vi "Main.vi"() -> ()   [LabVIEW 2015]
doc: "This template is for the Queued Message Handler design pattern.\n\nThe Event Handling Loop generates messages based on user interface actions.\n\nThe Message Handling Loop processes messages generated by the Event Handling Loop, or by other messages. The messages are string values, so new messages can be added easily to the Message Cases case structure in the Message Handling Loop. Each message cluster can also provide an optional value for Message Data, which is a variant that can be converted to whatever message-specific data is required."
uses:
  <vilib>/Utility/miscctls.llb/LV3DPointTypeDef.ctl
  <vilib>/Utility/miscctls.llb/LVRGBAColorTypeDef.ctl
  processedObjectInfo.ctl
  controls/UI Data.ctl
  controls/scanInstrumentInfo.ctl
  controls/Equip_Data.ctl
  controls/startScanData.ctl
  <vilib>/addons/h5labview2/base/hid_t.ctl
  controls/relativeMoveData.ctl
  controls/pBotMessageData.ctl
  controls/currentInfoData.ctl
  <vilib>/addons/h5labview2/file/H5Fmode.ctl
  controls/_acquireScanData_currentState.ctl
  <vilib>/Utility/miscctls.llb/LVPoint32TypeDef.ctl
  <vilib>/Utility/miscctls.llb/LVPointTypeDef.ctl
  <vilib>/Utility/miscctls.llb/LVPositionTypeDef.ctl
  <vilib>/Instr/_visa.llb/VISA Find Search Mode.ctl
  <vilib>/event_ctls.llb/usereventprio.ctl
  support/Message Queue/Enqueue Message (Single).vi
  <vilib>/Instr/_visa.llb/VISA Configure Serial Port (Instr).vi
  <vilib>/addons/h5labview2/base/lib_path.vi
  <vilib>/addons/h5labview2/base/H5Equery.vi
  <vilib>/Utility/error.llb/Error Cluster From Error Code.vi
  <userlib>/_MGI/Application Control/MGI Disable Enum/MGI Disable Enum (Grayed).vi
  <userlib>/_MGI/Application Control/MGI Disable Enum/MGI Disable Enum (Enabled).vi
  flipYZdbl.vi
  flipYZsgl.vi
  <vilib>/Utility/file.llb/Write Delimited Spreadsheet (DBL).vi
  <vilib>/addons/h5labview2/attrib/H5Awrite.llb/H5Awrite.xnode
  <vilib>/addons/h5labview2/dataset/H5Dwrite.llb/H5Dwrite.xnode
  <vilib>/ErrorRing/Error Ring.xnode
  support/Message Queue/Message Queue.lvlib
  support/User Event - Stop/User Event - Stop.lvlib
  <vilib>/picture/3D Picture Control/NI_3D Picture Control.lvlib
  <vilib>/addons/h5labview2/file/H5F.lvlib
  <vilib>/addons/h5labview2/dataset/H5D.lvlib
  <instrlib>/Ocean Optics 2000 4000/Ocean Optics 2000 4000.lvlib
  <vilib>/addons/h5labview2/space/H5S.lvlib
panel:
  out "textColorGray":u32(colorbox)=9174826
  out "textColorRed":u32(colorbox)=9174826
  out "textColorGreen":u32(colorbox)=9174826
  in  "pBot_timeSinceXHome":dbl
  in  "pBot_timeSinceYHome":dbl
  out "emptyObj":T1
  in  "objCol_sel":T2={"Red"=0.0, "Green"=1.0, "Blue"=0.0, "Alpha"=1.0}
  in  "objCol_deSel":T2={"Red"=0.0, "Green"=1.0, "Blue"=0.0, "Alpha"=1.0}
  out "PickPoint":T3
  in  "numberOfCommandLines":i32=50
  in  "cB_dataView":bool
  in  "cB_3Dview":bool
  in  "cB_USB2000+":bool
  in  "cB_plasmaBot":bool
  in  "controlTab":T4(tab)
  in  "pBot_ExperimentTabControl":enum32{"Scan", "Simple Exposure"}(tab)
  in  "pBot_scanNz":u16
  in  "pBot_scanNy":u16
  in  "pBot_scanNx":u16
  in  "pBot_scanningZmax":sgl min=0 step=0.1
  in  "pBot_scanningZmin":sgl caption="Z" min=0 step=0.1
  in  "pBot_scanningYmax":sgl min=0 step=0.1
  in  "pBot_scanningYmin":sgl caption="Y" min=0 step=0.1
  in  "pBot_scanningXmax":sgl min=0 step=0.1
  in  "pBot_scanningXmin":sgl caption="X" min=0 step=0.1
  in  "pBot_scanInstrument":string(combo) caption="Data instrument"
  in  "pBot_runScan":bool
  in  "pBot_yBack1":bool
  in  "pBot_yBack01":bool
  in  "pBot_yBack10":bool
  in  "pBot_xHome":bool
  in  "pBot_xRight1":bool
  in  "pBot_xRight01":bool
  in  "pBot_xRight10":bool
  in  "pBot_xLeft1":bool
  in  "pBot_xLeft10":bool
  in  "pBot_xLeft01":bool
  out "pBot_xyMoveDisplay":string
  in  "pBot_yForward1":bool
  in  "pBot_yForward10":bool
  in  "pBot_yForward01":bool
  in  "pBot_yHome":bool
  in  "pBot_zHome":bool
  out "pBot_zMoveDisplay":string
  in  "pBot_zUp1":bool
  in  "pBot_zUp01":bool
  in  "pBot_zUp10":bool
  in  "pBot_zDown1":bool
  in  "pBot_zDown10":bool
  in  "pBot_zDown01":bool
  in  "pBot_sendCommand":bool
  in  "pBot_gcodeCommand":string caption="G-code command"
  in  "pBot_ConnectButton":bool
  in  "pBot_VISAstrings":string(combo) caption="printrBot Port"
  in  "usb2000p_continuous?":bool caption="Continuous?"
  in  "usb2000p_saveSpectra":bool caption="usb2000p_ConnectButton"
  in  "usb2000p_aquireSpectra":bool caption="usb2000p_ConnectButton"
  in  "usb2000p_ConnectButton":bool
  in  "usb2000p_VISAstrings":string(combo) caption="USB2000+ Port"
  in  "usb2000p_intTime":u32=1000 caption="Integration Time (ms):"
  in  "cB_getObjectInfo":bool caption="Object Information:"
  in  "cB_rotate":bool
  in  "cB_translateDown":bool caption="cB_translateUp"
  in  "cB_translateUp":bool
  in  "cB_translateRight":bool
  in  "cB_translateLeft":bool
  in  "cB_translateForward":bool
  in  "cB_translateBack":bool caption="cB_translateUp"
  in  "cB_revertToActualPos":bool
  in  "cB_visualizeYtrans":dbl(knob) caption="Y" min=0.0 max=150.0 scale=0.0..150.0
  in  "cB_visualizeXtrans":dbl(knob) caption="X" min=0.0 max=285.0 scale=0.0..285.0
  in  "cB_visualizeZtrans":dbl(knob) caption="Z" min=0.0 max=150.0 scale=0.0..150.0
  in  "cB_addObject":bool
  in  "availibleObjectNames":string(combo) caption="Objects availible to add"
  in  "cB_toggleView":bool
  out "cB_realTimeInfoT2":string caption=", T2="
  out "cB_realTimeInfoT1":string caption=", T1="
  out "cB_realTimeInfoZ":string caption=", Z="
  out "cB_realTimeInfoY":string caption=",Y="
  out "cB_realTimeInfoX":string caption="X="
  out "1DdataGraph":cluster{dbl[], dbl[]}(graph)
  out "3D Picture":refnum<vi>(3d-picture)
  out "cB_commandLog":string
  # "(escape to quit  for now)"
  # "Configure the instrument first!!"
  # "Region"
  # "# of points"
  # ":"
  # ":"
  # ":"
  # "Y"
  # "X"
  # "Z"
  # "Use toggleView in the top right to switch between viewing spectra and the  3Dscene."
  # "Translate, rotate, get info of object\n(right click to select)"
  # "Use below knobs to visualize a\ntranslation without actually moving"
  # "dataView"
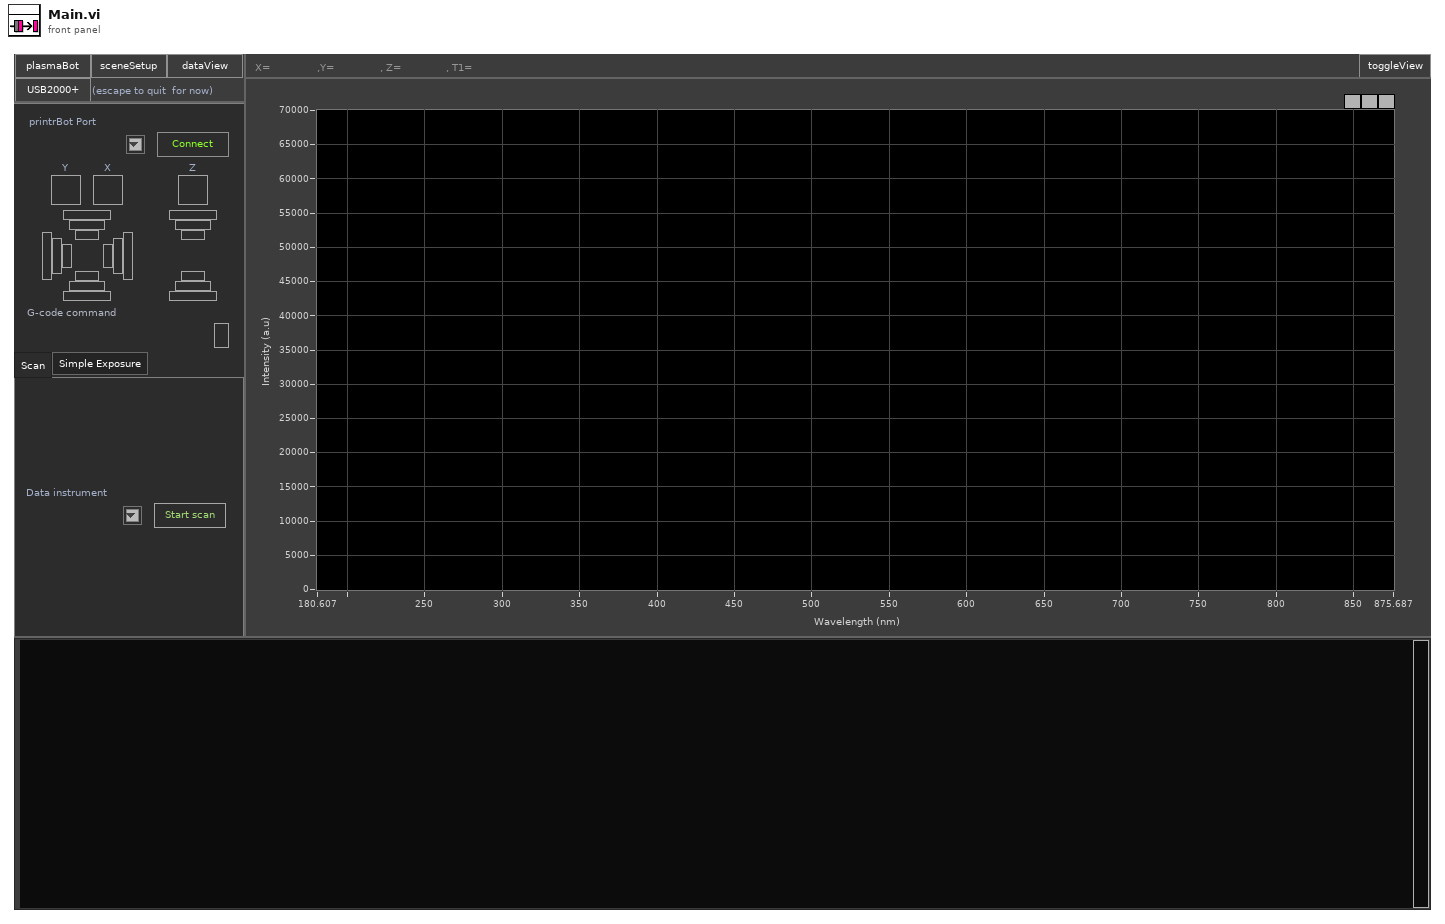
[diagram p1: front panel]
types:
  T1 = typedef "processedObjectInfo.ctl" = cluster{"Name":string, "objectFiles":cluster{"Location":path, "Color":cluster{"R":dbl, "G":dbl, "B":dbl, "A":dbl}}[], "center":cluster{"X":dbl, "Y":dbl, "Z":dbl}, "extent":cluster{"X":dbl, "Y":dbl, "Z":dbl}, "allowedMotion":enum16{"XY", "Z"}, "mountOn":enum16{"yArm", "breadBoard"}, "Movements":cluster{"Type":enum16{"rr", "ra", "tr", "ta"}, "vector":cluster{"X":dbl, "Y":dbl, "Z":dbl}, "scalar":dbl}[], "extraInfo":cluster{"parameter":string, "dataType":string, "vector":cluster{"X":dbl, "Y":dbl, "Z":dbl}, "scalar":dbl}[], "hasPOI?":bool, "POI":cluster{"X":dbl, "Y":dbl, "Z":dbl}, "posOffset":cluster{"X":dbl, "Y":dbl, "Z":dbl}, "referenceNum":refnum<vi>}
  T2 = typedef "LVRGBAColorTypeDef.ctl" = cluster{"Red":sgl, "Green":sgl, "Blue":sgl, "Alpha":sgl}
  T3 = typedef "LV3DPointTypeDef.ctl" = cluster{"X":sgl, "Y":sgl, "Z":sgl}
  T4 = enum32{"plasmaBot", "USB2000+", "3DView", "dataView"}
  T5 = typedef "Equip_Data.ctl" = cluster{"travelRange":T3, "yPOI_0":T3, "yPOI":T3, "pBot_VISA":refnum<visa-resource-name>, "pBotConnected?":bool, "disconnectPBot_Event":refnum<user-event>, "scanData":T6, "scanIndex":cluster{"X":u16, "Y":u16, "Z":u16}, "scanIncrementDir":cluster{"xFwd?":i16, "yFwd?":i16, "zFwd?":i16}, "scanSpeed":u16, "instrDataPage":u16[][][][], "instrDataPageSize":i32[], "h5File_refOut":T8, "ish5FileOpen?":bool, "h5File_dsetOut":T8, "h5FileError":errorcluster, "totalSteps":u32, "currentStep":u32, "USB2000p_Info":T7, "integrationTime":u32, "scan?":bool, "pBot_currentEEPROMsettings":string}
  T6 = typedef "startScanData.ctl" = cluster{"dataFilePath":path, "scanPoints":cluster{"dim1":sgl[], "dim2":sgl[], "dim3":sgl[]}, "N":cluster{"X":u16, "Y":u16, "Z":u16}, "scanInstrumentInfo":T7}
  T7 = typedef "scanInstrumentInfo.ctl" = cluster{"Name":string, "VISAname":refnum<visa-resource-name>, "1D_dataArraySize":u16, "extraInfo":variant, "error":errorcluster}
  T8 = typedef "hid_t.ctl" = i32
  T9 = typedef "UI Data.ctl" = cluster{"controlTabState":bool[], "pathToSTLFiles":path, "availableObjs":T1[], "objectNames":string[], "addedObjs":T1[], "selectedObj":T1, "3DPictureObjRef":refnum<vi>, "yPOI_0":cluster{"X":dbl, "Y":dbl, "Z":dbl}, "yPOI":cluster{"X":dbl, "Y":dbl, "Z":dbl}, "yPOI_Added?":bool, "breadBoard_00":cluster{"X":dbl, "Y":dbl, "Z":dbl}, "breadBoardOriginOffset":cluster{"X":dbl, "Y":dbl, "Z":dbl}, "XYtranslateObjControls":refnum<vi>[], "ZtranslateObjControls":refnum<vi>[], "pBot_controls":refnum<vi>[], "pBot_VISA":refnum<visa-resource-name>, "commandLog":string, "pBotConnected?":bool, "pBot_currentEEPROMsettings":string, "realTimeInfoControls":refnum<vi>[], "pBot_tempSensor1":dbl, "pBot_tempSensor2":dbl, "realTimeInfoTextColor":u32[], "disconnectPBot_Event":refnum<user-event>, "needToHomeY?":bool, "pBot_relativePositioning":bool, "pBot_minPos":cluster{"X":dbl, "Y":dbl, "Z":dbl}, "pBot_maxPos":cluster{"X":dbl, "Y":dbl, "Z":dbl}, "pBot_homeOffset":cluster{"X":dbl, "Y":dbl, "Z":dbl}, "textColorGreen":u32, "textColorRed":u32, "textColorGray":u32, "transVisualizationControls":refnum<vi>[], "needToHomeXY?":bool, "pBot_minScanRegion":cluster{"X":sgl, "Y":sgl, "Z":sgl}, "pBot_maxScanRegion":cluster{"X":sgl, "Y":sgl, "Z":sgl}, "pBot_scanN":cluster{"X":u16, "Y":u16, "Z":u16}, "connectedInstruments":T7[], "isScanning?":bool, "Wavelengths":dbl[], "usb2000p_controlRefs":refnum<vi>[], "3DPictureRef":refnum<vi>}
  T10 = typedef "Message Queue.lvlib/All Message Queues.ctl" = cluster{"UI":refnum<queue>, "equipment":refnum<queue>}
  T11 = cluster{"Message":string, "error constant":errorcluster, "disconnectPBot_Event":refnum<user-event>}
  T12 = typedef "relativeMoveData.ctl" = cluster{"Direction":enum16{"Y", "X", "Z"}, "Amount":dbl}
  T13 = typedef "eventvkey.ctl" = enum16{"ASCII", "Enter", "Return", "Shift", "Ctrl", "Alt", "Cmd", "Opt", "Caps", "NumLock", "Clear", "Break", "Up", "Down", "Left", "Right", "Insert", "Delete", "Home", "End", "PageUp", "PageDown", "Escape", "Help", "Pause", "ScrollLock", "F1", "F2", "F3", "F4", "F5", "F6", "F7", "F8", "F9", "F10", "F11", "F12", "F13", "F14", "F15", "F16", "F17", "F18", "F19", "F20", "F21", "F22", "F23", "F24", "Play", "VolumeUp", "VolumeDown", "Mute", "Two Byte Char"}
  T14 = typedef "LVPoint32TypeDef.ctl" = cluster{"Horizontal":i32, "Vertical":i32}
  T15 = typedef "pBotMessageData.ctl" = cluster{"commandID":string, "gCode":string, "extraInfo":string, "originatingCommandID":string, "error":errorcluster}
  T16 = typedef "currentInfoData.ctl" = cluster{"currentPos":cluster{"X":dbl, "Y":dbl, "Z":dbl}, "temperature":dbl, "error constant":errorcluster}
  T17 = typedef "H5F.lvlib/H5Fmode.ctl" = enum16{"read-only", "read-write", "overwrite", "create new", "open or create"}
  T18 = typedef "_acquireScanData_currentState.ctl" = cluster{"scanIndex":cluster{"X":u16, "Y":u16, "Z":u16}, "scanFinished?":bool, "savePageData?":bool}
  T19 = cluster{"dim1":sgl[], "dim2":sgl[], "dim3":sgl[]}
  T20 = cluster{"cB_visualizeXtrans":dbl, "cB_visualizeZtrans":dbl, "cB_visualizeYtrans":dbl}
  T21 = cluster{"cB_visualizeXtrans":dbl, "cB_visualizeYtrans":dbl, "cB_visualizeZtrans":dbl}
  T22 = enum8{"Enabled", "Disabled", "Disabled and Grayed Out"}
  T23 = typedef "LVPositionTypeDef.ctl" = cluster{"Left":i32, "Top":i32}
  T24 = typedef "LVPointTypeDef.ctl" = cluster{"Horizontal":i16, "Vertical":i16}
  T25 = enum16{"None", "Spherical", "Flying", "Oriented"}
  T26 = typedef "usereventprio.ctl" = enum32{"high priority", "normal priority"}
  T27 = typedef "LVRectTypeDef.ctl" = cluster{"Left":i16, "Top":i16, "Right":i16, "Bottom":i16}
  T28 = typedef "VISA Find Search Mode.ctl" = u32
  T29 = cluster{"Wavelengths":dbl[], "Spectrum by Pixels":dbl[]}
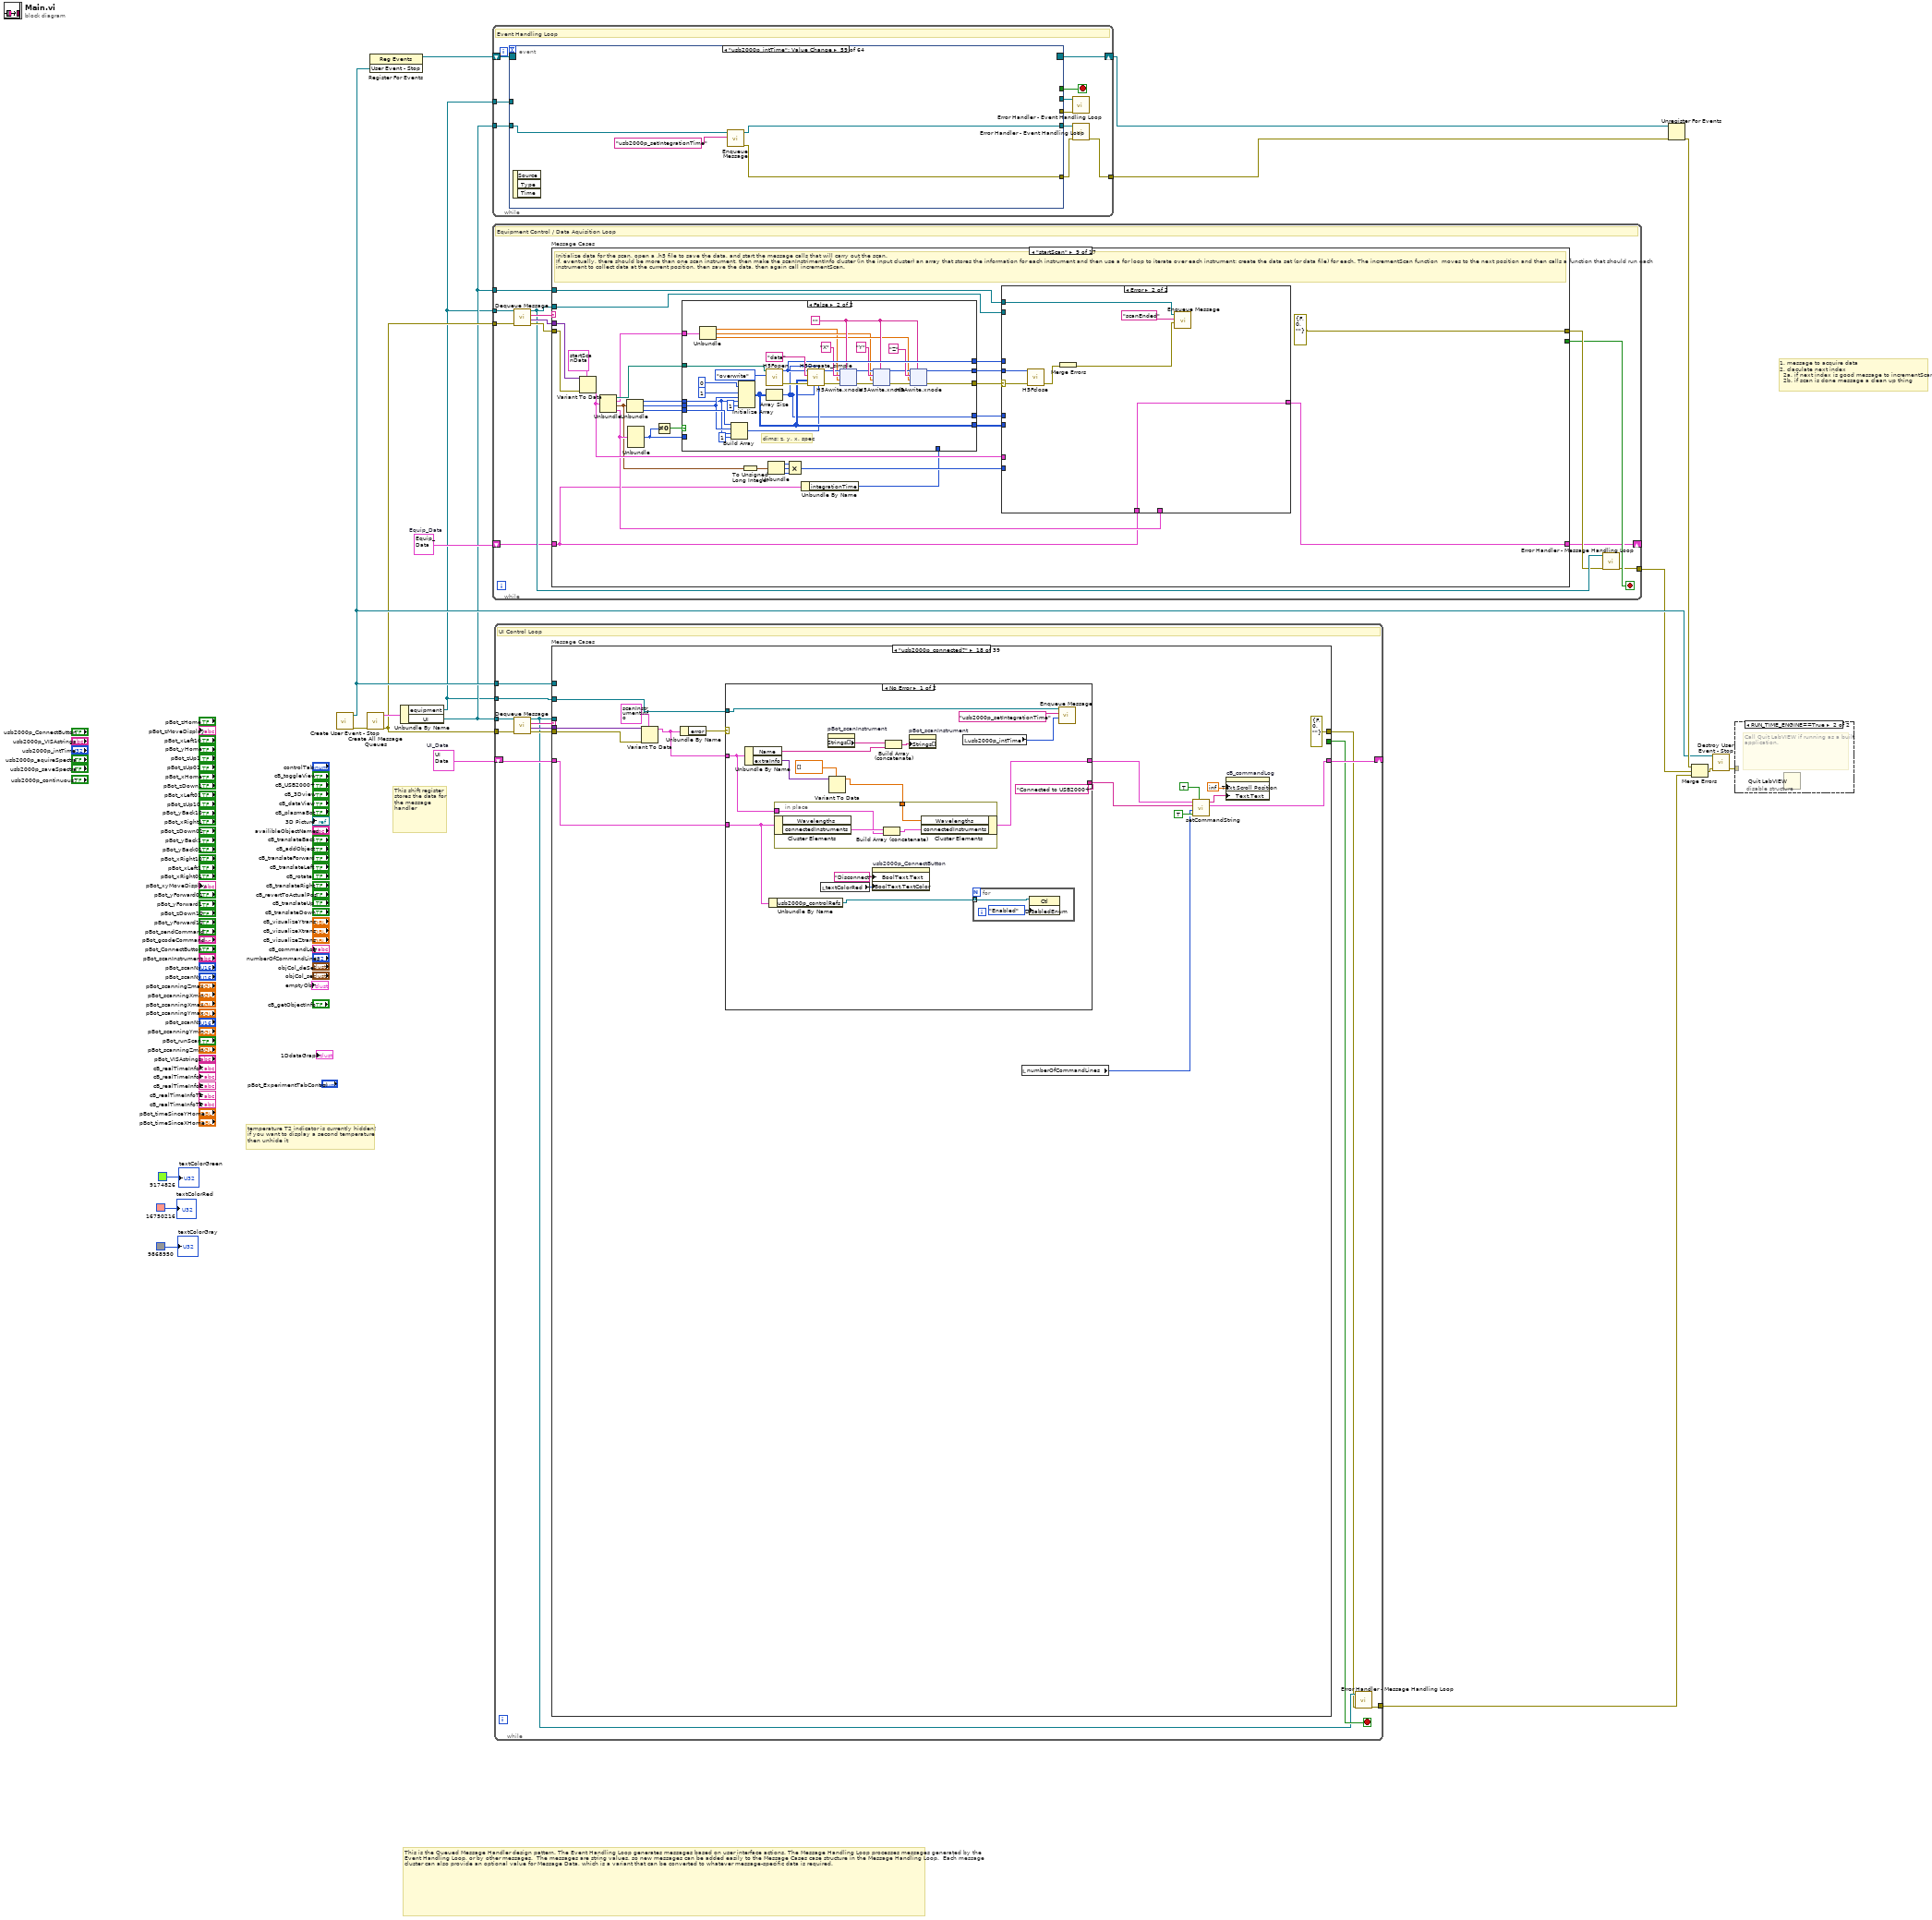
[diagram p0: block diagram]
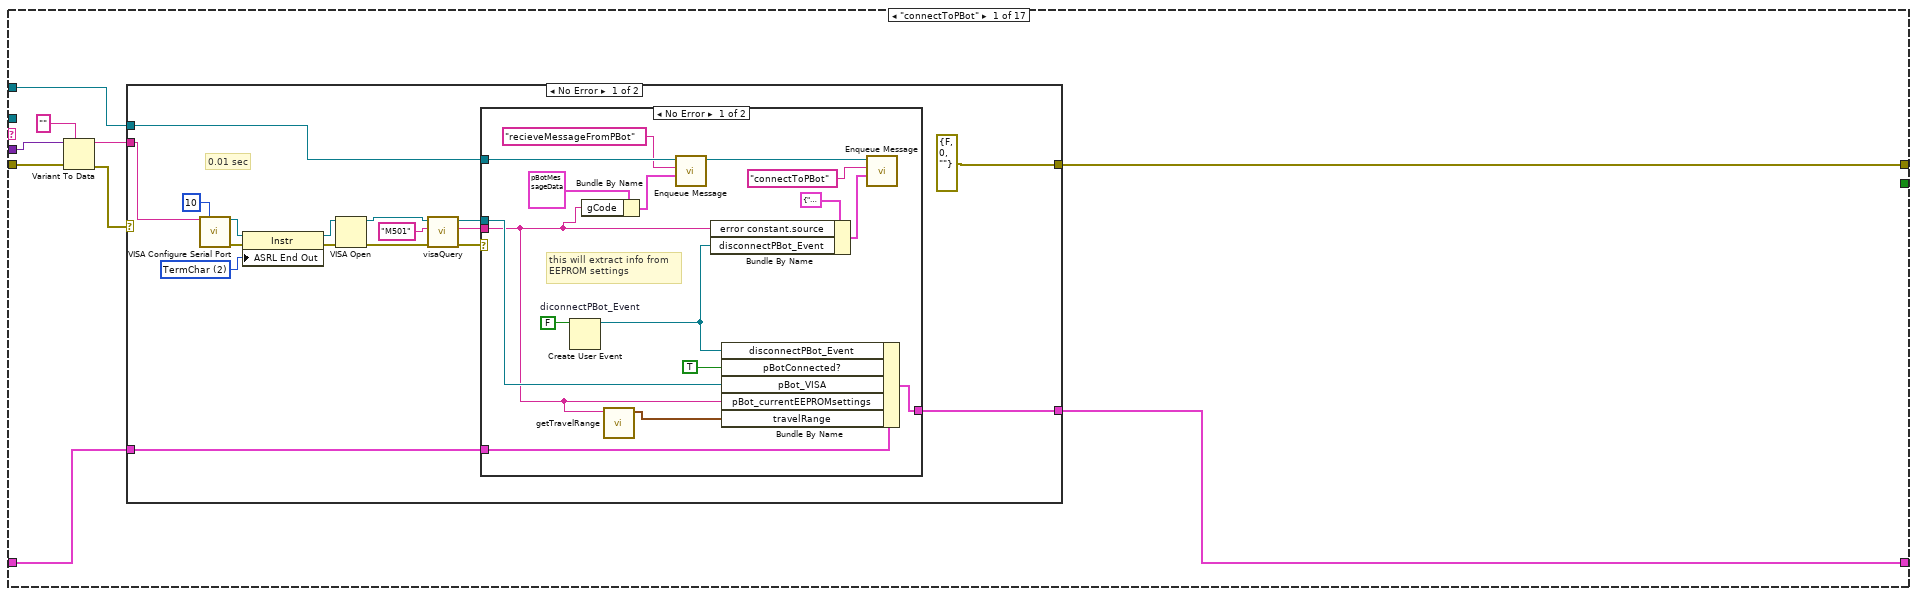
[diagram p2: hidden frame]
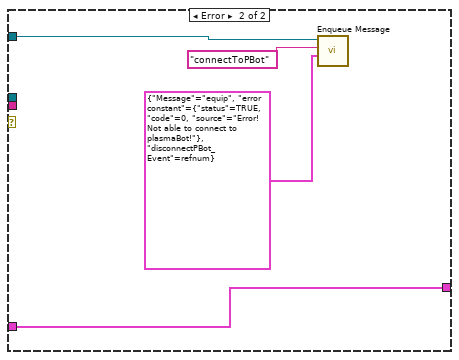
[diagram p3: hidden frame]
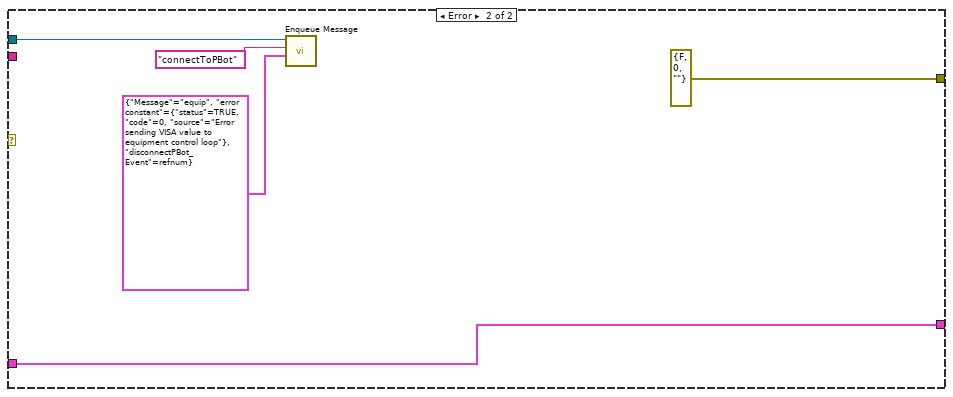
[diagram p4: hidden frame]
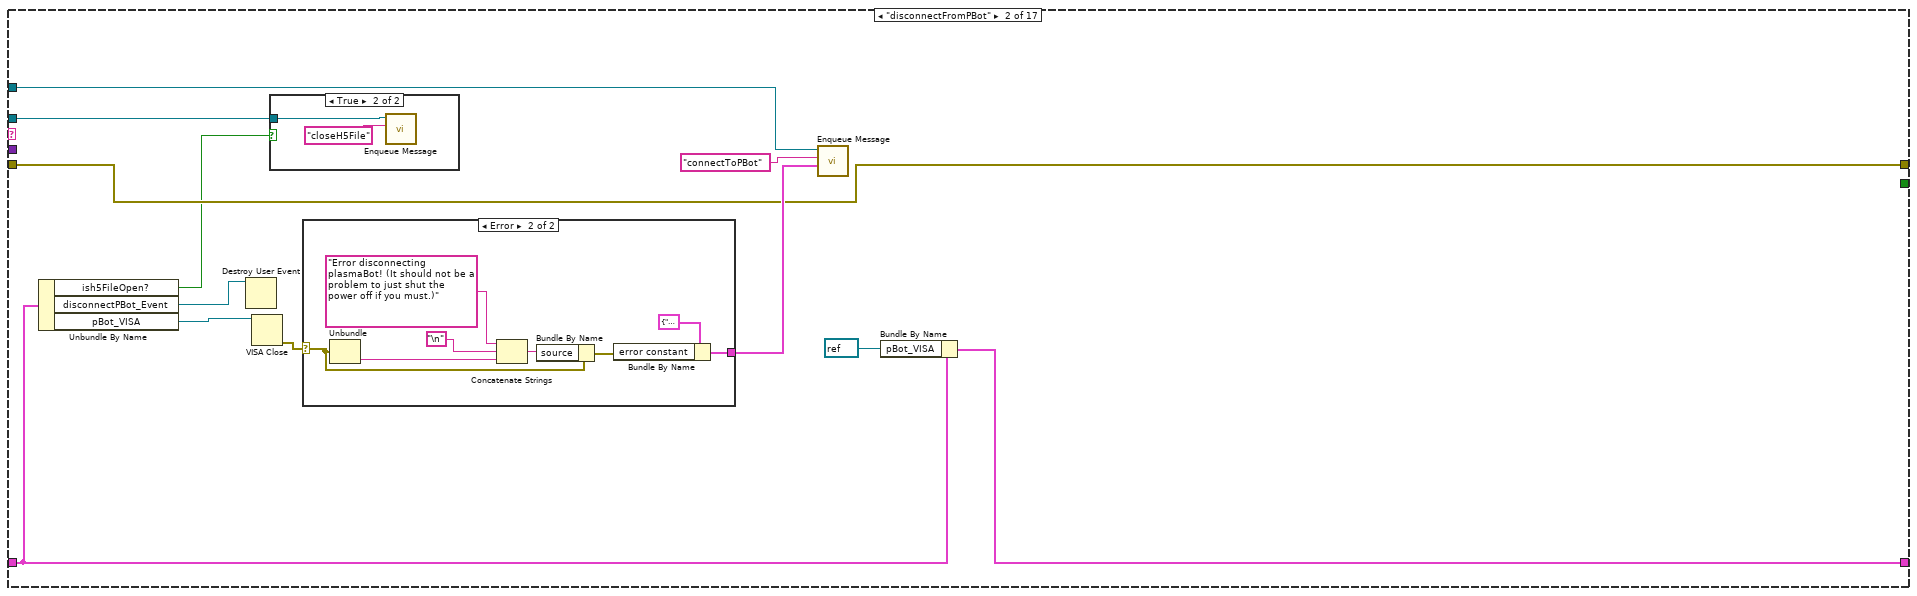
[diagram p5: hidden frame]
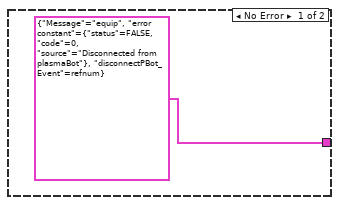
[diagram p7: hidden frame]
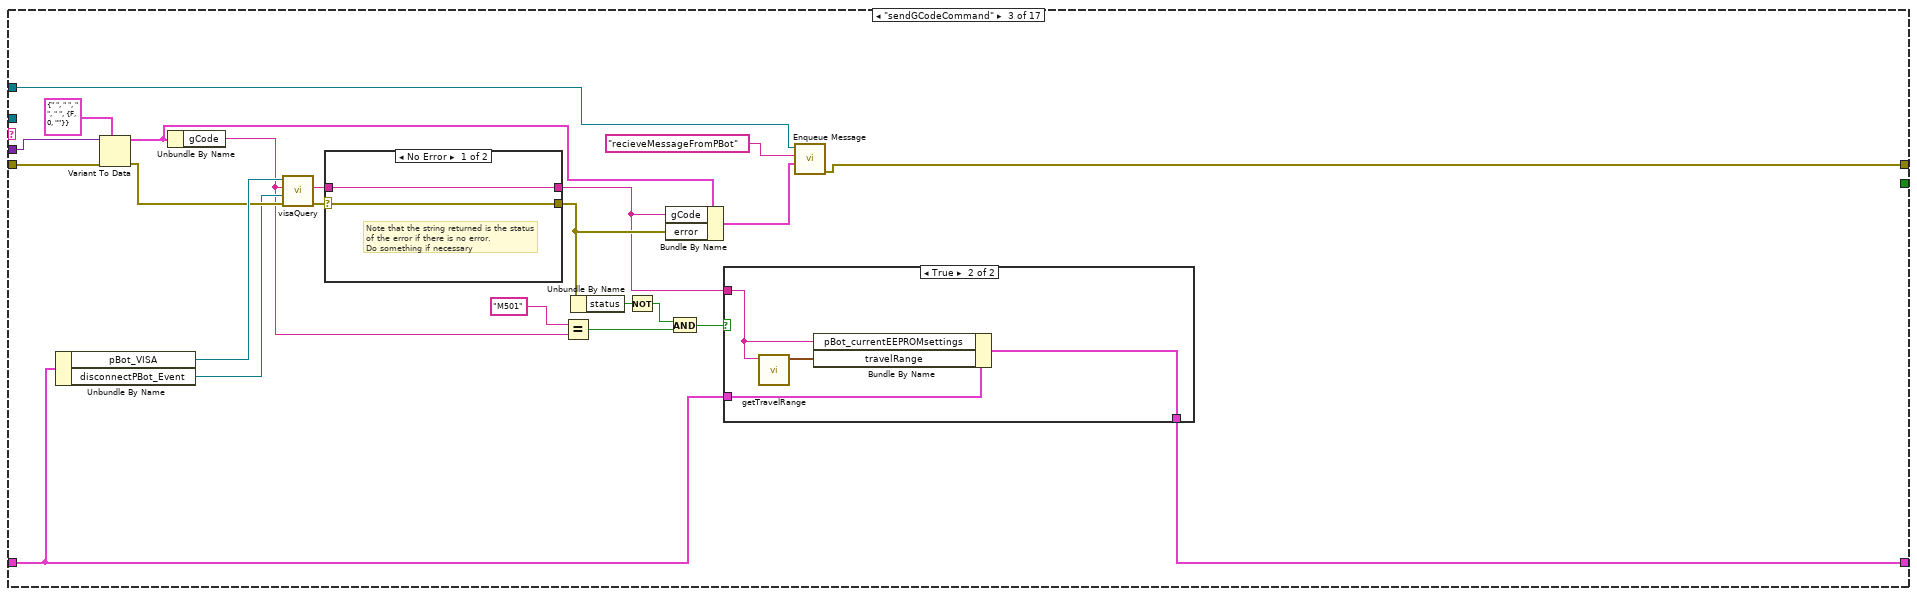
[diagram p8: hidden frame]
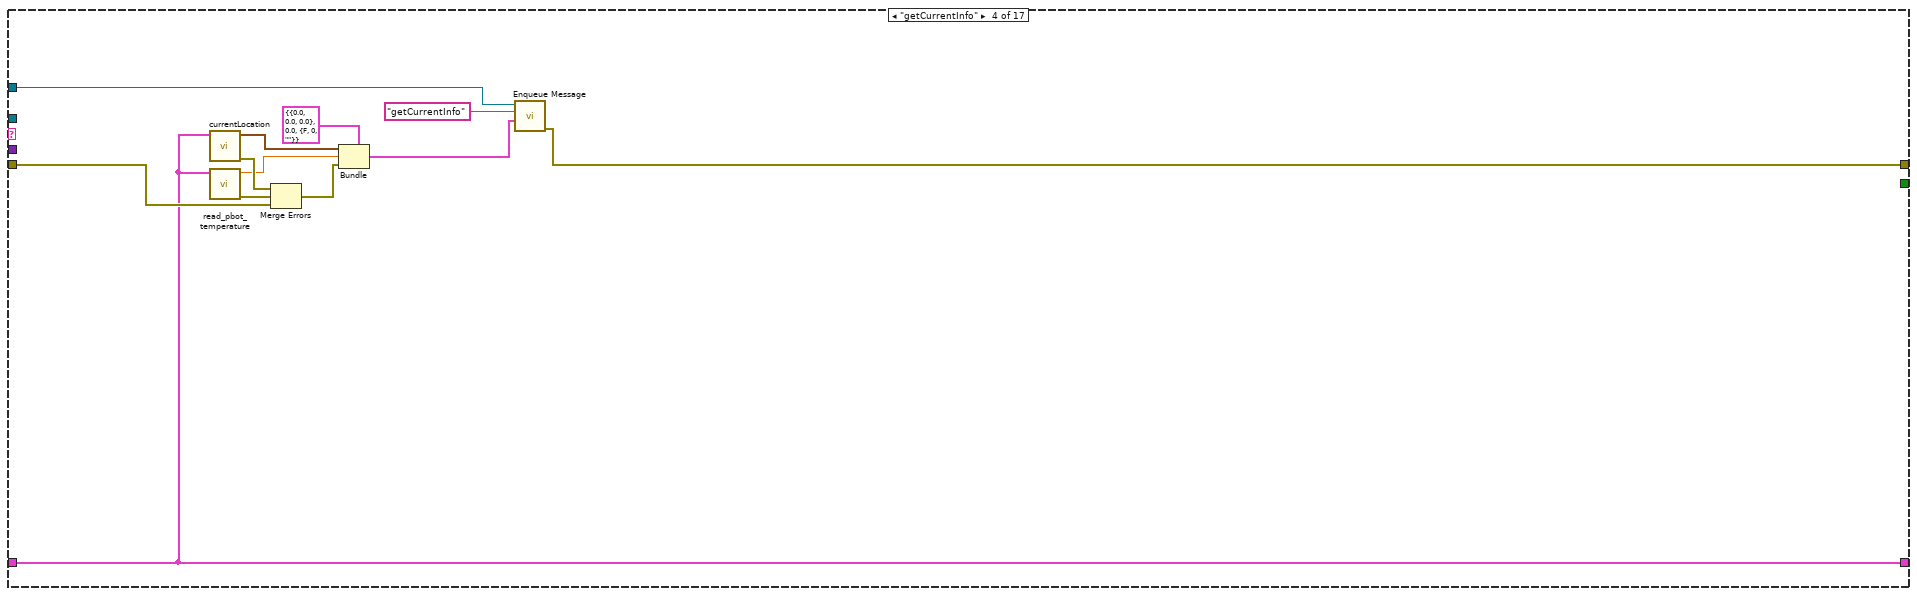
[diagram p11: hidden frame]
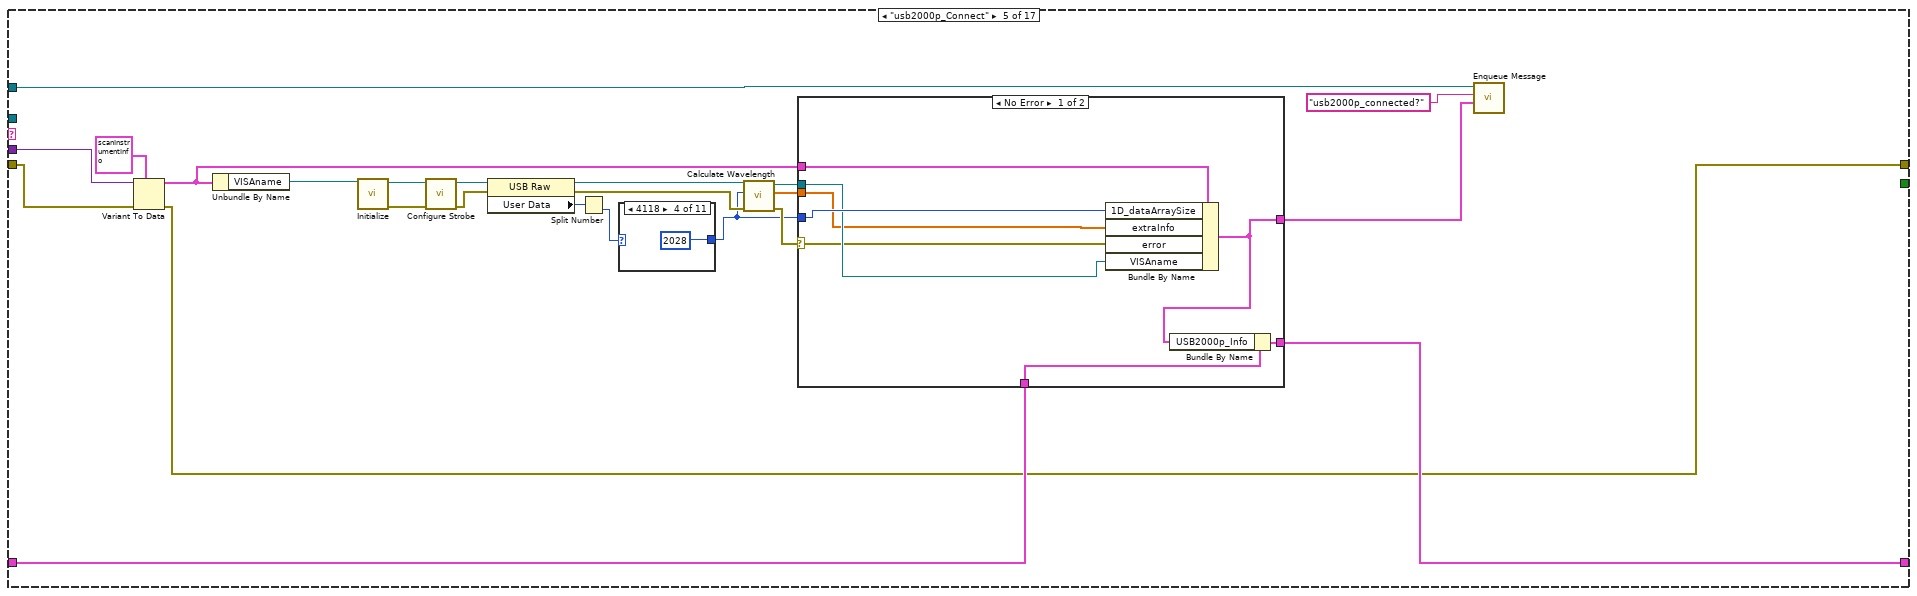
[diagram p12: hidden frame]
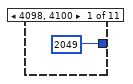
[diagram p13: hidden frame]
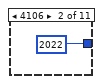
[diagram p14: hidden frame]
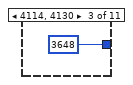
[diagram p15: hidden frame]
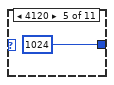
[diagram p16: hidden frame]
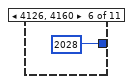
[diagram p17: hidden frame]
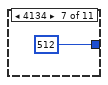
[diagram p18: hidden frame]
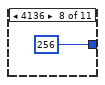
[diagram p19: hidden frame]
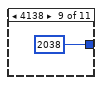
[diagram p20: hidden frame]
diagram:
  w4 = T5 {"travelRange"={"X"=0.0, "Y"=0.0, "Z"=0.0}, "yPOI_0"={"X"=0.0, "Y"=0.0, "Z"=0.0}, "yPOI"={"X"=0.0, "Y"=0.0, "Z"=0.0}, "pBot_VISA"="", "pBotConnected?"=FALSE, "disconnectPBot_Event"=refnum, "scanData"={"dataFilePath"=path "", "scanPoints"={"dim1"=[], "dim2"=[], "dim3"=[]}, "N"={"X"=0, "Y"=0, "Z"=0}, "scanInstrumentInfo"={"Name"="", "VISAname"="", "1D_dataArraySize"=0, "extraInfo"=variant, "error"={"status"=FALSE, "code"=0, "source"=""}}}, "scanIndex"={"X"=0, "Y"=0, "Z"=0}, "scanIncrementDir"={"xFwd?"=0, "yFwd?"=0, "zFwd?"=0}, "scanSpeed"=0, "instrDataPage"=[], "instrDataPageSize"=[], "h5File_refOut"=0, "ish5FileOpen?"=FALSE, "h5File_dsetOut"=0, "h5FileError"={"status"=FALSE, "code"=0, "source"=""}, "totalSteps"=0, "currentStep"=0, "USB2000p_Info"={"Name"="", "VISAname"="", "1D_dataArraySize"=0, "extraInfo"=variant, "error"={"status"=FALSE, "code"=0, "source"=""}}, "integrationTime"=0, "scan?"=FALSE, "pBot_currentEEPROMsettings"=""}  # Equip_Data
  w14 = T9 {"controlTabState"=[], "pathToSTLFiles"=path "", "availableObjs"=[], "objectNames"=[], "addedObjs"=[], "selectedObj"={"Name"="", "objectFiles"=[], "center"={"X"=0.0, "Y"=0.0, "Z"=0.0}, "extent"={"X"=0.0, "Y"=0.0, "Z"=0.0}, "allowedMotion"=enum."XY", "mountOn"=enum."yArm", "Movements"=[], "extraInfo"=[], "hasPOI?"=FALSE, "POI"={"X"=0.0, "Y"=0.0, "Z"=0.0}, "posOffset"={"X"=0.0, "Y"=0.0, "Z"=0.0}, "referenceNum"=refnum}, "3DPictureObjRef"=refnum, "yPOI_0"={"X"=0.0, "Y"=0.0, "Z"=0.0}, "yPOI"={"X"=0.0, "Y"=0.0, "Z"=0.0}, "yPOI_Added?"=FALSE, "breadBoard_00"={"X"=0.0, "Y"=0.0, "Z"=0.0}, "breadBoardOriginOffset"={"X"=0.0, "Y"=0.0, "Z"=0.0}, "XYtranslateObjControls"=[], "ZtranslateObjControls"=[], "pBot_controls"=[], "pBot_VISA"="", "commandLog"="", "pBotConnected?"=FALSE, "pBot_currentEEPROMsettings"="", "realTimeInfoControls"=[], "pBot_tempSensor1"=0.0, "pBot_tempSensor2"=0.0, "realTimeInfoTextColor"=[], "disconnectPBot_Event"=refnum, "needToHomeY?"=FALSE, "pBot_relativePositioning"=FALSE, "pBot_minPos"={"X"=0.0, "Y"=0.0, "Z"=0.0}, "pBot_maxPos"={"X"=0.0, "Y"=0.0, "Z"=0.0}, "pBot_homeOffset"={"X"=0.0, "Y"=0.0, "Z"=0.0}, "textColorGreen"=9174826, "textColorRed"=16750216, "textColorGray"=9868950, "transVisualizationControls"=[], "needToHomeXY?"=FALSE, "pBot_minScanRegion"={"X"=0.0, "Y"=0.0, "Z"=0.0}, "pBot_maxScanRegion"={"X"=0.0, "Y"=0.0, "Z"=0.0}, "pBot_scanN"={"X"=0, "Y"=0, "Z"=0}, "connectedInstruments"=[], "isScanning?"=FALSE, "Wavelengths"=[], "usb2000p_controlRefs"=[], "3DPictureRef"=refnum}  # UI_Data
  # "1. message to acquire data\n2. claculate next index\n  2a. if next index is good message to incrementScan\n  2b. if scan is done message a clean up thing"
  # "temperature T2 indicator is currently hidden!\nif you want to display a second temperature\nthen unhide it"
  # "This is the Queued Message Handler design pattern. The Event Handling Loop generates messages based on user interface actions. The Message Handling Loop processes messages generated by the Event Handling Loop, or by other messages.  The messages are string values, so new messages can be added easily to the Message Cases case structure in the Message Handling Loop.  Each message cluster can also provide an optional value for Message Data, which is a variant that can be converted to whatever message-specific data is required."
  # "This shift register stores the data for the message handler"
  n1 = call "Create User Event - Stop.vi"() -> ("error out"=w18:errorcluster, "User Event - Stop"=w10:refnum<user-event>)  [unwired: 10 in]
  n2 = call "Create All Message Queues.vi"("error in (no error)"=w18) -> ("error out"=w7:errorcluster, "Message Queues out"=w19:T10)  [unwired: 9 in]
  n3 = register-events(w10) -> (reference out=w11:refnum<event-registration>)  [unwired: 2 in, 1 out]
  n4 = Unbundle By Name(w19) -> ("equipment"=w2:refnum<queue>, "UI"=w3:refnum<queue>)
  n5 = while {
    tunnel: w3 -> [w29]
    shift-right: [w27] -> w15
    shift-left: w11 -> [w28]
    tunnel: [w23] -> w12
    tunnel: w2 -> [w22]
    stop <- w25 stop-if-true
    # "Event Handling Loop"
    n6 = event shown="[58] \"usb2000p_intTime\": Value Change" {
      selector: w28 -> [_ _ _ _ _ _ _ _ _ _ _ _ _ _ _ _ _ _ _ _ _ _ _ _ _ _ _ _ _ _ _ _ _ _ _ _ _ _ _ _ _ _ _ _ _ _ _ _ _ _ _ _ _ _ _ _ _ _ _ _ _ _ _ _]
      dyn-events: [_ _ _ _ _ _ _ _ _ _ _ _ _ _ _ _ _ _ _ _ _ _ _ _ _ _ _ _ _ _ _ _ _ _ _ _ _ _ _ _ _ _ _ _ _ _ _ _ _ _ _ _ _ _ _ _ _ _ _ _ _ _ _ _] -> w27
      timeout: _ -> [_ _ _ _ _ _ _ _ _ _ _ _ _ _ _ _ _ _ _ _ _ _ _ _ _ _ _ _ _ _ _ _ _ _ _ _ _ _ _ _ _ _ _ _ _ _ _ _ _ _ _ _ _ _ _ _ _ _ _ _ _ _ _ _]
      tunnel: [_ _ _ _ _ _ _ _ _ _ _ _ _ _ _ _ _ _ _ _ _ _ _ _ _ _ _ _ _ _ _ _ _ _ _ _ _ _ _ _ _ _ _ _ _ _ _ _ _ _ _ _ _ _ _ _ _ _ _ _ _ TRUE ("Discard?") _ _] -> w25
      tunnel: w29 -> [w33 w37 w41 w45 w49 w54 w59 w64 w69 w74 w79 w83 w90 w117 w120 w124 w132 w136 w140 w144 w149 w154 w159 w164 w169 w174 w179 w184 w189 w194 w199 w204 w209 w215 w220 w225 w231 w236 w241 w246 w251 w256 w261 w266 w271 w276 w281 w286 w291 w296 w301 w306 w311 w316 w319 w323 w328 w332 w336 w340 w344 w346 w351 w353]
      tunnel: [w31 w34 w38 w42 w46 w50 w55 w60 w65 w70 w75 w80 w87 _ _ _ _ _ w138 w142 w147 w152 w157 w162 w167 w172 w177 w182 w187 w192 w197 w202 w207 w213 w218 w223 w227 w232 w237 w242 w247 w252 w257 w262 w267 w272 w277 w282 w287 w292 w297 w302 w307 w312 w317 w321 w326 w330 w334 w338 w342 _ w350 _] -> w26
      tunnel: [w32 w36 w40 w44 w48 w53 w58 w63 w68 w73 w78 w82 w89 w116 w119 w123 w131 w135 w139 w143 w148 w153 w158 w163 w168 w173 w178 w183 w188 w193 w198 w203 w208 w214 w219 w224 w228 w233 w238 w243 w248 w253 w258 w263 w268 w273 w278 w283 w288 w293 w298 w303 w308 w313 w318 w322 w327 w331 w335 w339 w343 w346 w349 w353] -> w24
      tunnel: w22 -> [_ _ _ _ _ _ _ _ _ _ _ _ w86 _ _ _ _ _ _ _ _ _ _ _ _ _ _ _ _ _ _ _ _ _ _ _ _ _ _ _ _ _ _ _ _ _ _ _ _ _ _ _ _ _ _ _ _ _ _ _ _ _ _ _]
      tunnel: [_ _ _ _ _ _ _ _ _ _ _ _ w85 _ _ _ _ _ _ _ _ _ _ _ _ _ _ _ _ _ _ _ _ _ _ _ _ _ _ _ _ _ _ _ _ _ _ _ _ _ _ _ _ _ _ _ _ _ _ _ _ _ _ _] -> w21
      tunnel: [_ _ _ _ _ _ _ _ _ _ _ _ w84 _ _ _ _ _ _ _ _ _ _ _ _ _ _ _ _ _ _ _ _ _ _ _ _ _ _ _ _ _ _ _ _ _ _ _ _ _ _ _ _ _ _ _ _ _ _ _ _ _ _ _] -> w20
      event Pane Size {
        n7 = event-data() -> ()  [unwired: 1 in, 1 out]
        n8 = call-poly "Enqueue Message.vi"("Message"="updateDisplay", "Message Queue"=w33) -> ("error out"=w31:errorcluster, "dup Message Queue"=w32:refnum<queue>)  [unwired: 8 in]
      }
      event "cB_dataView", "cB_3Dview", "cB_USB2000+", "cB_plasmaBot": Value Change {
        n9 = event-data() -> ()  [unwired: 1 in, 6 out]
        n10 = call-poly "Enqueue Message.vi"("Message"="changeControlTab", "Message Queue"=w37) -> ("error out"=w34:errorcluster, "dup Message Queue"=w36:refnum<queue>)  [unwired: 8 in]
      }
      event "cB_toggleView": Value Change {
        n11 = event-data() -> ()  [unwired: 1 in, 6 out]
        n12 = call-poly "Enqueue Message.vi"("Message"="toggleView", "Message Queue"=w41) -> ("error out"=w38:errorcluster, "dup Message Queue"=w40:refnum<queue>)  [unwired: 8 in]
      }
      event "cB_addObject": Value Change {
        n13 = event-data() -> ()  [unwired: 1 in, 1 out]
        n14 = call-poly "Enqueue Message.vi"("Message"="addObject", "Message Queue"=w45) -> ("error out"=w42:errorcluster, "dup Message Queue"=w44:refnum<queue>)  [unwired: 8 in]
      }
      event "cB_rotate": Value Change {
        n15 = event-data() -> ()  [unwired: 1 in, 1 out]
        n16 = call-poly "Enqueue Message.vi"("Message"="rotateObject", "Message Queue"=w49) -> ("error out"=w46:errorcluster, "dup Message Queue"=w48:refnum<queue>)  [unwired: 8 in]
      }
      event "cB_translateBack": Value Change {
        n17 = event-data() -> ()  [unwired: 1 in, 2 out]
        n18 = call-poly "Enqueue Message.vi"("Message Data"=cluster{"X":dbl, "Y":dbl, "Z":dbl} {"X"=0.0, "Y"=0.0, "Z"=-25.4} ("currentCenter"), "Message"="translateObj", "Message Queue"=w54) -> ("error out"=w50:errorcluster, "dup Message Queue"=w53:refnum<queue>)  [unwired: 7 in]
      }
      event "cB_translateForward": Value Change {
        n19 = event-data() -> ()  [unwired: 1 in, 2 out]
        n20 = call-poly "Enqueue Message.vi"("Message Data"=cluster{"X":dbl, "Y":dbl, "Z":dbl} {"X"=0.0, "Y"=0.0, "Z"=25.4} ("currentCenter"), "Message"="translateObj", "Message Queue"=w59) -> ("error out"=w55:errorcluster, "dup Message Queue"=w58:refnum<queue>)  [unwired: 7 in]
      }
      event "cB_translateRight": Value Change {
        n21 = event-data() -> ()  [unwired: 1 in, 2 out]
        n22 = call-poly "Enqueue Message.vi"("Message Data"=cluster{"X":dbl, "Y":dbl, "Z":dbl} {"X"=25.4, "Y"=0.0, "Z"=0.0} ("currentCenter"), "Message"="translateObj", "Message Queue"=w64) -> ("error out"=w60:errorcluster, "dup Message Queue"=w63:refnum<queue>)  [unwired: 7 in]
      }
      event "cB_translateLeft": Value Change {
        n23 = event-data() -> ()  [unwired: 1 in, 2 out]
        n24 = call-poly "Enqueue Message.vi"("Message Data"=cluster{"X":dbl, "Y":dbl, "Z":dbl} {"X"=-25.4, "Y"=0.0, "Z"=0.0} ("currentCenter"), "Message"="translateObj", "Message Queue"=w69) -> ("error out"=w65:errorcluster, "dup Message Queue"=w68:refnum<queue>)  [unwired: 7 in]
      }
      event "cB_translateUp": Value Change {
        n25 = event-data() -> ()  [unwired: 1 in, 2 out]
        n26 = call-poly "Enqueue Message.vi"("Message Data"=cluster{"X":dbl, "Y":dbl, "Z":dbl} {"X"=0.0, "Y"=10.0, "Z"=0.0} ("currentCenter"), "Message"="translateObj", "Message Queue"=w74) -> ("error out"=w70:errorcluster, "dup Message Queue"=w73:refnum<queue>)  [unwired: 7 in]
      }
      event "cB_translateDown": Value Change {
        n27 = event-data() -> ()  [unwired: 1 in, 2 out]
        n28 = call-poly "Enqueue Message.vi"("Message Data"=cluster{"X":dbl, "Y":dbl, "Z":dbl} {"X"=0.0, "Y"=-10.0, "Z"=0.0} ("currentCenter"), "Message"="translateObj", "Message Queue"=w79) -> ("error out"=w75:errorcluster, "dup Message Queue"=w78:refnum<queue>)  [unwired: 7 in]
      }
      event "cB_getObjectInfo": Value Change {
        n29 = event-data() -> ()  [unwired: 1 in, 2 out]
        n30 = call-poly "Enqueue Message.vi"("Message"="getObjectInfo", "Message Queue"=w83) -> ("error out"=w80:errorcluster, "dup Message Queue"=w82:refnum<queue>)  [unwired: 8 in]
      }
      event Key Down {
        n31 = event-data() -> ("VKey"=w88:T13)  [unwired: 1 in]
        n32 = case shown="Default" w88 {
          tunnel: w90 -> [w94 w100 w106]
          tunnel: [w94 w99 w105] -> w89
          tunnel: [errorcluster {"status"=FALSE, "code"=0, "source"=""} ("error out") w97 w104] -> w87
          tunnel: w86 -> [w91 w96 w103]
          tunnel: [w91 w96 w102] -> w85
          tunnel: [errorcluster {"status"=FALSE, "code"=0, "source"=""} ("error out") errorcluster {"status"=FALSE, "code"=0, "source"=""} ("error out") errorcluster {"status"=FALSE, "code"=0, "source"=""} ("error out")] -> w84
          frame Default {
          }
          frame "Delete" {
            n33 = call-poly "Enqueue Message.vi"("Message"="deleteObject", "Message Queue"=w100) -> ("error out"=w97:errorcluster, "dup Message Queue"=w99:refnum<queue>)  [unwired: 8 in]
          }
          frame "Escape" {
            n34 = disable-structure shown="Enabled" {
              disable-tunnel: w106 -> [w110 w114]
              disable-tunnel: [w109 w114] -> w105
              disable-tunnel: [w108 errorcluster {"status"=FALSE, "code"=0, "source"=""} ("error out")] -> w104
              disable-tunnel: w103 -> [w107 _]
              disable-tunnel: [w107 _] -> w102
              frame Enabled {
                n35 = call-poly "Enqueue Message.vi"("Priority Message? (F)"=TRUE, "Message"="Confirm Quit", "Message Queue"=w110) -> ("error out"=w108:errorcluster, "dup Message Queue"=w109:refnum<queue>)  [unwired: 7 in]
              }
              frame Disabled {
              }
            }
          }
        }
      }
      event "cB_visualizeXtrans", "cB_visualizeZtrans", "cB_visualizeYtrans": Value Change {
        n36 = event-data() -> ()  [unwired: 1 in, 3 out]
        n37 = call-poly "Enqueue Message.vi"("Message"="visualizeTranslation", "Message Queue"=w117) -> ("dup Message Queue"=w116:refnum<queue>)  [unwired: 8 in, 1 out]
      }
      event "cB_revertToActualPos": Value Change {
        n38 = event-data() -> ()  [unwired: 1 in, 3 out]
        n39 = call-poly "Enqueue Message.vi"("Message"="revertToActualPos", "Message Queue"=w120) -> ("dup Message Queue"=w119:refnum<queue>)  [unwired: 8 in, 1 out]
      }
      event "3D Picture": Mouse Down {
        n40 = event-data() -> ("Button"=w121:u16, "Coords"=w122:T14)  [unwired: 1 in]
        n41 = case shown="2" w121 {
          tunnel: w124 -> [w125 w129]
          tunnel: [w125 w128] -> w123
          tunnel: w122 -> [_ w127]
          frame Default {
          }
          frame 2 {
            n42 = call-poly "Enqueue Message.vi"("Message Data"=w127, "Message"="selectObject", "Message Queue"=w129) -> ("dup Message Queue"=w128:refnum<queue>)  [unwired: 7 in, 1 out]
          }
        }
      }
      event "pBot_VISAstrings": Mouse Down? {
        n43 = event-data() -> ()  [unwired: 1 in, 3 out]
        n44 = call-poly "Enqueue Message.vi"("Message"="pBot_getInstruments" ("expression (\"?*\")"), "Message Queue"=w132) -> ("dup Message Queue"=w131:refnum<queue>)  [unwired: 8 in, 1 out]
        n45 = event-data() -> ()  [unwired: 2 in, 1 out]
      }
      event "pBot_ConnectButton": Value Change {
        n46 = event-data() -> ()  [unwired: 1 in, 3 out]
        n47 = call-poly "Enqueue Message.vi"("Message Data"=T11 {"Message"="event", "error constant"={"status"=FALSE, "code"=0, "source"=""}, "disconnectPBot_Event"=refnum}, "Message"="connectToPBot", "Message Queue"=w136) -> ("dup Message Queue"=w135:refnum<queue>)  [unwired: 7 in, 1 out]
      }
      event "pBot_sendCommand": Value Change {
        # "I do not really know where to put this. \nWith that, I am grabbing the gcodeCommand here because that way it might be more deterministic in that when you click the button the message currently there is used. If i grabbed the gcodeCommand in one of the other loops, there may be some delay before the sendGCodeCommand is actually run, and during this time the user might have changed the string; therefore, making the actual string sent to the printrBoard not the string that was in the G-code Command when the Send button was pressed."
        n48 = event-data() -> ()  [unwired: 1 in, 3 out]
        n49 = property on="pBot_gcodeCommand" class="Str"() -> ("Text.Text"=w137:string)  [unwired: 2 in, 2 out]
        n50 = call-poly "Enqueue Message.vi"("Message Data"=w137, "Message"="sendGCodeCommand", "Message Queue"=w140) -> ("error out"=w138:errorcluster, "dup Message Queue"=w139:refnum<queue>)  [unwired: 7 in]
      }
      event "pBot_yForward10", "pBot_xRight10": Mouse Enter {
        n51 = event-data() -> ()  [unwired: 1 in, 3 out]
        n52 = call-poly "Enqueue Message.vi"("Message Data"="+10" ("Message"), "Message"="updateXYmoveDisplay", "Message Queue"=w144) -> ("error out"=w142:errorcluster, "dup Message Queue"=w143:refnum<queue>)  [unwired: 7 in]
      }
      event "pBot_yForward1", "pBot_xRight1": Mouse Enter {
        n53 = event-data() -> ()  [unwired: 1 in, 3 out]
        n54 = call-poly "Enqueue Message.vi"("Message Data"="+1" ("Message"), "Message"="updateXYmoveDisplay", "Message Queue"=w149) -> ("error out"=w147:errorcluster, "dup Message Queue"=w148:refnum<queue>)  [unwired: 7 in]
      }
      event "pBot_yForward01", "pBot_xRight01": Mouse Enter {
        n55 = event-data() -> ()  [unwired: 1 in, 3 out]
        n56 = call-poly "Enqueue Message.vi"("Message Data"="+0.1" ("Message"), "Message"="updateXYmoveDisplay", "Message Queue"=w154) -> ("error out"=w152:errorcluster, "dup Message Queue"=w153:refnum<queue>)  [unwired: 7 in]
      }
      event "pBot_yBack10", "pBot_xLeft10": Mouse Enter {
        n57 = event-data() -> ()  [unwired: 1 in, 3 out]
        n58 = call-poly "Enqueue Message.vi"("Message Data"="-10" ("Message"), "Message"="updateXYmoveDisplay", "Message Queue"=w159) -> ("error out"=w157:errorcluster, "dup Message Queue"=w158:refnum<queue>)  [unwired: 7 in]
      }
      event "pBot_yBack1", "pBot_xLeft1": Mouse Enter {
        n59 = event-data() -> ()  [unwired: 1 in, 3 out]
        n60 = call-poly "Enqueue Message.vi"("Message Data"="-1" ("Message"), "Message"="updateXYmoveDisplay", "Message Queue"=w164) -> ("error out"=w162:errorcluster, "dup Message Queue"=w163:refnum<queue>)  [unwired: 7 in]
      }
      event "pBot_yBack01", "pBot_xLeft01": Mouse Enter {
        n61 = event-data() -> ()  [unwired: 1 in, 3 out]
        n62 = call-poly "Enqueue Message.vi"("Message Data"="-0.1" ("Message"), "Message"="updateXYmoveDisplay", "Message Queue"=w169) -> ("error out"=w167:errorcluster, "dup Message Queue"=w168:refnum<queue>)  [unwired: 7 in]
      }
      event "pBot_yForward01", "pBot_yForward10", "pBot_yForward1", "pBot_yBack10", "pBot_yBack01", "pBot_yBack1", "pBot_xLeft01", "pBot_xLeft10", "pBot_xLeft1", "pBot_xRight10", "pBot_xRight01", "pBot_xRight1": Mouse Leave {
        n63 = event-data() -> ()  [unwired: 1 in, 3 out]
        n64 = call-poly "Enqueue Message.vi"("Message Data"="X/Y" ("Message"), "Message"="updateXYmoveDisplay", "Message Queue"=w174) -> ("error out"=w172:errorcluster, "dup Message Queue"=w173:refnum<queue>)  [unwired: 7 in]
      }
      event "pBot_zDown01", "pBot_zDown10", "pBot_zDown1", "pBot_zUp10", "pBot_zUp01", "pBot_zUp1": Mouse Leave {
        n65 = event-data() -> ()  [unwired: 1 in, 3 out]
        n66 = call-poly "Enqueue Message.vi"("Message Data"="Z" ("Message"), "Message"="updateZmoveDisplay", "Message Queue"=w179) -> ("error out"=w177:errorcluster, "dup Message Queue"=w178:refnum<queue>)  [unwired: 7 in]
      }
      event "pBot_zDown01": Mouse Enter {
        n67 = event-data() -> ()  [unwired: 1 in, 3 out]
        n68 = call-poly "Enqueue Message.vi"("Message Data"="-0.1" ("Message"), "Message"="updateZmoveDisplay", "Message Queue"=w184) -> ("error out"=w182:errorcluster, "dup Message Queue"=w183:refnum<queue>)  [unwired: 7 in]
      }
      event "pBot_zDown10": Mouse Enter {
        n69 = event-data() -> ()  [unwired: 1 in, 3 out]
        n70 = call-poly "Enqueue Message.vi"("Message Data"="-10" ("Message"), "Message"="updateZmoveDisplay", "Message Queue"=w189) -> ("error out"=w187:errorcluster, "dup Message Queue"=w188:refnum<queue>)  [unwired: 7 in]
      }
      event "pBot_zDown1": Mouse Enter {
        n71 = event-data() -> ()  [unwired: 1 in, 3 out]
        n72 = call-poly "Enqueue Message.vi"("Message Data"="-1" ("Message"), "Message"="updateZmoveDisplay", "Message Queue"=w194) -> ("error out"=w192:errorcluster, "dup Message Queue"=w193:refnum<queue>)  [unwired: 7 in]
      }
      event "pBot_zUp10": Mouse Enter {
        n73 = event-data() -> ()  [unwired: 1 in, 3 out]
        n74 = call-poly "Enqueue Message.vi"("Message Data"="+10" ("Message"), "Message"="updateZmoveDisplay", "Message Queue"=w199) -> ("error out"=w197:errorcluster, "dup Message Queue"=w198:refnum<queue>)  [unwired: 7 in]
      }
      event "pBot_zUp01": Mouse Enter {
        n75 = event-data() -> ()  [unwired: 1 in, 3 out]
        n76 = call-poly "Enqueue Message.vi"("Message Data"="+0.1" ("Message"), "Message"="updateZmoveDisplay", "Message Queue"=w204) -> ("error out"=w202:errorcluster, "dup Message Queue"=w203:refnum<queue>)  [unwired: 7 in]
      }
      event "pBot_zUp1": Mouse Enter {
        n77 = event-data() -> ()  [unwired: 1 in, 3 out]
        n78 = call-poly "Enqueue Message.vi"("Message Data"="+1" ("Message"), "Message"="updateZmoveDisplay", "Message Queue"=w209) -> ("error out"=w207:errorcluster, "dup Message Queue"=w208:refnum<queue>)  [unwired: 7 in]
      }
      event "pBot_yHome": Value Change {
        n79 = event-data() -> ()  [unwired: 1 in, 3 out]
        n80 = call-poly "Enqueue Message.vi"("Message Data"=enum16{"Y", "X", "Z"}."Y", "Message"="homePBotAxis", "Message Queue"=w215) -> ("error out"=w213:errorcluster, "dup Message Queue"=w214:refnum<queue>)  [unwired: 7 in]
      }
      event "pBot_xHome": Value Change {
        n81 = event-data() -> ()  [unwired: 1 in, 3 out]
        n82 = call-poly "Enqueue Message.vi"("Message Data"=enum16{"Y", "X", "Z"}."X", "Message"="homePBotAxis", "Message Queue"=w220) -> ("error out"=w218:errorcluster, "dup Message Queue"=w219:refnum<queue>)  [unwired: 7 in]
      }
      event "pBot_zHome": Value Change {
        n83 = event-data() -> ()  [unwired: 1 in, 3 out]
        n84 = call-poly "Enqueue Message.vi"("Message Data"=enum16{"Y", "X", "Z"}."Z", "Message"="homePBotAxis", "Message Queue"=w225) -> ("error out"=w223:errorcluster, "dup Message Queue"=w224:refnum<queue>)  [unwired: 7 in]
      }
      event "pBot_yForward01": Value Change {
        n85 = event-data() -> ()  [unwired: 1 in, 3 out]
        n86 = call-poly "Enqueue Message.vi"("Message Data"=T12 {"Direction"=enum."Y", "Amount"=0.1}, "Message"="moveRelative", "Message Queue"=w231) -> ("error out"=w227:errorcluster, "dup Message Queue"=w228:refnum<queue>)  [unwired: 7 in]
      }
      event "pBot_yForward10": Value Change {
        n87 = event-data() -> ()  [unwired: 1 in, 3 out]
        n88 = call-poly "Enqueue Message.vi"("Message Data"=T12 {"Direction"=enum."Y", "Amount"=10.0}, "Message"="moveRelative", "Message Queue"=w236) -> ("error out"=w232:errorcluster, "dup Message Queue"=w233:refnum<queue>)  [unwired: 7 in]
      }
      event "pBot_yForward1": Value Change {
        n89 = event-data() -> ()  [unwired: 1 in, 3 out]
        n90 = call-poly "Enqueue Message.vi"("Message Data"=T12 {"Direction"=enum."Y", "Amount"=1.0}, "Message"="moveRelative", "Message Queue"=w241) -> ("error out"=w237:errorcluster, "dup Message Queue"=w238:refnum<queue>)  [unwired: 7 in]
      }
      event "pBot_yBack10": Value Change {
        n91 = event-data() -> ()  [unwired: 1 in, 3 out]
        n92 = call-poly "Enqueue Message.vi"("Message Data"=T12 {"Direction"=enum."Y", "Amount"=-10.0}, "Message"="moveRelative", "Message Queue"=w246) -> ("error out"=w242:errorcluster, "dup Message Queue"=w243:refnum<queue>)  [unwired: 7 in]
      }
      event "pBot_yBack01": Value Change {
        n93 = event-data() -> ()  [unwired: 1 in, 3 out]
        n94 = call-poly "Enqueue Message.vi"("Message Data"=T12 {"Direction"=enum."Y", "Amount"=-0.1}, "Message"="moveRelative", "Message Queue"=w251) -> ("error out"=w247:errorcluster, "dup Message Queue"=w248:refnum<queue>)  [unwired: 7 in]
      }
      event "pBot_yBack1": Value Change {
        n95 = event-data() -> ()  [unwired: 1 in, 3 out]
        n96 = call-poly "Enqueue Message.vi"("Message Data"=T12 {"Direction"=enum."Y", "Amount"=-1.0}, "Message"="moveRelative", "Message Queue"=w256) -> ("error out"=w252:errorcluster, "dup Message Queue"=w253:refnum<queue>)  [unwired: 7 in]
      }
      event "pBot_xLeft01": Value Change {
        n97 = event-data() -> ()  [unwired: 1 in, 3 out]
        n98 = call-poly "Enqueue Message.vi"("Message Data"=T12 {"Direction"=enum."X", "Amount"=-0.1}, "Message"="moveRelative", "Message Queue"=w261) -> ("error out"=w257:errorcluster, "dup Message Queue"=w258:refnum<queue>)  [unwired: 7 in]
      }
      event "pBot_xLeft10": Value Change {
        n99 = event-data() -> ()  [unwired: 1 in, 3 out]
        n100 = call-poly "Enqueue Message.vi"("Message Data"=T12 {"Direction"=enum."X", "Amount"=-10.0}, "Message"="moveRelative", "Message Queue"=w266) -> ("error out"=w262:errorcluster, "dup Message Queue"=w263:refnum<queue>)  [unwired: 7 in]
      }
      event "pBot_xLeft1": Value Change {
        n101 = event-data() -> ()  [unwired: 1 in, 3 out]
        n102 = call-poly "Enqueue Message.vi"("Message Data"=T12 {"Direction"=enum."X", "Amount"=-1.0}, "Message"="moveRelative", "Message Queue"=w271) -> ("error out"=w267:errorcluster, "dup Message Queue"=w268:refnum<queue>)  [unwired: 7 in]
      }
      event "pBot_xRight10": Value Change {
        n103 = event-data() -> ()  [unwired: 1 in, 3 out]
        n104 = call-poly "Enqueue Message.vi"("Message Data"=T12 {"Direction"=enum."X", "Amount"=10.0}, "Message"="moveRelative", "Message Queue"=w276) -> ("error out"=w272:errorcluster, "dup Message Queue"=w273:refnum<queue>)  [unwired: 7 in]
      }
      event "pBot_xRight01": Value Change {
        n105 = event-data() -> ()  [unwired: 1 in, 3 out]
        n106 = call-poly "Enqueue Message.vi"("Message Data"=T12 {"Direction"=enum."X", "Amount"=0.1}, "Message"="moveRelative", "Message Queue"=w281) -> ("error out"=w277:errorcluster, "dup Message Queue"=w278:refnum<queue>)  [unwired: 7 in]
      }
      event "pBot_xRight1": Value Change {
        n107 = event-data() -> ()  [unwired: 1 in, 3 out]
        n108 = call-poly "Enqueue Message.vi"("Message Data"=T12 {"Direction"=enum."X", "Amount"=1.0}, "Message"="moveRelative", "Message Queue"=w286) -> ("error out"=w282:errorcluster, "dup Message Queue"=w283:refnum<queue>)  [unwired: 7 in]
      }
      event "pBot_zDown01": Value Change {
        n109 = event-data() -> ()  [unwired: 1 in, 3 out]
        n110 = call-poly "Enqueue Message.vi"("Message Data"=T12 {"Direction"=enum."Z", "Amount"=-0.1}, "Message"="moveRelative", "Message Queue"=w291) -> ("error out"=w287:errorcluster, "dup Message Queue"=w288:refnum<queue>)  [unwired: 7 in]
      }
      event "pBot_zDown10": Value Change {
        n111 = event-data() -> ()  [unwired: 1 in, 3 out]
        n112 = call-poly "Enqueue Message.vi"("Message Data"=T12 {"Direction"=enum."Z", "Amount"=-10.0}, "Message"="moveRelative", "Message Queue"=w296) -> ("error out"=w292:errorcluster, "dup Message Queue"=w293:refnum<queue>)  [unwired: 7 in]
      }
      event "pBot_zDown1": Value Change {
        n113 = event-data() -> ()  [unwired: 1 in, 3 out]
        n114 = call-poly "Enqueue Message.vi"("Message Data"=T12 {"Direction"=enum."Z", "Amount"=-1.0}, "Message"="moveRelative", "Message Queue"=w301) -> ("error out"=w297:errorcluster, "dup Message Queue"=w298:refnum<queue>)  [unwired: 7 in]
      }
      event "pBot_zUp10": Value Change {
        n115 = event-data() -> ()  [unwired: 1 in, 3 out]
        n116 = call-poly "Enqueue Message.vi"("Message Data"=T12 {"Direction"=enum."Z", "Amount"=10.0}, "Message"="moveRelative", "Message Queue"=w306) -> ("error out"=w302:errorcluster, "dup Message Queue"=w303:refnum<queue>)  [unwired: 7 in]
      }
      event "pBot_zUp01": Value Change {
        n117 = event-data() -> ()  [unwired: 1 in, 3 out]
        n118 = call-poly "Enqueue Message.vi"("Message Data"=T12 {"Direction"=enum."Z", "Amount"=0.1}, "Message"="moveRelative", "Message Queue"=w311) -> ("error out"=w307:errorcluster, "dup Message Queue"=w308:refnum<queue>)  [unwired: 7 in]
      }
      event "pBot_zUp1": Value Change {
        n119 = event-data() -> ()  [unwired: 1 in, 3 out]
        n120 = call-poly "Enqueue Message.vi"("Message Data"=T12 {"Direction"=enum."Z", "Amount"=1.0}, "Message"="moveRelative", "Message Queue"=w316) -> ("error out"=w312:errorcluster, "dup Message Queue"=w313:refnum<queue>)  [unwired: 7 in]
      }
      event "pBot_scanningXmin", "pBot_scanningXmax", "pBot_scanningYmin", "pBot_scanningYmax", "pBot_scanningZmin", "pBot_scanningZmax", "pBot_scanNx", "pBot_scanNy", "pBot_scanNz": Value Change {
        n121 = event-data() -> ()  [unwired: 1 in, 3 out]
        n122 = call-poly "Enqueue Message.vi"("Message"="updateScanRegion", "Message Queue"=w319) -> ("error out"=w317:errorcluster, "dup Message Queue"=w318:refnum<queue>)  [unwired: 8 in]
      }
      event "pBot_runScan": Value Change {
        n123 = event-data() -> ()  [unwired: 1 in, 3 out]
        n124 = call-poly "Enqueue Message.vi"("Message"="startScan", "Message Queue"=w323) -> ("error out"=w321:errorcluster, "dup Message Queue"=w322:refnum<queue>)  [unwired: 8 in]
      }
      event "usb2000p_VISAstrings": Mouse Down? {
        n125 = event-data() -> ()  [unwired: 1 in, 3 out]
        n126 = call-poly "Enqueue Message.vi"("Message"="usb2000p_getInstruments" ("expression (\"?*\")"), "Message Queue"=w328) -> ("error out"=w326:errorcluster, "dup Message Queue"=w327:refnum<queue>)  [unwired: 8 in]
        n127 = event-data() -> ()  [unwired: 2 in, 1 out]
      }
      event "usb2000p_ConnectButton": Value Change {
        n128 = event-data() -> ()  [unwired: 1 in, 3 out]
        n129 = call-poly "Enqueue Message.vi"("Message"="usb2000p_tryToConnect" ("expression (\"?*\")"), "Message Queue"=w332) -> ("error out"=w330:errorcluster, "dup Message Queue"=w331:refnum<queue>)  [unwired: 8 in]
      }
      event "usb2000p_intTime": Value Change {
        n130 = event-data() -> ()  [unwired: 1 in, 3 out]
        n131 = call-poly "Enqueue Message.vi"("Message"="usb2000p_setIntegrationTime" ("expression (\"?*\")"), "Message Queue"=w336) -> ("error out"=w334:errorcluster, "dup Message Queue"=w335:refnum<queue>)  [unwired: 8 in]
      }
      event "usb2000p_aquireSpectra": Value Change {
        n132 = event-data() -> ()  [unwired: 1 in, 3 out]
        n133 = call-poly "Enqueue Message.vi"("Message"="usb2000p_acquireSpec" ("expression (\"?*\")"), "Message Queue"=w340) -> ("error out"=w338:errorcluster, "dup Message Queue"=w339:refnum<queue>)  [unwired: 8 in]
      }
      event "usb2000p_saveSpectra": Value Change {
        n134 = event-data() -> ()  [unwired: 1 in, 3 out]
        n135 = call-poly "Enqueue Message.vi"("Message"="savePlot" ("expression (\"?*\")"), "Message Queue"=w344) -> ("error out"=w342:errorcluster, "dup Message Queue"=w343:refnum<queue>)  [unwired: 8 in]
      }
      event User Event {
        # "The Message Handling Loop processed an \"Exit\" message, which fired this event to stop the Event Handling Loop."
        n136 = event-data() -> ()  [unwired: 1 in, 2 out]
      }
      event Panel Close? {
        # "Send the 'Confirm Quit' message if the user closes the panel of the VI. Discard the event so the 'Confirm Quit' message has a chance to run."
        n137 = event-data() -> ()  [unwired: 1 in, 1 out]
        n138 = call-poly "Enqueue Message.vi"("Priority Message? (F)"=TRUE, "Message"="Confirm Quit", "Message Queue"=w351) -> ("error out"=w350:errorcluster, "dup Message Queue"=w349:refnum<queue>)  [unwired: 7 in]
        n139 = event-data("Discard?"=TRUE) -> ()  [unwired: 1 in, 1 out]
      }
      event Application Instance Close {
        # "#CodeRecommended - When a project closes, all VIs within that project are aborted and leave memory. However, any code placed in this event frame is guaranteed to run to completion, so add any cleanup code that absolutely must happen here."
        n140 = event-data() -> ()  [unwired: 1 in, 1 out]
      }
    }
    n141 = call "Error Handler - Event Handling Loop.vi"("error in (no error)"=w20, "Message Queue"=w21) -> ()  [unwired: 8 in, 2 out]
    n142 = call "Error Handler - Event Handling Loop.vi"("error in (no error)"=w26, "Message Queue"=w24) -> ("dup error in"=w23:errorcluster)  [unwired: 8 in, 1 out]
  }
  n143 = while {
    tunnel: w2 -> [w362]
    tunnel: w7 -> [w361]
    tunnel: [w357] -> w5
    shift-right: [w355] -> _
    shift-left: w4 -> [w356]
    tunnel: w3 -> [w354]
    stop <- w358 stop-if-true
    # "Equipment Control / Data Aquisition Loop"
    n144 = call "Dequeue Message.vi"("error in (no error)"=w361, "Message Queue"=w362) -> ("error out"=w363:errorcluster, "Message Data"=w364:variant, "Message"=w365:string, "dup Message Queue"=w360:refnum<queue>)  [unwired: 6 in]
    n145 = case "Message Cases" shown="\"startScan\"" w365 {
      selector: w365 -> [_ _ _ _ _ _ _ _ _ _ _ _ _ _ _ _ w1188]
      tunnel: w360 -> [_ w417 _ _ _ _ _ w577 w599 _ w906 w1070 _ _ w1175 w1179 _]
      tunnel: w364 -> [w373 _ w461 _ w504 w538 w562 _ w622 w857 _ w1078 w1131 _ w1170 w1183 _]
      tunnel: w363 -> [w374 w420 w462 w476 w505 w539 w563 w579 w623 w858 _ w1077 w1132 w1162 w1171 w1180 _]
      tunnel: [w366 w420 w455 w481 w484 w533 w555 w579 errorcluster {"status"=FALSE, "code"=0, "source"=""} ("error out") errorcluster {"status"=FALSE, "code"=0, "source"=""} ("error out") errorcluster {"status"=FALSE, "code"=0, "source"=""} ("error out") w1071 w1125 w1162 w1167 w1185 w1187] -> w359
      tunnel: [_ _ _ _ _ _ _ _ _ _ _ _ _ _ _ TRUE _] -> w358
      tunnel: w356 -> [w368 w423 w441 w472 w488 w532 w554 w578 w596 w851 w907 w1073 w1128 w1161 w1166 w1177 w1186]
      tunnel: [w367 w421 w440 w472 w487 w532 w550 w578 w620 w849 w904 w1072 w1126 w1158 w1165 w1177 w1186] -> w355
      tunnel: w354 -> [w369 w424 w456 w482 w492 w536 w556 w580 w610 w850 w902 w1069 _ _ w1173 _ _]
      frame "connectToPBot" {
        n146 = Variant To Data(error in=w374, type="", Variant=w373) -> (data=w371:string, error out=w370:errorcluster)
        n147 = case shown="No Error" w370 {
          tunnel: w371 -> [w382 _]
          tunnel: w369 -> [w377 w415]
          tunnel: w368 -> [w380 w416]
          tunnel: [w378 w416] -> w367
          tunnel: [errorcluster {"status"=FALSE, "code"=0, "source"=""} ("error constant") errorcluster {"status"=FALSE, "code"=0, "source"=""} ("error constant")] -> w366
          frame No Error {
            w389 = u16 2 items=["None", "Last Bit", "TermChar", "Break"] ("Serial Settings:End Mode for Writes")
            # "0.01 sec"
            n148 = call-poly "VISA Configure Serial Port"("VISA resource name"=w382, "timeout (10sec)"=u32 10) -> ("VISA resource name out"=w390:refnum<visa-resource-name>, "error out"=w388:errorcluster)  [unwired: 12 in]
            n149 = property class="Instr"(reference=w390, error in=w388, "ASRL End Out"=w389) -> (reference out=w386:refnum<visa-resource-name>, error out=w387:errorcluster)
            n150 = VISA Open(error in (no error)=w387, VISA resource name=w386) -> (VISA resource name=w385:refnum<visa-resource-name>, error out=w384:errorcluster)  [unwired: 3 in]
            n151 = call "visaQuery.vi"("error constant"=w384, "stringToWrite"="M501", "VISA resource name"=w385) -> ("error Out"=w381:errorcluster, "String"=w375:string, "dub: VISA resource name"=w379:refnum<visa-resource-name>)  [unwired: 6 in]
            n152 = case shown="No Error" w381 {
              tunnel: w380 -> [w407 w411]
              tunnel: w379 -> [w406 _]
              tunnel: [w404 w411] -> w378
              tunnel: w377 -> [w397 w408]
              tunnel: w375 -> [w393 _]
              frame No Error {
                w400 = FALSE  # diconnectPBot_Event
                # "this will extract info from\nEEPROM settings"
                n153 = Create User Event(user event datatype=w400) -> (user event=w399:refnum<user-event>)  [unwired: 1 in, 1 out]
                n154 = Bundle By Name(cluster=T15 {"commandID"="M501", "gCode"="M501", "extraInfo"="noDisplay", "originatingCommandID"="initialization", "error"={"status"=FALSE, "code"=0, "source"=""}}, "gCode"=w393) -> (w394:T15)
                n155 = call "getTravelRange.vi"("EEPROM_string"=w393) -> ("travelRange"=w392:cluster{"X":dbl, "Y":dbl, "Z":dbl})  [unwired: 9 in, 1 out]
                n156 = call-poly "Enqueue Message.vi"("Message Data"=w394, "Message"="recieveMessageFromPBot", "Message Queue"=w397) -> ("dup Message Queue"=w398:refnum<queue>)  [unwired: 7 in, 1 out]
                n157 = Bundle By Name(cluster=T11 {"Message"="equip", "error constant"={"status"=FALSE, "code"=0, "source"=""}, "disconnectPBot_Event"=refnum}, "error constant.source"=w393, "disconnectPBot_Event"=w399) -> (w401:T11)
                n158 = Bundle By Name(cluster=w407, "disconnectPBot_Event"=w399, "pBotConnected?"=TRUE, "pBot_VISA"=w406, "pBot_currentEEPROMsettings"=w393, "travelRange"=w392) -> (w404:T5)
                n159 = call-poly "Enqueue Message.vi"("Message Data"=w401, "Message"="connectToPBot", "Message Queue"=w398) -> ()  [unwired: 7 in, 2 out]
              }
              frame Error {
                n160 = call-poly "Enqueue Message.vi"("Message Data"=T11 {"Message"="equip", "error constant"={"status"=TRUE, "code"=0, "source"="Error! Not able to connect to plasmaBot!"}, "disconnectPBot_Event"=refnum}, "Message"="connectToPBot", "Message Queue"=w408) -> ()  [unwired: 7 in, 2 out]
              }
            }
          }
          frame Error {
            n161 = call-poly "Enqueue Message.vi"("Message Data"=T11 {"Message"="equip", "error constant"={"status"=TRUE, "code"=0, "source"="Error sending VISA value to equipment control loop"}, "disconnectPBot_Event"=refnum}, "Message"="connectToPBot", "Message Queue"=w415) -> ()  [unwired: 7 in, 2 out]
          }
        }
      }
      frame "disconnectFromPBot" {
        n162 = Unbundle By Name(w423) -> ("ish5FileOpen?"=w418:bool, "disconnectPBot_Event"=w419:refnum<user-event>, "pBot_VISA"=w428:refnum<visa-resource-name>)
        n163 = Destroy User Event(user event=w419) -> ()  [unwired: 1 in, 1 out]
        n164 = VISA Close(VISA resource name=w428) -> (error out=w427:errorcluster)  [unwired: 1 in]
        n165 = case shown="True" w418 {
          tunnel: w417 -> [_ w430]
          frame False {
          }
          frame True {
            n166 = call-poly "Enqueue Message.vi"("Message"="closeH5File", "Message Queue"=w430) -> ()  [unwired: 8 in, 2 out]
          }
        }
        n167 = case shown="Error" w427 {
          selector: w427 -> [_ w436]
          tunnel: [T11 {"Message"="equip", "error constant"={"status"=FALSE, "code"=0, "source"="Disconnected from plasmaBot"}, "disconnectPBot_Event"=refnum} w433] -> w426
          frame No Error {
          }
          frame Error {
            n168 = Unbundle(w436) -> ("source"=w439:string)  [unwired: 2 out]
            n169 = Concatenate Strings("Error disconnecting plasmaBot! (It should not be a problem to just shut the power off if you must.)", "\n", w439) -> (w435:string)
            n170 = Bundle By Name(cluster=w436, "source"=w435) -> (w434:errorcluster)
            n171 = Bundle By Name(cluster=T11 {"Message"="equip", "error constant"={"status"=FALSE, "code"=0, "source"=""}, "disconnectPBot_Event"=refnum}, "error constant"=w434) -> (w433:T11)
          }
        }
        n172 = call-poly "Enqueue Message.vi"("Message Data"=w426, "Message"="connectToPBot", "Message Queue"=w424) -> ()  [unwired: 7 in, 2 out]
        n173 = Bundle By Name(cluster=w423, "pBot_VISA"=refnum<visa-resource-name> refnum) -> (w421:T5)
      }
      frame "sendGCodeCommand" {
        n174 = Unbundle By Name(w441) -> ("pBot_VISA"=w460:refnum<visa-resource-name>, "disconnectPBot_Event"=w454:refnum<user-event>)
        n175 = Variant To Data(error in=w462, type=T15 {"commandID"=" ", "gCode"=" ", "extraInfo"=" ", "originatingCommandID"=" ", "error"={"status"=FALSE, "code"=0, "source"=""}}, Variant=w461) -> (data=w450:T15, error out=w459:errorcluster)
        n176 = Unbundle By Name(w450) -> ("gCode"=w443:string)
        n177 = call "visaQuery.vi"("error constant"=w459, "disconnectPBot_Event"=w454, "stringToWrite"=w443, "VISA resource name"=w460) -> ("error Out"=w458:errorcluster, "String"=w452:string)  [unwired: 5 in, 1 out]
        n178 = case shown="No Error" w458 {
          selector: w458 -> [w469 w471]
          tunnel: [w469 w471] -> w448
          tunnel: w452 -> [w468 w470]
          tunnel: [w468 w470] -> w442
          frame No Error {
            # "Note that the string returned is the status of the error if there is no error.\nDo something if necessary"
          }
          frame Error {
          }
        }
        n179 = Equal?(x="M501" ("y"), y=w443) -> (x = y?=w449:bool)
        n180 = Unbundle By Name(w448) -> ("status"=w447:bool)
        n181 = Not(x=w447) -> (.not. x?=w446:bool)
        n182 = Bundle By Name(cluster=w450, "gCode"=w442, "error"=w448) -> (w451:T15)
        n183 = And(x=w446, y=w449) -> (x .and. y?=w445:bool)
        n184 = case shown="True" w445 {
          tunnel: w442 -> [_ w466]
          tunnel: w441 -> [w463 w467]
          tunnel: [w463 w464] -> w440
          frame False {
          }
          frame True {
            n185 = call "getTravelRange.vi"("EEPROM_string"=w466) -> ("travelRange"=w465:cluster{"X":dbl, "Y":dbl, "Z":dbl})  [unwired: 9 in, 1 out]
            n186 = Bundle By Name(cluster=w467, "pBot_currentEEPROMsettings"=w466, "travelRange"=w465) -> (w464:T5)
          }
        }
        n187 = call-poly "Enqueue Message.vi"("Message Data"=w451, "Message"="recieveMessageFromPBot", "Message Queue"=w456) -> ("error out"=w455:errorcluster)  [unwired: 7 in, 1 out]
      }
      frame "getCurrentInfo" {
        n188 = call "currentLocation.vi"("Equip_Data"=w472) -> ("error out"=w477:errorcluster, "position"=w473:cluster{"X":dbl, "Y":dbl, "Z":dbl})  [unwired: 9 in]
        n189 = call "read_pbot_temperature.vi"("Equip_Data"=w472) -> ("error out"=w478:errorcluster, "Temperature"=w474:dbl)  [unwired: 9 in]
        n190 = Merge Errors(w477, w478, w476) -> (w475:errorcluster)
        n191 = Bundle(cluster=T16 {"currentPos"={"X"=0.0, "Y"=0.0, "Z"=0.0}, "temperature"=0.0, "error constant"={"status"=FALSE, "code"=0, "source"=""}}, "currentPos"=w473, "temperature"=w474, "error constant"=w475) -> (w480:T16)
        n192 = call-poly "Enqueue Message.vi"("Message Data"=w480, "Message"="getCurrentInfo", "Message Queue"=w482) -> ("error out"=w481:errorcluster)  [unwired: 7 in, 1 out]
      }
      frame "usb2000p_Connect" {
        n193 = Variant To Data(error in=w505, type=T7 {"Name"="", "VISAname"="", "1D_dataArraySize"=0, "extraInfo"=variant, "error"={"status"=FALSE, "code"=0, "source"=""}} ("instrumentInfo"), Variant=w504) -> (data=w489:T7, error out=w484:errorcluster)
        n194 = Unbundle By Name(w489) -> ("VISAname"=w501:refnum<visa-resource-name>)
        n195 = call <instrlib>:"Initialize.vi"("VISA resource name"=w501) -> ("error out"=w503:errorcluster, "VISA resource name out"=w502:refnum<visa-resource-name>)  [unwired: 1 in, 8 out]
        n196 = call <instrlib>:"Configure Strobe.vi"("error in (no error)"=w503, "VISA resource name"=w502) -> ("error out"=w496:errorcluster, "VISA resource name out"=w497:refnum<visa-resource-name>)  [unwired: 1 in, 7 out]
        n197 = property class="USB Raw"(reference=w497, error in=w496) -> (reference out=w499:refnum<visa-resource-name>, error out=w500:errorcluster, "User Data"=w498:u32)
        n198 = Split Number(x=w498) -> (lo(x)=w485:u16)  [unwired: 1 out]
        n199 = case shown="4118" w485 {
          tunnel: [2049 ("Number of Pixels (3840)") 2022 ("Number of Pixels (3840)") 3648 ("Number of Pixels (3840)") 2028 ("Number of Pixels (3840)") 1024 ("Number of Pixels (3840)") 2028 ("Number of Pixels (3840)") 512 ("Number of Pixels (3840)") 256 ("Number of Pixels (3840)") 2038 ("Number of Pixels (3840)") 2048 ("Number of Pixels (3840)") 0 ("Number of Pixels (3840)")] -> w486
          frame 4098, 4100 {
          }
          frame 4106 {
          }
          frame 4114, 4130 {
          }
          frame 4118 {
          }
          frame 4120 {
          }
          frame 4126, 4160 {
          }
          frame 4134 {
          }
          frame 4136 {
          }
          frame 4138 {
          }
          frame 4140 {
          }
          frame Default {
          }
        }
        n200 = call <instrlib>:"Calculate Wavelength.vi"("error in (no error)"=w500, "Number of Pixels (3648)"=w486, "VISA resource name"=w499) -> ("error out"=w495:errorcluster, "Wavelength (nm)"=w494:dbl[], "VISA resource name out"=w493:refnum<visa-resource-name>)  [unwired: 6 out]
        n201 = case shown="No Error" w495 {
          selector: w495 -> [w518 w527]
          tunnel: w494 -> [w519 _]
          tunnel: w493 -> [w520 _]
          tunnel: w486 -> [w521 _]
          tunnel: [w522 w528] -> w491
          tunnel: w489 -> [w525 _]
          tunnel: w488 -> [w524 w526]
          tunnel: [w523 w526] -> w487
          frame No Error {
            n202 = Bundle By Name(cluster=w525, "1D_dataArraySize"=w521, "extraInfo"=w519, "error"=w518, "VISAname"=w520) -> (w522:T7)
            n203 = Bundle By Name(cluster=w524, "USB2000p_Info"=w522) -> (w523:T5)
          }
          frame Error {
            n204 = Bundle By Name(cluster=T7 {"Name"="", "VISAname"="", "1D_dataArraySize"=0, "extraInfo"=variant, "error"={"status"=FALSE, "code"=0, "source"=""}} ("instrumentInfo"), "error"=w527) -> (w528:T7)
          }
        }
        n205 = call-poly "Enqueue Message.vi"("Message Data"=w491, "Message"="usb2000p_connected?", "Message Queue"=w492) -> ()  [unwired: 7 in, 2 out]
      }
      frame "usb2000p_Disconnect" {
        n206 = Variant To Data(error in=w539, type=T7 {"Name"="", "VISAname"="", "1D_dataArraySize"=0, "extraInfo"=variant, "error"={"status"=FALSE, "code"=0, "source"=""}} ("instrumentInfo"), Variant=w538) -> (data=w537:T7, error out=w533:errorcluster)
        n207 = Unbundle By Name(w537) -> ("VISAname"=w531:refnum<visa-resource-name>)
        n208 = call <instrlib>:"Close.vi"("VISA resource name"=w531) -> ("error out"=w530:errorcluster)  [unwired: 1 in, 9 out]
        n209 = case shown="No Error" w530 {
          selector: w530 -> [w544 w547]
          tunnel: [w545 w548] -> w535
          frame No Error {
            n210 = Bundle By Name(cluster=w544, "status"=TRUE, "source"="Disconnected from USB2000+") -> (w541:errorcluster)
            n211 = Bundle By Name(cluster=T7 {"Name"="", "VISAname"="", "1D_dataArraySize"=0, "extraInfo"=variant, "error"={"status"=FALSE, "code"=0, "source"=""}} ("instrumentInfo"), "error"=w541) -> (w545:T7)
          }
          frame Error {
            n212 = Bundle By Name(cluster=T7 {"Name"="", "VISAname"="", "1D_dataArraySize"=0, "extraInfo"=variant, "error"={"status"=FALSE, "code"=0, "source"=""}} ("instrumentInfo"), "error"=w547) -> (w548:T7)
          }
        }
        n213 = call-poly "Enqueue Message.vi"("Message Data"=w535, "Message"="usb2000p_connected?", "Message Queue"=w536) -> ()  [unwired: 7 in, 2 out]
      }
      frame "usb2000p_setIntegrationTime" {
        n214 = Unbundle By Name(w554) -> ("USB2000p_Info.VISAname"=w560:refnum<visa-resource-name>)
        n215 = Variant To Data(error in=w563, type=u32 0 ("usb2000p_intTime"), Variant=w562) -> (data=w553:u32, error out=w555:errorcluster)
        n216 = Multiply(x=w553, y=u32 1000) -> (x*y=w551:u32)
        n217 = call <instrlib>:"Configure Integration Time.vi"("Integration Time (6000)"=w551, "VISA resource name"=w560) -> ("error out"=w559:errorcluster)  [unwired: 1 in, 8 out]
        n218 = case shown="Error" w559 {
          selector: w559 -> [_ w571]
          tunnel: ["Integration time set" ("Message") w569] -> w557
          tunnel: w554 -> [w566 w568]
          tunnel: w553 -> [w565 _]
          tunnel: [w564 w568] -> w550
          frame No Error {
            n219 = Bundle By Name(cluster=w566, "integrationTime"=w565) -> (w564:T5)
          }
          frame Error {
            n220 = Unbundle By Name(w571) -> ("source"=w570:string)
            n221 = Concatenate Strings("Error! The integration time was not set:" ("Message"), "\n", w570) -> (w569:string)
          }
        }
        n222 = call-poly "Enqueue Message.vi"("Message Data"=w557, "Message"="messageFromEquipLoop", "Message Queue"=w556) -> ()  [unwired: 7 in, 2 out]
      }
      frame "usb2000p_acquireSpec" {
        n223 = Unbundle By Name(w578) -> ("USB2000p_Info.VISAname"=w574:refnum<visa-resource-name>)
        n224 = call <instrlib>:"Read Optical Spectrum.vi"("VISA resource name"=w574) -> ("error out"=w575:errorcluster, "Spectrum by Pixels"=w576:dbl[])  [unwired: 7 in, 2 out]
        n225 = case shown="No Error" w575 {
          selector: w575 -> [_ w590]
          tunnel: w580 -> [w581 w593]
          tunnel: w576 -> [w584 _]
          tunnel: w577 -> [w582 _]
          frame No Error {
            n226 = call-poly "Enqueue Message.vi"("Message Data"=w584, "Message"="plotData", "Message Queue"=w581) -> ()  [unwired: 7 in, 2 out]
            n227 = local read "usb2000p_continuous?"() -> (w583:bool)
            n228 = case shown="True" w583 {
              tunnel: w582 -> [_ w587]
              frame False {
              }
              frame True {
                n229 = call-poly "Enqueue Message.vi"("Message"="usb2000p_acquireSpec", "Message Queue"=w587) -> ()  [unwired: 8 in, 2 out]
              }
            }
          }
          frame Error {
            n230 = Unbundle By Name(w590) -> ("source"=w589:string)
            n231 = Concatenate Strings("Error! Not able to obtain spectra from USB2000+:" ("Message"), "\n", w589) -> (w588:string)
            n232 = call-poly "Enqueue Message.vi"("Message Data"=w588, "Message"="messageFromEquipLoop", "Message Queue"=w593) -> ()  [unwired: 7 in, 2 out]
          }
        }
      }
      frame "startScan" {
        # "Initialize data for the scan, open a .h5 file to save the data, and start the message calls that will carry out the scan. \nIf, eventually, there should be more than one scan instrument, then make the scanInstrimentInfo cluster (in the input cluster) an array that stores the information for each instrument and then use a for loop to iterate over each instrument: create the data set (or data file) for each. The incrementScan function  moves to the next position and then calls a function that should run each instrument to collect data at the current position, then save the data, then again call incrementScan."
        n233 = Variant To Data(error in=w623, type=T6 {"dataFilePath"=path "", "scanPoints"={"dim1"=[], "dim2"=[], "dim3"=[]}, "N"={"X"=0, "Y"=0, "Z"=0}, "scanInstrumentInfo"={"Name"="", "VISAname"="", "1D_dataArraySize"=0, "extraInfo"=variant, "error"={"status"=FALSE, "code"=0, "source"=""}}}, Variant=w622) -> (data=w612:T6)  [unwired: 1 out]
        n234 = Unbundle(w612) -> ("dataFilePath"=w619:path, "scanPoints"=w609:T19, "N"=w602:cluster{"X":u16, "Y":u16, "Z":u16}, "scanInstrumentInfo"=w606:T7)
        n235 = Unbundle(w602) -> ("X"=w614:u16, "Y"=w615:u16, "Z"=w616:u16)
        n236 = Unbundle(w606) -> ("1D_dataArraySize"=w598:u16)  [unwired: 4 out]
        n237 = Not Equal To 0?(x=w598) -> (x != 0?=w597:bool)
        n238 = To Unsigned Long Integer(number=w602) -> (unsigned 32bit integer=w601:cluster{"X":u32, "Y":u32, "Z":u32})
        n239 = Unbundle(w601) -> ("X"=w605:u32, "Y"=w604:u32, "Z"=w603:u32)
        n240 = Compound Arithmetic op=MULTIPLY(w605, w604, w603) -> (w600:u32)
        n241 = Unbundle By Name(w596) -> ("integrationTime"=w595:u32)
        n242 = case shown="False" w597 {
          tunnel: w619 -> [w655 w758]
          tunnel: [w652 w755] -> w618
          tunnel: [w651 w754] -> w617
          tunnel: w616 -> [w632 w753]
          tunnel: w615 -> [w650 w752]
          tunnel: w614 -> [w649 w751]
          tunnel: w598 -> [w648 _]
          tunnel: [w646 w749] -> w613
          tunnel: w609 -> [w636 w738]
          tunnel: [w627 w734] -> w608
          tunnel: [w628 w733] -> w607
          tunnel: w595 -> [w624 _]
          frame True {
            w626 = ""
            # "dims: z, y, x, spec"
            n243 = Increment(x=w632) -> (x+1=w631:u16)
            n244 = Unbundle(w636) -> ("dim1"=w633:sgl[], "dim2"=w634:sgl[], "dim3"=w635:sgl[])
            n245 = Initialize Array(u16 0 ("element"), u32 1 ("dimension size"), w650, w649, w648) -> (w651:u16[][][][])
            n246 = Build Array(w631, w650, w649, w648) -> (w647:u16[])
            n247 = call <vilib>:"H5Fopen.vi"("mode (read-only)"=H5Fmode."overwrite" ("mode"), "path"=w655) -> ("error out"=w654:errorcluster, "ref out"=w652:T8)  [unwired: 8 in]
            n248 = Array Size(array=w651) -> (size(s)=w646:i32[])
            n249 = call <vilib>:"H5Dcreate_simple.vi"("max size"=w647, "chunk size"=w646, "error in (no error)"=w654, "type in"=w651, "name"="data", "ref in"=w652) -> ("error out"=w637:errorcluster, "dset out"=w638:T8)  [unwired: 4 in]
            n250 = xnode "H5Awrite.xnode"("object name"=w626, "error in (no error)"=w637, "data"=w633, "attrib name"="X", "ref in"=w638) -> ("error out"=w640:errorcluster, "ref out"=w642:T8)  [unwired: 2 in, 1 out]
            n251 = xnode "H5Awrite.xnode"("object name"=w626, "error in (no error)"=w640, "data"=w634, "attrib name"="Y", "ref in"=w642) -> ("error out"=w639:errorcluster, "ref out"=w641:T8)  [unwired: 2 in, 1 out]
            n252 = xnode "H5Awrite.xnode"("object name"=w626, "error in (no error)"=w639, "data"=w635, "attrib name"="Z", "ref in"=w641) -> ("error out"=w630:errorcluster, "ref out"=w629:T8)  [unwired: 2 in, 1 out]
            n253 = xnode "H5Awrite.xnode"("object name"=w626, "error in (no error)"=w630, "data"=w624, "attrib name"="integrationTime", "ref in"=w629) -> ("error out"=w627:errorcluster, "ref out"=w628:T8)  [unwired: 2 in, 1 out]
          }
          frame False {
            w745 = ""
            # "dims: z, y, x, spec"
            n254 = Unbundle(w738) -> ("dim1"=w735:sgl[], "dim2"=w736:sgl[], "dim3"=w737:sgl[])
            n255 = Build Array(w753, w752, w751, u16 1 ("element")) -> (w750:u16[])
            n256 = Initialize Array(u16 0 ("element"), u32 1 ("dimension size"), w752, w751, 1 ("dimension size")) -> (w754:u16[][][][])
            n257 = call <vilib>:"H5Fopen.vi"("mode (read-only)"=H5Fmode."overwrite" ("mode"), "path"=w758) -> ("error out"=w757:errorcluster, "ref out"=w755:T8)  [unwired: 8 in]
            n258 = Array Size(array=w754) -> (size(s)=w749:i32[])
            n259 = call <vilib>:"H5Dcreate_simple.vi"("max size"=w750, "chunk size"=w749, "initial size"=w749, "error in (no error)"=w757, "type in"=w754, "name"="data", "ref in"=w755) -> ("error out"=w739:errorcluster, "dset out"=w740:T8)  [unwired: 3 in]
            n260 = xnode "H5Awrite.xnode"("object name"=w745, "error in (no error)"=w739, "data"=w735, "attrib name"="X", "ref in"=w740) -> ("error out"=w742:errorcluster, "ref out"=w744:T8)  [unwired: 2 in, 1 out]
            n261 = xnode "H5Awrite.xnode"("object name"=w745, "error in (no error)"=w742, "data"=w736, "attrib name"="Y", "ref in"=w744) -> ("error out"=w741:errorcluster, "ref out"=w743:T8)  [unwired: 2 in, 1 out]
            n262 = xnode "H5Awrite.xnode"("object name"=w745, "error in (no error)"=w741, "data"=w737, "attrib name"="Z", "ref in"=w743) -> ("error out"=w734:errorcluster, "ref out"=w733:T8)  [unwired: 2 in, 1 out]
          }
        }
        n263 = case shown="Error" w608 {
          selector: w608 -> [w823 w843]
          tunnel: w596 -> [w835 w847]
          tunnel: [w834 w847] -> w620
          tunnel: w618 -> [w833 _]
          tunnel: w607 -> [w827 w844]
          tunnel: w617 -> [w830 _]
          tunnel: w613 -> [w829 _]
          tunnel: w612 -> [w828 _]
          tunnel: w606 -> [w822 _]
          tunnel: w599 -> [w826 _]
          tunnel: w610 -> [_ w846]
          tunnel: w600 -> [w819 _]
          frame No Error {
            n264 = Unbundle By Name(w822) -> ("Name"=w821:string)
            n265 = Bundle By Name(cluster=w835, "ish5FileOpen?"=TRUE, "h5File_refOut"=w833, "h5File_dsetOut"=w827, "h5FileError"=w823, "scanIndex"=cluster{"X":u16, "Y":u16, "Z":u16} {"X"=0, "Y"=0, "Z"=0}, "instrDataPageSize"=w829, "instrDataPage"=w830, "scanData"=w828, "scanSpeed"=u16 500, "currentStep"=u32 0, "totalSteps"=w819, "scanIncrementDir"=cluster{"xFwd?":i16, "yFwd?":i16, "zFwd?":i16} {"xFwd?"=1, "yFwd?"=1, "zFwd?"=1}, "scan?"=TRUE) -> (w834:T5)
            n266 = case shown="Default" w821 {
              tunnel: w826 -> [w836 w840]
              tunnel: [w836 w839] -> w825
              tunnel: w822 -> [_ w837]
              frame "" {
              }
              frame Default {
                n267 = call-poly "Enqueue Message.vi"("Message Data"=w837, "Message"="saveInstrConstData", "Message Queue"=w840) -> ("dup Message Queue"=w839:refnum<queue>)  [unwired: 7 in, 1 out]
              }
            }
            n268 = call-poly "Enqueue Message.vi"("Message"="incrementScan", "Message Queue"=w825) -> ()  [unwired: 8 in, 2 out]
          }
          frame Error {
            n269 = call <vilib>:"H5Fclose.vi"("error in (no error)"=w843, "ref"=w844) -> ("error out"=w842:errorcluster)  [unwired: 9 in]
            n270 = Merge Errors(w842) -> (w841:errorcluster)
            n271 = call-poly "Enqueue Message.vi"("Message Data"=w841, "Message"="scanEnded", "Message Queue"=w846) -> ()  [unwired: 7 in, 2 out]
          }
        }
      }
      frame "saveInstrConstData" {
        n272 = Variant To Data(error in=w858, type=T7 {"Name"="", "VISAname"="", "1D_dataArraySize"=0, "extraInfo"=variant, "error"={"status"=FALSE, "code"=0, "source"=""}} ("scanInstrumentInfo"), Variant=w857) -> (data=w855:T7)  [unwired: 1 out]
        n273 = Unbundle(w855) -> ("Name"=w854:string, "VISAname"=w853:refnum<visa-resource-name>, "1D_dataArraySize"=w852:u16)  [unwired: 2 out]
        n274 = case shown="\"USB2000p\"" w854 {
          tunnel: w853 -> [_ w868]
          tunnel: w852 -> [_ w869]
          tunnel: w851 -> [w859 w864]
          tunnel: w850 -> [_ w861]
          tunnel: [w859 w860] -> w849
          frame Default {
          }
          frame "USB2000p" {
            n275 = Unbundle By Name(w864) -> ("h5File_dsetOut"=w867:T8, "h5FileError"=w865:errorcluster)
            n276 = call <instrlib>:"Calculate Wavelength.vi"("Number of Pixels (3648)"=w869, "VISA resource name"=w868) -> ("error out"=w862:errorcluster, "Wavelength (nm)"=w866:dbl[])  [unwired: 1 in, 7 out]
            n277 = case shown="No Error" w862 {
              tunnel: w867 -> [w873 _]
              tunnel: w866 -> [w872 _]
              tunnel: w865 -> [w871 w897]
              tunnel: [w870 w897] -> w863
              tunnel: w861 -> [_ w894]
              frame No Error {
                n278 = xnode "H5Awrite.xnode"("object name"="", "error in (no error)"=w871, "data"=w872, "attrib name"="Wavelengths", "ref in"=w873) -> ("error out"=w870:errorcluster)  [unwired: 2 in, 2 out]
              }
              frame Error {
                n279 = call-poly "Enqueue Message.vi"("Message Data"="Error! Unable to acquire the wavelength data from the spectrometer!\n\nThe scan will still continue though." ("Message"), "Message"="messageFromEquipLoop", "Message Queue"=w894) -> ()  [unwired: 7 in, 2 out]
              }
            }
            n280 = Bundle By Name(cluster=w864, "h5FileError"=w863) -> (w860:T5)
          }
        }
      }
      frame "incrementScan" {
        n281 = Unbundle By Name(w907) -> ("scan?"=w898:bool, "scanData"=w905:T6, "pBot_VISA"=w912:refnum<visa-resource-name>, "disconnectPBot_Event"=w911:refnum<user-event>, "scanData.scanPoints"=w913:T19, "scanIndex"=w899:cluster{"X":u16, "Y":u16, "Z":u16}, "scanSpeed"=w910:u16, "scanIncrementDir"=w901:cluster{"xFwd?":i16, "yFwd?":i16, "zFwd?":i16}, "currentStep"=w909:u32, "scanData.N"=w908:cluster{"X":u16, "Y":u16, "Z":u16}, "totalSteps"=w900:u32)
        n282 = case shown="True" w898 {
          tunnel: w913 -> [_ w950]
          tunnel: w912 -> [_ w939]
          tunnel: w911 -> [_ w916]
          tunnel: w910 -> [_ w936]
          tunnel: w909 -> [_ w935]
          tunnel: w908 -> [_ w933]
          tunnel: w907 -> [w914 w925]
          tunnel: w906 -> [_ w924]
          tunnel: w905 -> [_ w923]
          tunnel: [w914 w921] -> w904
          tunnel: w902 -> [_ w920]
          tunnel: w901 -> [_ w919]
          tunnel: w900 -> [_ w918]
          tunnel: w899 -> [_ w917]
          frame False {
          }
          frame True {
            n283 = Unbundle By Name(w923) -> ("scanInstrumentInfo.Name"=w922:string)
            n284 = To Unsigned Long Integer(number=w933) -> (unsigned 32bit integer=w932:cluster{"X":u32, "Y":u32, "Z":u32})
            n285 = Unbundle(w932) -> ("X"=w929:u32, "Y"=w931:u32, "Z"=w930:u32)
            n286 = Unbundle(w950) -> ("dim1"=w949:sgl[], "dim2"=w948:sgl[], "dim3"=w947:sgl[])
            n287 = Unbundle(w917) -> ("X"=w946:u16, "Y"=w945:u16, "Z"=w944:u16)
            n288 = Multiply(x=w929, y=w931) -> (x*y=w928:u32)
            n289 = Multiply(x=w928, y=w930) -> (x*y=w927:u32)
            n290 = Index Array(array=w949, index=w946) -> (element=w943:sgl)
            n291 = Index Array(array=w948, index=w945) -> (element=w942:sgl)
            n292 = Index Array(array=w947, index=w944) -> (element=w941:sgl)
            n293 = Build Array(w929, w928, w927) -> (w926:u32[])
            n294 = Format Into String(format string="G1 X%0.3f Y%0.3f Z%0.3f F%u", w943, w942, w941, w936) -> (resulting string=w938:string)  [unwired: 2 in, 1 out]
            n295 = Increment(x=w935) -> (x+1=w934:u32)
            n296 = call "visaQuery.vi"("disconnectPBot_Event"=w916, "stringToWrite"=w938, "VISA resource name"=w939) -> ("error Out"=w937:errorcluster, "dub: VISA resource name"=w915:refnum<visa-resource-name>)  [unwired: 6 in, 1 out]
            n297 = case shown="No Error" w937 {
              tunnel: w919 -> [w958 _]
              tunnel: w917 -> [w954 _]
              tunnel: w934 -> [w956 _]
              tunnel: w926 -> [w963 _]
              tunnel: w925 -> [w962 w1066]
              tunnel: w924 -> [w959 w1065]
              tunnel: w922 -> [w960 _]
              tunnel: [w961 w1066] -> w921
              tunnel: w920 -> [w957 _]
              tunnel: w918 -> [w955 _]
              tunnel: w916 -> [w952 _]
              tunnel: w915 -> [w951 _]
              frame No Error {
                n298 = call "pBot_waitForMoveFinish.vi"("disconnectPBot_Event"=w952, "pBot_VISA"=w951) -> ("errorOut"=w953:errorcluster)  [unwired: 8 in, 1 out]
                n299 = case shown="No Error" w953 {
                  tunnel: w963 -> [w983 _]
                  tunnel: w962 -> [w980 w1060]
                  tunnel: [w979 w1060] -> w961
                  tunnel: w960 -> [w978 _]
                  tunnel: w959 -> [w977 w1061]
                  tunnel: w958 -> [w974 _]
                  tunnel: w957 -> [w968 _]
                  tunnel: w956 -> [w967 _]
                  tunnel: w955 -> [w966 _]
                  tunnel: w954 -> [w964 _]
                  frame No Error {
                    n300 = Quotient & Remainder(x=w967, y=w983) -> (x-y*floor(x/y)=w981:u32[])  [unwired: 1 out]
                    n301 = Equal?(x=w981, y=u32 0) -> (x = y?=w970:bool[])
                    n302 = Boolean Array To Number(Boolean array=w970) -> (number=w969:u32)
                    n303 = case shown="0" w969 {
                      tunnel: w964 -> [w989 w1006 w1026 w1037 w1041]
                      tunnel: w974 -> [w988 w1007 w1027 w1038 w1042]
                      tunnel: [w987 w1004 w1024 w1037 w1041] -> w972
                      tunnel: [w986 w1005 w1025 w1038 w1042] -> w973
                      tunnel: [FALSE FALSE FALSE TRUE FALSE] -> w971
                      tunnel: w968 -> [_ w1002 w1022 _ _]
                      tunnel: w967 -> [_ w1000 w1019 _ _]
                      tunnel: w966 -> [_ w999 w1018 _ _]
                      tunnel: [FALSE FALSE TRUE TRUE FALSE] -> w965
                      frame 0 {
                        # "None of the axis are at a turning point -- increment the first dimension"
                        n304 = in-place {
                          n305 = in-place-cluster #1(w988) -> ("xFwd?"=w990:i16)
                          n306 = in-place-cluster #2(w989) -> ("X"=w992:u16)
                          n307 = Add(x=w990, y=w992) -> (x+y=w991:u16)
                          n308 = in-place-cluster #1("xFwd?"=w990) -> (w986:cluster{"xFwd?":i16, "yFwd?":i16, "zFwd?":i16})
                          n309 = in-place-cluster #2("X"=w991) -> (w987:cluster{"X":u16, "Y":u16, "Z":u16})
                        }
                      }
                      frame 1 {
                        # "the first dimension is at a turning point. reverse the increment value of the first dimension and increment the second dimension"
                        n310 = in-place {
                          n311 = in-place-cluster #3(w1007) -> ("xFwd?"=w1012:i16, "yFwd?"=w1008:i16)
                          n312 = in-place-cluster #4(w1006) -> ("Y"=w1010:u16)
                          n313 = Negate(x=w1012) -> (-x=w1011:i16)
                          n314 = Add(x=w1008, y=w1010) -> (x+y=w1009:u16)
                          n315 = in-place-cluster #3("xFwd?"=w1011, "yFwd?"=w1008) -> (w1005:cluster{"xFwd?":i16, "yFwd?":i16, "zFwd?":i16})
                          n316 = in-place-cluster #4("Y"=w1009) -> (w1004:cluster{"X":u16, "Y":u16, "Z":u16})
                        }
                        n317 = Divide(x=w1000, y=w999) -> (x/y=w997:dbl)
                        n318 = Multiply(x=w997, y=100.0) -> (x*y=w993:dbl)
                        n319 = Format Into String(format string="...%0.2f%%...", w993) -> (resulting string=w995:string)  [unwired: 2 in, 1 out]
                        n320 = call-poly "Enqueue Message.vi"("Message Data"=w995, "Message"="messageFromEquipLoop", "Message Queue"=w1002) -> ()  [unwired: 7 in, 2 out]
                      }
                      frame 3 {
                        # "the first and second dimensions are at a turning points. reverse the increment value of the first and second dimension and increment the third dimension"
                        n321 = in-place {
                          n322 = in-place-cluster #5(w1027) -> ("xFwd?"=w1034:i16, "yFwd?"=w1030:i16, "zFwd?"=w1028:i16)
                          n323 = in-place-cluster #6(w1026) -> ("Z"=w1032:u16)
                          n324 = Negate(x=w1034) -> (-x=w1033:i16)
                          n325 = Negate(x=w1030) -> (-x=w1029:i16)
                          n326 = Add(x=w1028, y=w1032) -> (x+y=w1031:u16)
                          n327 = in-place-cluster #5("xFwd?"=w1033, "yFwd?"=w1029, "zFwd?"=w1028) -> (w1025:cluster{"xFwd?":i16, "yFwd?":i16, "zFwd?":i16})
                          n328 = in-place-cluster #6("Z"=w1031) -> (w1024:cluster{"X":u16, "Y":u16, "Z":u16})
                        }
                        n329 = Divide(x=w1019, y=w1018) -> (x/y=w1016:dbl)
                        n330 = Multiply(x=w1016, y=100.0) -> (x*y=w1013:dbl)
                        n331 = Format Into String(format string="...%0.2f%%...layer finished...", w1013) -> (resulting string=w1017:string)  [unwired: 2 in, 1 out]
                        n332 = call-poly "Enqueue Message.vi"("Message Data"=w1017, "Message"="messageFromEquipLoop", "Message Queue"=w1022) -> ()  [unwired: 7 in, 2 out]
                      }
                      frame 7 {
                        # "The scan is done"
                      }
                      frame Default {
                        # "Should never happen"
                      }
                    }
                    n333 = call-poly "Enqueue Message.vi"("Message"="getCurrentInfo", "Message Queue"=w977) -> ("dup Message Queue"=w976:refnum<queue>)  [unwired: 8 in, 1 out]
                    n334 = case shown="Default" w978 {
                      selector: w978 -> [_ w1055]
                      tunnel: w976 -> [w1043 w1058]
                      tunnel: w964 -> [_ w1054]
                      tunnel: w971 -> [w1044 w1053]
                      tunnel: w965 -> [_ w1050]
                      frame "" {
                        n335 = case shown="True" w1044 {
                          tunnel: w1043 -> [w1046 w1049]
                          frame False {
                            n336 = call-poly "Enqueue Message.vi"("Message"="incrementScan", "Message Queue"=w1046) -> ()  [unwired: 8 in, 2 out]
                          }
                          frame True {
                            n337 = call-poly "Enqueue Message.vi"("Message Data"=errorcluster {"status"=FALSE, "code"=0, "source"=""} ("error out"), "Message"="scanComplete", "Message Queue"=w1049) -> ()  [unwired: 7 in, 2 out]
                          }
                        }
                      }
                      frame Default {
                        n338 = Bundle(cluster=T18 {"scanIndex"={"X"=0, "Y"=0, "Z"=0}, "scanFinished?"=FALSE, "savePageData?"=FALSE} ("output cluster"), "scanIndex"=w1054, "scanFinished?"=w1053, "savePageData?"=w1050) -> (w1052:T18)
                        n339 = Concatenate Strings("acquireScanData_" ("string"), w1055) -> (w1056:string)
                        n340 = call-poly "Enqueue Message.vi"("Message Data"=w1052, "Message"=w1056, "Message Queue"=w1058) -> ()  [unwired: 7 in, 2 out]
                      }
                    }
                    n341 = Bundle By Name(cluster=w980, "scanIncrementDir"=w973, "scanIndex"=w972, "currentStep"=w967) -> (w979:T5)
                  }
                  frame Error {
                    n342 = call-poly "Enqueue Message.vi"("Message Data"=errorcluster {"status"=TRUE, "code"=0, "source"="Error! Scan has been killed because due to an error from pBot_waitForMoveFinish. There may still be data in the file you selected."} ("error constant"), "Message"="scanComplete", "Message Queue"=w1061) -> ()  [unwired: 7 in, 2 out]
                  }
                }
              }
              frame Error {
                n343 = call-poly "Enqueue Message.vi"("Message Data"=errorcluster {"status"=TRUE, "code"=0, "source"="Error! Scan has been killed because due to an error from visaQuery. There may still be data in the file you selected."} ("error constant"), "Message"="scanComplete", "Message Queue"=w1065) -> ()  [unwired: 7 in, 2 out]
              }
            }
          }
        }
      }
      frame "acquireScanData_USB2000p" {
        n344 = Unbundle By Name(w1073) -> ("scanData.scanInstrumentInfo.VISAname"=w1076:refnum<visa-resource-name>, "integrationTime"=w1067:u32, "scan?"=w1068:bool)
        n345 = Variant To Data(error in=w1077, type=T18 {"scanIndex"={"X"=0, "Y"=0, "Z"=0}, "scanFinished?"=FALSE, "savePageData?"=FALSE} ("output cluster"), Variant=w1078) -> (data=w1074:T18, error out=w1071:errorcluster)
        n346 = case shown="True" w1068 {
          tunnel: w1076 -> [_ w1089]
          tunnel: w1074 -> [_ w1088]
          tunnel: w1073 -> [w1079 w1087]
          tunnel: [w1079 w1086] -> w1072
          tunnel: w1070 -> [_ w1085]
          tunnel: w1069 -> [_ w1084]
          tunnel: w1067 -> [_ w1081]
          frame False {
          }
          frame True {
            n347 = call "acquireSpectraWithOverSaturationProtection.vi"("default_integration_time"=w1081, "VISA_name"=w1089) -> ("error out"=w1082:errorcluster, "integration_time"=w1080:i32, "Spectrum"=w1083:dbl[])  [unwired: 7 in]
            n348 = case shown="No Error" w1082 {
              tunnel: w1088 -> [w1104 _]
              tunnel: w1087 -> [w1102 w1121]
              tunnel: [w1099 w1121] -> w1086
              tunnel: w1085 -> [w1097 w1122]
              tunnel: w1084 -> [w1095 _]
              tunnel: w1083 -> [w1090 _]
              tunnel: w1080 -> [_ _]
              frame No Error {
                n349 = To Unsigned Word Integer(number=w1090) -> (unsigned 16bit integer=w1091:u16[])
                n350 = Unbundle By Name(w1104) -> ("savePageData?"=w1093:bool, "scanFinished?"=w1092:bool, "scanIndex"=w1103:cluster{"X":u16, "Y":u16, "Z":u16})
                n351 = Unbundle(w1103) -> ("X"=w1100:u16, "Y"=w1101:u16)  [unwired: 1 out]
                n352 = in-place {
                  in-place-border: w1091 -> [w1116]
                  in-place-border: w1101 -> [w1118]
                  in-place-border: w1100 -> [w1117]
                  in-place-border: [w1115] -> w1098
                  n353 = in-place-cluster #7(w1102) -> ("instrDataPage"=w1120:u16[][][][])
                  n354 = Replace Array Subset(array=w1120, new element=w1116, index (dim 0)=0 ("disabled index (vol)"), index (dim 1)=w1118, index (dim 2)=w1117) -> (w1115:u16[][][][])  [unwired: 1 in]
                  n355 = in-place-cluster #7("instrDataPage"=w1115) -> (w1099:T5)
                }
                n356 = case shown="True" w1093 {
                  tunnel: w1098 -> [_ w1112]
                  tunnel: w1097 -> [w1110 w1113]
                  tunnel: [w1110 w1111] -> w1096
                  frame False {
                  }
                  frame True {
                    n357 = call-poly "Enqueue Message.vi"("Message Data"=w1112, "Message"="appendDataToH5File", "Message Queue"=w1113) -> ("dup Message Queue"=w1111:refnum<queue>)  [unwired: 7 in, 1 out]
                  }
                }
                n358 = case shown="True" w1092 {
                  tunnel: w1096 -> [w1106 w1108]
                  frame False {
                    n359 = call-poly "Enqueue Message.vi"("Message"="incrementScan", "Message Queue"=w1106) -> ()  [unwired: 8 in, 2 out]
                  }
                  frame True {
                    n360 = call-poly "Enqueue Message.vi"("Message Data"=errorcluster {"status"=FALSE, "code"=0, "source"=""} ("error constant"), "Message"="scanComplete", "Message Queue"=w1108) -> ()  [unwired: 7 in, 2 out]
                  }
                }
                n361 = call-poly "Enqueue Message.vi"("Message Data"=w1090, "Message"="plotData", "Message Queue"=w1095) -> ()  [unwired: 7 in, 2 out]
              }
              frame Error {
                n362 = call-poly "Enqueue Message.vi"("Message Data"=errorcluster {"status"=TRUE, "code"=0, "source"="Error! Cannot read spectrum from USB2000+. Scan has been stopped."} ("error constant"), "Message"="scanComplete", "Message Queue"=w1122) -> ()  [unwired: 7 in, 2 out]
              }
            }
          }
        }
      }
      frame "appendDataToH5File" {
        n363 = Variant To Data(error in=w1132, type=u16[][][][] [], Variant=w1131) -> (data=w1129:u16[][][][], error out=w1125:errorcluster)
        n364 = Unbundle By Name(w1128) -> ("h5File_dsetOut"=w1135:T8, "instrDataPageSize"=w1134:i32[], "h5FileError"=w1133:errorcluster)
        n365 = call <vilib>:"H5Dprepare_append.vi"("error in (no error)"=w1133, "append dims"=w1134, "dset in"=w1135) -> ("error out"=w1136:errorcluster, "space out"=w1139:T8, "dset out"=w1137:T8)  [unwired: 6 in]
        n366 = xnode "H5Dwrite.xnode"("error in (no error)"=w1136, "data"=w1129, "file space"=w1139, "ref in"=w1137) -> ("error out"=w1138:errorcluster)  [unwired: 3 in, 2 out]
        n367 = call <vilib>:"H5Sclose.vi"("error in (no error)"=w1138, "space in"=w1139) -> ("error out"=w1127:errorcluster)  [unwired: 9 in]
        n368 = Bundle By Name(cluster=w1128, "h5FileError"=w1127) -> (w1126:T5)
      }
      frame "closeH5File" {
        n369 = Unbundle By Name(w1161) -> ("h5File_refOut"=w1164:T8, "h5FileError"=w1163:errorcluster)
        n370 = call <vilib>:"H5Fclose.vi"("error in (no error)"=w1163, "ref"=w1164) -> ("error out"=w1160:errorcluster)  [unwired: 9 in]
        n371 = Bundle By Name(cluster=w1161, "ish5FileOpen?"=FALSE, "h5FileError"=w1160) -> (w1158:T5)
      }
      frame "scanComplete" {
        n372 = Variant To Data(error in=w1171, type=errorcluster {"status"=FALSE, "code"=0, "source"=""} ("error constant"), Variant=w1170) -> (data=w1168:errorcluster, error out=w1167:errorcluster)
        n373 = call-poly "Enqueue Message.vi"("Message"="closeH5File", "Message Queue"=w1175) -> ()  [unwired: 8 in, 2 out]
        n374 = call-poly "Enqueue Message.vi"("Message Data"=w1168, "Message"="scanEnded", "Message Queue"=w1173) -> ()  [unwired: 7 in, 2 out]
        n375 = in-place {
          n376 = in-place-cluster #8(w1166) -> ()  [unwired: 1 out]
          n377 = in-place-cluster #8("scan?"=FALSE) -> (w1165:T5)
        }
      }
      frame "Exit" {
        # "stop the VI"
        # "Exit the application"
        n378 = Variant To Data(type=errorcluster {"status"=FALSE, "code"=0, "source"=""} ("error constant"), Variant=w1183) -> (data=w1181:errorcluster)  [unwired: 1 in, 1 out]
        n379 = call <vilib>:"Simple Error Handler.vi"("error in (no error)"=w1181) -> ()  [unwired: 4 in, 5 out]
        n380 = Release Queue(queue=w1179, error in (no error)=w1180) -> (error out=w1178:errorcluster)  [unwired: 1 in, 2 out]
        n381 = Merge Errors(w1178) -> (w1185:errorcluster)
      }
      frame Default {
        n382 = xnode "Error Ring"("parameter 0"=w1188) -> ("error out"=w1187:errorcluster)
      }
    }
    n383 = call "Error Handler - Message Handling Loop.vi"("error in (no error)"=w359, "Message Queue"=w360) -> ("dup error in"=w357:errorcluster)  [unwired: 8 in, 1 out]
  }
  n384 = while {
    tunnel: w3 -> [w1200]
    shift-right: [w1207] -> _
    shift-left: w14 -> [w1208]
    tunnel: w10 -> [w1205]
    tunnel: w7 -> [w1204]
    tunnel: [w1198] -> w6
    tunnel: w2 -> [w1196]
    stop <- w1206 stop-if-true
    # "UI Control Loop"
    n385 = call "Dequeue Message.vi"("error in (no error)"=w1204, "Message Queue"=w1200) -> ("error out"=w1203:errorcluster, "Message Data"=w1201:variant, "Message"=w1202:string, "dup Message Queue"=w1199:refnum<queue>)  [unwired: 6 in]
    n386 = case "Message Cases" shown="\"usb2000p_connected?\"" w1202 {
      selector: w1202 -> [_ _ _ _ _ _ _ _ _ _ _ _ _ _ _ _ _ _ _ _ _ _ _ _ _ _ _ _ _ _ _ _ _ _ _ _ _ _ w2930]
      tunnel: w1199 -> [_ _ w1216 w1355 w1456 w1478 _ w1544 w1604 w1625 w1797 _ _ _ _ _ _ _ _ _ w2136 w2261 _ w2424 _ _ _ w2571 w2619 _ _ _ _ _ _ _ w2892 w2929 _]
      tunnel: w1203 -> [w1211 w1212 w1220 w1368 w1458 w1484 w1527 w1548 w1606 w1627 w1800 w1869 w1876 w1898 w1957 w1996 w2034 w2077 w2130 w2135 w2148 w2274 w2412 w2435 w2478 w2485 w2496 w2575 w2618 w2699 w2813 w2833 w2852 w2874 w2876 w2883 w2891 w2922 _]
      tunnel: [w1209 w1214 w1222 w1369 w1464 w1488 w1529 w1554 w1614 w1634 w1701 w1868 w1876 w1904 w1957 w1996 w2034 errorcluster {"status"=FALSE, "code"=0, "source"=""} ("error out") w2130 w2135 w2141 w2282 w2410 w2425 w2473 w2480 w2491 w2562 w2617 w2699 w2795 w2826 w2852 w2871 w2876 w2877 w2889 w2925 w2931] -> w1197
      tunnel: w1208 -> [w1210 w1215 w1218 w1359 w1463 w1486 w1526 w1552 w1607 w1632 w1799 w1860 w1875 w1902 w1949 w1989 w2027 w2072 w2129 w2134 w2143 w2272 w2408 w2433 w2479 w2486 w2493 w2560 w2601 w2695 w2796 w2830 w2853 w2864 w2875 w2882 w2893 w2928 w2932]
      tunnel: [w1210 w1215 w1217 w1358 w1463 w1485 w1524 w1551 w1607 w1632 w1707 w1858 w1875 w1902 w1948 w1988 w2026 w2064 w2129 w2134 w2142 w2276 w2400 w2427 w2479 w2486 w2492 w2561 w2609 w2694 w2802 w2830 w2853 w2863 w2875 w2882 w2893 w2928 w2932] -> w1207
      tunnel: [_ _ _ _ _ _ _ _ _ _ _ _ _ _ _ _ _ _ _ _ _ _ _ _ _ _ _ _ _ _ _ _ _ _ _ _ _ TRUE _] -> w1206
      tunnel: w1201 -> [_ _ _ w1367 _ w1482 _ _ _ _ _ _ _ _ _ _ _ w2076 _ _ w2147 w2273 w2411 w2434 w2477 w2484 w2495 w2574 _ _ w2812 w2832 _ w2873 _ w2881 _ w2919 _]
      tunnel: w1205 -> [_ _ _ _ _ _ _ _ _ _ _ _ _ _ _ _ _ _ _ _ _ _ _ _ _ _ _ _ _ _ _ _ _ _ _ _ _ w2924 _]
      tunnel: w1196 -> [_ _ _ _ _ _ _ _ _ _ _ _ _ _ _ _ w2030 w2062 w2128 w2133 w2149 w2283 _ _ _ _ w2489 _ _ w2693 w2798 _ _ _ _ _ w2890 _ _]
      frame "---Copy This Frame---" {
        # "Duplicate this frame when creating new messages.  Change this comment in the duplicated frame to describe this message."
        n387 = Merge Errors(w1211) -> (w1209:errorcluster)
      }
      frame "update3DPicture" {
        # "update the 3D picture"
        n388 = invoke on="3D Picture" class="SceneGraphDisp (strict)" method="Redraw"(error in=w1212) -> (error out=w1213:errorcluster)  [unwired: 2 in, 2 out]
        n389 = Merge Errors(w1213) -> (w1214:errorcluster)
      }
      frame "addObject" {
        # "This will add an object to the breadBoard"
        n390 = stacked-sequence {
          seq-local: [_ w1256 _] -> [_ _ w1340]
          seq-local: [w1223 _ _] -> [_ _ w1326]
          seq-local: [_ w1255 _] -> [_ _ w1339]
          seq-local: [w1226 _ _] -> [_ w1254 _]
          tunnel: w1218 -> [w1224 _ _]
          tunnel: [_ _ w1338] -> w1217
          tunnel: w1216 -> [_ w1253 _]
          frame #0 {
            n391 = flat-sequence {
              tunnel: [w1235] -> w1223
              tunnel: w1224 -> [w1240]
              frame #0 {
                # "save current visual translation"
                n392 = local read "cB_visualizeXtrans"() -> (w1238:dbl)
                n393 = local read "cB_visualizeZtrans"() -> (w1237:dbl)
                n394 = local read "cB_visualizeYtrans"() -> (w1236:dbl)
                n395 = Bundle(cluster=T20 {"cB_visualizeXtrans"=0.0, "cB_visualizeZtrans"=0.0, "cB_visualizeYtrans"=0.0}, "cB_visualizeXtrans"=w1238, "cB_visualizeZtrans"=w1237, "cB_visualizeYtrans"=w1236) -> (w1235:T20)
              }
              frame #1 {
                # "reset any visual translation"
                n396 = Unbundle By Name(w1240) -> ("3DPictureObjRef"=w1246:refnum<vi>, "yPOI"=w1239:cluster{"X":dbl, "Y":dbl, "Z":dbl}, "yPOI_0"=w1249:cluster{"X":dbl, "Y":dbl, "Z":dbl}, "breadBoard_00"=w1252:cluster{"X":dbl, "Y":dbl, "Z":dbl})
                n397 = Subtract(x=w1239, y=w1249) -> (x-y=w1244:cluster{"X":dbl, "Y":dbl, "Z":dbl})
                n398 = Negate(x=w1239) -> (-x=w1250:cluster{"X":dbl, "Y":dbl, "Z":dbl})
                n399 = Add(x=w1250, y=w1252) -> (x+y=w1251:cluster{"X":dbl, "Y":dbl, "Z":dbl})
                n400 = call <vilib>:"Find Object.vi"("Object Name"="yArm", "Scene Refnum"=w1246) -> ("Object Refnum"=w1248:refnum<vi>)  [unwired: 8 in, 1 out]
                n401 = call "translateObj.vi"("POI_proj_Offset (0,0,0)"=w1251, "vector"=w1244, "Type"="ta", "Scene: Object"=w1248) -> ()  [unwired: 6 in, 2 out]
                n402 = Unbundle(w1244) -> ("X"=w1242:dbl, "Y"=w1243:dbl, "Z"=w1241:dbl)
                n403 = local write "cB_visualizeXtrans"(w1242) -> ()
                n404 = local write "cB_visualizeZtrans"(w1243) -> ()
                n405 = local write "cB_visualizeYtrans"(w1241) -> ()
              }
            }
            n406 = local read "numberOfCommandLines"() -> (w1232:i32)
            n407 = local write "cB_addObject"(FALSE ("cB_addObject")) -> ()
            n408 = call "setCommandString.vi"("addLF? (T)"=FALSE, "addTimeAndChevron? (T)"=TRUE ("addTimeAndChevron?"), "numLines"=w1232, "stringToAdd"="Adding object....", "UI Data In"=w1224) -> ("error out"=w1227:errorcluster, "UI Data Out"=w1226:T9, "outputCommandString"=w1230:string)  [unwired: 4 in]
            n409 = property on="cB_commandLog" class="Str"(error in=w1227, "Text.Scroll Position"=inf) -> ()  [unwired: 1 in, 2 out]
            n410 = local write "cB_commandLog"(w1230) -> ()
          }
          frame #1 {
            n411 = Unbundle By Name(w1254) -> ("addedObjs"=w1258:T1[], "3DPictureObjRef"=w1259:refnum<vi>, "availableObjs"=w1262:T1[], "objectNames"=w1264:string[], "yPOI_Added?"=w1260:bool, "breadBoard_00"=w1257:cluster{"X":dbl, "Y":dbl, "Z":dbl})
            n412 = property on="availibleObjectNames" class="CmbBox"() -> ("Value"=w1263:string)  [unwired: 2 in, 2 out]
            n413 = Search 1D Array(1D array=w1264, element=w1263) -> (index of element=w1261:i32)  [unwired: 1 in]
            n414 = case shown="False" w1260 {
              tunnel: w1262 -> [w1286 w1307]
              tunnel: w1261 -> [w1287 w1306]
              tunnel: w1254 -> [w1281 w1310]
              tunnel: [w1283 w1309] -> w1255
              tunnel: w1259 -> [w1284 w1308]
              tunnel: w1258 -> [w1285 w1305]
              tunnel: w1257 -> [w1280 _]
              tunnel: ["" w1304] -> w1256
              tunnel: w1253 -> [w1265 _]
              frame False {
                n415 = local read "objCol_deSel"() -> (w1288:T2)
                n416 = call "addObjToPlasmaBot.vi"("deselectedColor"=w1288, "homePos_Offset"=w1280, "index"=w1287, "array"=w1286, "3DpictureRefrenceIn"=w1284) -> ("addedObject"=w1279:T1)  [unwired: 3 in, 2 out]
                n417 = Build Array (concatenate)(w1285, w1279) -> (w1275:T1[])
                n418 = Unbundle By Name(w1279) -> ("posOffset"=w1269:cluster{"X":dbl, "Y":dbl, "Z":dbl}, "mountOn"=w1267:enum16{"yArm", "breadBoard"}, "hasPOI?"=w1272:bool, "POI"=w1276:cluster{"X":dbl, "Y":dbl, "Z":dbl})
                n419 = Equal?(x=w1267, y=enum16{"yArm", "breadBoard"}."yArm") -> (x = y?=w1271:bool)
                n420 = Format Into String(w1267) -> (resulting string=w1266:string)  [unwired: 3 in, 1 out]
                n421 = And(x=w1271, y=w1272) -> (x .and. y?=w1270:bool)
                n422 = call <vilib>:"Find Object.vi"("Object Name"=w1266, "Scene Refnum"=w1284) -> ("error out"=w1277:errorcluster, "Object Refnum"=w1278:refnum<vi>)  [unwired: 8 in]
                n423 = call <vilib>:"Get Translation.vi"("error in (no error)"=w1277, "Scene Object"=w1278) -> ("Transformation:Get Translation"=w1274:cluster{"X":sgl, "Y":sgl, "Z":sgl})  [unwired: 7 in, 2 out]
                n424 = case shown="True" w1270 {
                  tunnel: w1276 -> [_ w1293]
                  tunnel: w1269 -> [_ w1298]
                  tunnel: w1274 -> [_ w1297]
                  tunnel: w1281 -> [w1289 w1296]
                  tunnel: [w1289 w1294] -> w1273
                  tunnel: w1265 -> [_ w1292]
                  frame False {
                  }
                  frame True {
                    n425 = Add(x=w1298, y=w1293) -> (x+y=w1290:cluster{"X":dbl, "Y":dbl, "Z":dbl})
                    n426 = Add(x=w1297, y=w1290) -> (x+y=w1295:cluster{"X":dbl, "Y":dbl, "Z":dbl})
                    n427 = Bundle By Name(cluster=w1296, "yPOI"=w1295, "yPOI_0"=w1290) -> (w1294:T9)
                    n428 = call-poly "Enqueue Message.vi"("Message"="updateScanRegion", "Message Queue"=w1292) -> ()  [unwired: 8 in, 2 out]
                  }
                }
                n429 = Bundle By Name(cluster=w1273, "yPOI_Added?"=w1270, "addedObjs"=w1275) -> (w1283:T9)
              }
              frame True {
                n430 = Index Array(array=w1307, index=w1306) -> (element=w1311:T1)
                n431 = Unbundle By Name(w1311) -> ("mountOn"=w1303:enum16{"yArm", "breadBoard"}, "hasPOI?"=w1300:bool)
                n432 = Equal?(x=enum16{"yArm", "breadBoard"}."yArm", y=w1303) -> (x = y?=w1301:bool)
                n433 = And(x=w1301, y=w1300) -> (x .and. y?=w1302:bool)
                n434 = case shown="False" w1302 {
                  tunnel: w1310 -> [w1317 w1323]
                  tunnel: [w1316 w1323] -> w1309
                  tunnel: w1308 -> [w1315 _]
                  tunnel: w1307 -> [w1320 _]
                  tunnel: w1306 -> [w1319 _]
                  tunnel: w1305 -> [w1318 _]
                  tunnel: ["" "Error! There is already an object added to the yArm that has a pointOfInterest. Only one object with a pointOfInterest can be added to the yArm. Remove the first object before trying to add a second. (Select and hit the delete key.)" ("stringToAdd")] -> w1304
                  frame False {
                    n435 = local read "objCol_deSel"() -> (w1321:T2)
                    n436 = call "addObjToPlasmaBot.vi"("deselectedColor"=w1321, "index"=w1319, "array"=w1320, "3DpictureRefrenceIn"=w1315) -> ("addedObject"=w1314:T1)  [unwired: 4 in, 2 out]
                    n437 = Build Array (concatenate)(w1318, w1314) -> (w1312:T1[])
                    n438 = Bundle By Name(cluster=w1317, "addedObjs"=w1312) -> (w1316:T9)
                  }
                  frame True {
                  }
                }
              }
            }
          }
          frame #2 {
            n439 = Unbundle By Name(w1339) -> ("3DPictureObjRef"=w1330:refnum<vi>, "yPOI_0"=w1325:cluster{"X":dbl, "Y":dbl, "Z":dbl}, "breadBoard_00"=w1328:cluster{"X":dbl, "Y":dbl, "Z":dbl})  [unwired: 2 out]
            n440 = Add(x=w1326, y=w1325) -> (x+y=w1324:cluster{dbl, dbl, dbl})
            n441 = call <vilib>:"Find Object.vi"("Object Name"="yArm", "Scene Refnum"=w1330) -> ("Object Refnum"=w1332:refnum<vi>)  [unwired: 8 in, 1 out]
            n442 = Negate(x=w1324) -> (-x=w1329:cluster{dbl, dbl, dbl})
            n443 = Add(x=w1329, y=w1328) -> (x+y=w1327:cluster{dbl, dbl, dbl})
            n444 = Unbundle(w1326) -> ("cB_visualizeXtrans"=w1336:dbl, "cB_visualizeZtrans"=w1334:dbl, "cB_visualizeYtrans"=w1335:dbl)
            n445 = call "translateObj.vi"("POI_proj_Offset (0,0,0)"=w1327, "vector"=w1326, "Type"="ta", "Scene: Object"=w1332) -> ()  [unwired: 6 in, 2 out]
            n446 = local write "cB_visualizeXtrans"(w1336) -> ()
            n447 = local write "cB_visualizeZtrans"(w1334) -> ()
            n448 = local write "cB_visualizeYtrans"(w1335) -> ()
            n449 = Empty String/Path?(string/path=w1340) -> (empty?=w1343:bool)
            n450 = Select(t="object added." ("stringToAdd"), s=w1343, f=w1340) -> (s? t:f=w1341:string)
            n451 = local read "numberOfCommandLines"() -> (w1349:i32)
            n452 = call "setCommandString.vi"("addTab? (F)"=FALSE, "addLF? (T)"=TRUE ("addLF?"), "addTimeAndChevron? (T)"=FALSE ("addTimeAndChevron?"), "numLines"=w1349, "stringToAdd"=w1341, "UI Data In"=w1339) -> ("error out"=w1344:errorcluster, "UI Data Out"=w1338:T9, "outputCommandString"=w1347:string)  [unwired: 3 in]
            n453 = local write "cB_commandLog"(w1347) -> ()
            n454 = property on="cB_commandLog" class="Str"(error in=w1344, "Text.Scroll Position"=inf) -> ()  [unwired: 1 in, 2 out]
          }
        }
        n455 = call-poly "Enqueue Message.vi"("error in (no error)"=w1220, "Message"="update3DPicture", "Message Queue"=w1216) -> ("error out"=w1221:errorcluster)  [unwired: 7 in, 1 out]
        n456 = Merge Errors(w1221) -> (w1222:errorcluster)
      }
      frame "selectObject" {
        # "There was a click in the 3D picture. This will determin if an added object was selected, and if it was it will place it in the selectedObject (overwriting any previously selected object)"
        n457 = property on="3D Picture" class="SceneGraphDisp (strict)"() -> ("Position"=w1364:T23)  [unwired: 2 in, 2 out]
        n458 = Variant To Data(error in=w1368, type=T14 {"Horizontal"=0, "Vertical"=0} ("Coords"), Variant=w1367) -> (data=w1365:T14, error out=w1356:errorcluster)
        n459 = Unbundle By Name(w1359) -> ("addedObjs"=w1361:T1[], "selectedObj"=w1360:T1)
        n460 = Subtract(x=w1365, y=w1364) -> (x-y=w1362:T14)
        n461 = invoke on="3D Picture" class="SceneGraphDisp (strict)" method="PickPoint"("PickPoint"=w1362) -> ("PickPoint"=→"PickPoint":T3, "Hit"=w1363:bool)  [unwired: 4 in, 3 out]
        n462 = call-poly "Enqueue Message.vi"("error in (no error)"=w1356, "Message"="update3DPicture", "Message Queue"=w1355) -> ("error out"=w1353:errorcluster, "dup Message Queue"=w1351:refnum<queue>)  [unwired: 7 in]
        n463 = case shown="True" w1363 {
          tunnel: w1362 -> [_ w1389]
          tunnel: w1361 -> [_ w1385]
          tunnel: w1360 -> [w1373 w1384]
          tunnel: w1359 -> [w1372 w1383]
          tunnel: [w1370 w1382] -> w1358
          frame False {
            n464 = Unbundle By Name(w1373) -> ("referenceNum"=w1374:refnum<vi>, "Name"=w1377:string)
            n465 = local read "emptyObj"() -> (w1371:T1)
            n466 = Equal?(x=w1377, y="") -> (x = y?=w1375:bool)
            n467 = Bundle By Name(cluster=w1372, "selectedObj"=w1371) -> (w1370:T9)
            n468 = case shown="False" w1375 {
              tunnel: w1374 -> [w1381 _]
              frame False {
                n469 = local read "objCol_deSel"() -> (w1378:T2)
                n470 = call <vilib>:"Find Object.vi"("Object Name"="boundingBox", "Scene Refnum"=w1381) -> ("Object Refnum"=w1379:refnum<vi>)  [unwired: 8 in, 1 out]
                n471 = property class="SceneObject"(reference=w1379, "Material.Ambient"=w1378, "Material.Diffuse"=w1378, "Material.Specular"=w1378) -> ()  [unwired: 1 in, 2 out]
              }
              frame True {
              }
            }
          }
          frame True {
            n472 = invoke on="3D Picture" class="SceneGraphDisp (strict)" method="Pick Model"("Point"=w1389) -> ("Pick Model"=w1388:cluster{"Node Path":refnum<vi>[]}[])  [unwired: 3 in, 3 out]
            n473 = Index Array(array=w1388) -> (element=w1387:cluster{"Node Path":refnum<vi>[]})  [unwired: 1 in]
            n474 = Unbundle(w1387) -> ("Node Path"=w1386:refnum<vi>[])
            n475 = while {
              tunnel: w1386 -> [w1397]
              tunnel: w1385 -> [w1394]
              tunnel: w1384 -> [w1392]
              tunnel: w1383 -> [w1391]
              tunnel: [w1390] -> w1382
              i -> [w1401]
              stop <- w1393 stop-if-true
              n476 = Array Size(array=w1397) -> (size(s)=w1400:i32)
              n477 = Increment(x=w1401) -> (x+1=w1399:i32)
              n478 = Subtract(x=w1400, y=w1399) -> (x-y=w1398:i32)
              n479 = Index Array(array=w1397, index=w1398) -> (element=w1396:refnum<vi>)
              n480 = property class="SceneObject"(reference=w1396) -> ("Name"=w1395:string)  [unwired: 1 in, 2 out]
              n481 = case shown="Default" w1395 {
                selector: w1395 -> [_ w1410]
                tunnel: w1394 -> [_ w1411]
                tunnel: [FALSE TRUE] -> w1393
                tunnel: w1392 -> [_ w1407]
                tunnel: w1391 -> [w1402 w1405]
                tunnel: [w1402 w1404] -> w1390
                frame "", "boundingBox" {
                }
                frame Default {
                  n482 = call "findObj.vi"("inputObjName"=w1410, "inputObjArray"=w1411) -> ("found?"=w1408:bool, "outputObj"=w1406:T1)  [unwired: 7 in, 1 out]
                  n483 = case shown="False" w1408 {
                    tunnel: w1407 -> [w1413 w1437]
                    tunnel: w1406 -> [_ w1424]
                    tunnel: w1405 -> [w1415 w1433]
                    tunnel: [w1414 w1432] -> w1404
                    frame False {
                      n484 = Unbundle By Name(w1413) -> ("referenceNum"=w1416:refnum<vi>, "Name"=w1419:string)
                      n485 = local read "emptyObj"() -> (w1412:T1)
                      n486 = Equal?(x=w1419, y="") -> (x = y?=w1417:bool)
                      n487 = Bundle By Name(cluster=w1415, "selectedObj"=w1412) -> (w1414:T9)
                      n488 = case shown="False" w1417 {
                        tunnel: w1416 -> [w1423 _]
                        frame False {
                          n489 = local read "objCol_deSel"() -> (w1420:T2)
                          n490 = call <vilib>:"Find Object.vi"("Object Name"="boundingBox", "Scene Refnum"=w1423) -> ("Object Refnum"=w1421:refnum<vi>)  [unwired: 8 in, 1 out]
                          n491 = property class="SceneObject"(reference=w1421, "Material.Ambient"=w1420, "Material.Diffuse"=w1420, "Material.Specular"=w1420) -> ()  [unwired: 1 in, 2 out]
                        }
                        frame True {
                        }
                      }
                    }
                    frame True {
                      n492 = Unbundle By Name(w1437) -> ("referenceNum"=w1427:refnum<vi>, "Name"=w1436:string)
                      n493 = Unbundle By Name(w1424) -> ("referenceNum"=w1426:refnum<vi>, "Name"=w1430:string)
                      n494 = Equal?(x=w1430, y="") -> (x = y?=w1429:bool)
                      n495 = Equal?(x=w1436, y="") -> (x = y?=w1434:bool)
                      n496 = Equal?(x=w1426, y=w1427) -> (x = y?=w1428:bool)
                      n497 = case shown="True" w1428 {
                        tunnel: w1434 -> [w1442 _]
                        tunnel: w1427 -> [w1441 w1453]
                        tunnel: w1429 -> [w1440 _]
                        tunnel: w1426 -> [w1439 _]
                        tunnel: [w1438 w1454] -> w1425
                        tunnel: w1424 -> [w1438 _]
                        frame False {
                          n498 = case shown="False" w1440 {
                            tunnel: w1439 -> [w1446 _]
                            frame False {
                              n499 = local read "objCol_sel"() -> (w1443:T2)
                              n500 = call <vilib>:"Find Object.vi"("Object Name"="boundingBox", "Scene Refnum"=w1446) -> ("Object Refnum"=w1444:refnum<vi>)  [unwired: 8 in, 1 out]
                              n501 = property class="SceneObject"(reference=w1444, "Material.Ambient"=w1443, "Material.Diffuse"=w1443, "Material.Specular"=w1443) -> ()  [unwired: 1 in, 2 out]
                            }
                            frame True {
                            }
                          }
                          n502 = case shown="False" w1442 {
                            tunnel: w1441 -> [w1450 _]
                            frame False {
                              n503 = local read "objCol_deSel"() -> (w1447:T2)
                              n504 = call <vilib>:"Find Object.vi"("Object Name"="boundingBox", "Scene Refnum"=w1450) -> ("Object Refnum"=w1448:refnum<vi>)  [unwired: 8 in, 1 out]
                              n505 = property class="SceneObject"(reference=w1448, "Material.Ambient"=w1447, "Material.Diffuse"=w1447, "Material.Specular"=w1447) -> ()  [unwired: 1 in, 2 out]
                            }
                            frame True {
                            }
                          }
                        }
                        frame True {
                          n506 = local read "emptyObj"() -> (w1454:T1)
                          n507 = local read "objCol_deSel"() -> (w1451:T2)
                          n508 = call <vilib>:"Find Object.vi"("Object Name"="boundingBox", "Scene Refnum"=w1453) -> ("Object Refnum"=w1452:refnum<vi>)  [unwired: 8 in, 1 out]
                          n509 = property class="SceneObject"(reference=w1452, "Material.Ambient"=w1451, "Material.Diffuse"=w1451, "Material.Specular"=w1451) -> ()  [unwired: 1 in, 2 out]
                        }
                      }
                      n510 = Bundle By Name(cluster=w1433, "selectedObj"=w1425) -> (w1432:T9)
                    }
                  }
                }
              }
            }
          }
        }
        n511 = call-poly "Enqueue Message.vi"("error in (no error)"=w1353, "Message"="updateDisplay", "Message Queue"=w1351) -> ("error out"=w1352:errorcluster)  [unwired: 7 in, 1 out]
        n512 = Merge Errors(w1352) -> (w1369:errorcluster)
      }
      frame "rotateObject" {
        # "rotate selected object by 90 degrees"
        n513 = Unbundle By Name(w1463) -> ("addedObjs"=w1462:T1[], "selectedObj.Name"=w1460:string)
        n514 = case shown="Default" w1460 {
          selector: w1460 -> [w1465 _]
          tunnel: w1462 -> [w1474 _]
          frame Default {
            n515 = call "findObj.vi"("inputObjName"=w1465, "inputObjArray"=w1474) -> ("outputObj"=w1473:T1)  [unwired: 7 in, 2 out]
            n516 = Unbundle By Name(w1473) -> ("referenceNum"=w1471:refnum<vi>, "posOffset"=w1466:cluster{"X":dbl, "Y":dbl, "Z":dbl})
            n517 = Negate(x=w1466) -> (-x=w1472:cluster{"X":dbl, "Y":dbl, "Z":dbl})
            n518 = call <vilib>:"Translate Object.vi"("Translation"=w1472, "Scene.Object In"=w1471) -> ("Scene.Object Out"=w1468:refnum<vi>)  [unwired: 8 in, 1 out]
            n519 = call <vilib>:"Rotate Object.vi"("Angle"=1.5707963267948966, "Axis"=cluster{"X":sgl, "Y":sgl, "Z":sgl} {"X"=0.0, "Y"=1.0, "Z"=0.0}, "Scene.Object In"=w1468) -> ("Scene.Object Out"=w1467:refnum<vi>)  [unwired: 7 in, 1 out]
            n520 = call <vilib>:"Translate Object.vi"("Translation"=w1466, "Scene.Object In"=w1467) -> ()  [unwired: 8 in, 2 out]
          }
          frame "" {
          }
        }
        n521 = call-poly "Enqueue Message.vi"("error in (no error)"=w1458, "Message"="update3DPicture", "Message Queue"=w1456) -> ("error out"=w1457:errorcluster)  [unwired: 7 in, 1 out]
        n522 = local write "cB_rotate"(FALSE ("cB_rotate")) -> ()
        n523 = Merge Errors(w1457) -> (w1464:errorcluster)
      }
      frame "translateObj" {
        w1480 = FALSE ("cB_rotate")
        # "translate selected object"
        n524 = Unbundle By Name(w1486) -> ("addedObjs"=w1487:T1[], "selectedObj.Name"=w1475:string)
        n525 = Variant To Data(error in=w1484, type=cluster{"X":dbl, "Y":dbl, "Z":dbl} {"X"=0.0, "Y"=0.0, "Z"=0.0} ("currentCenter"), Variant=w1482) -> (data=w1481:cluster{"X":dbl, "Y":dbl, "Z":dbl}, error out=w1479:errorcluster)
        n526 = local write "cB_translateForward"(w1480) -> ()
        n527 = local write "cB_translateLeft"(w1480) -> ()
        n528 = local write "cB_translateRight"(w1480) -> ()
        n529 = local write "cB_translateBack"(w1480) -> ()
        n530 = local write "cB_translateUp"(w1480) -> ()
        n531 = local write "cB_translateDown"(w1480) -> ()
        n532 = case shown="Default" w1475 {
          selector: w1475 -> [w1489 _]
          tunnel: w1487 -> [w1503 _]
          tunnel: w1486 -> [w1494 w1522]
          tunnel: [w1501 w1522] -> w1485
          tunnel: w1481 -> [w1491 _]
          frame Default {
            n533 = call "findObj.vi"("inputObjName"=w1489, "inputObjArray"=w1503) -> ("index"=w1506:i32, "outputObj"=w1505:T1)  [unwired: 7 in, 1 out]
            n534 = Unbundle By Name(w1505) -> ("mountOn"=w1493:enum16{"yArm", "breadBoard"}, "referenceNum"=w1497:refnum<vi>, "posOffset"=w1507:cluster{"X":dbl, "Y":dbl, "Z":dbl})
            n535 = Equal?(x=enum16{"yArm", "breadBoard"}."yArm", y=w1493) -> (x = y?=w1492:bool)
            n536 = case shown="True" w1492 {
              tunnel: [w1508 w1512] -> w1500
              tunnel: w1494 -> [w1508 w1510]
              tunnel: w1491 -> [_ w1509]
              frame False {
              }
              frame True {
                n537 = Unbundle By Name(w1510) -> ("yPOI_0"=w1515:cluster{"X":dbl, "Y":dbl, "Z":dbl}, "yPOI"=w1514:cluster{"X":dbl, "Y":dbl, "Z":dbl})
                n538 = Add(x=w1509, y=w1514) -> (x+y=w1513:cluster{"X":dbl, "Y":dbl, "Z":dbl})
                n539 = Add(x=w1509, y=w1515) -> (x+y=w1511:cluster{"X":dbl, "Y":dbl, "Z":dbl})
                n540 = Bundle By Name(cluster=w1510, "yPOI_0"=w1511, "yPOI"=w1513) -> (w1512:T9)
              }
            }
            n541 = call <vilib>:"Find Object.vi"("Object Name"="POI_proj", "Scene Refnum"=w1497) -> ("error out"=w1496:errorcluster, "Object Refnum"=w1495:refnum<vi>)  [unwired: 8 in]
            n542 = Add(x=w1491, y=w1507) -> (x+y=w1499:cluster{"X":dbl, "Y":dbl, "Z":dbl})
            n543 = case shown="No Error" w1496 {
              tunnel: w1495 -> [w1521 _]
              tunnel: w1491 -> [w1519 _]
              frame No Error {
                n544 = Unbundle By Name(w1519) -> ("Y"=w1518:dbl)
                n545 = Negate(x=w1518) -> (-x=w1517:dbl)
                n546 = Bundle By Name(cluster=cluster{"X":dbl, "Y":dbl, "Z":dbl} {"X"=0.0, "Y"=0.0, "Z"=0.0} ("currentCenter"), "Y"=w1517) -> (w1516:cluster{"X":dbl, "Y":dbl, "Z":dbl})
                n547 = call <vilib>:"Translate Object.vi"("Translation"=w1516, "Scene.Object In"=w1521) -> ()  [unwired: 8 in, 2 out]
              }
              frame Error {
              }
            }
            n548 = Bundle By Name(cluster=w1505, "posOffset"=w1499) -> (w1504:T1)
            n549 = call <vilib>:"Set Translation.vi"("Translation"=w1499, "Scene Object"=w1497) -> ()  [unwired: 8 in, 2 out]
            n550 = Replace Array Subset(array=w1503, new element=w1504, index=w1506) -> (w1502:T1[])
            n551 = Bundle By Name(cluster=w1500, "addedObjs"=w1502, "selectedObj.posOffset"=w1499) -> (w1501:T9)
          }
          frame "" {
          }
        }
        n552 = call-poly "Enqueue Message.vi"("error in (no error)"=w1479, "Message"="update3DPicture", "Message Queue"=w1478) -> ("error out"=w1477:errorcluster)  [unwired: 7 in, 1 out]
        n553 = Merge Errors(w1477) -> (w1488:errorcluster)
      }
      frame "getObjectInfo" {
        # "translate selected object"
        n554 = Unbundle By Name(w1526) -> ("selectedObj.Name"=w1523:string, "selectedObj"=w1525:T1)
        n555 = case shown="Default" w1523 {
          tunnel: w1526 -> [w1531 w1543]
          tunnel: w1525 -> [w1533 _]
          tunnel: [w1530 w1543] -> w1524
          frame Default {
            n556 = call "getPosInfo.vi"("UI_DataIn"=w1531) -> ("POI"=w1534:T3[], "extent"=w1535:T3[], "origin"=w1536:T3[])  [unwired: 7 in, 1 out]
            n557 = call "formatObjectInfo.vi"("POI"=w1534, "extent"=w1535, "origin"=w1536, "selectedObj"=w1533) -> ("displayString"=w1532:string)  [unwired: 7 in]
            n558 = local read "numberOfCommandLines"() -> (w1538:i32)
            n559 = call "setCommandString.vi"("addLF? (T)"=FALSE ("addLF?"), "addTimeAndChevron? (T)"=TRUE ("addTimeAndChevron?"), "numLines"=w1538, "stringToAdd"=w1532, "UI Data In"=w1531) -> ("error out"=w1542:errorcluster, "UI Data Out"=w1530:T9, "outputCommandString"=w1540:string)  [unwired: 4 in]
            n560 = local write "cB_commandLog"(w1540) -> ()
            n561 = property on="cB_commandLog" class="Str"(error in=w1542, "Text.Scroll Position"=inf) -> ()  [unwired: 1 in, 2 out]
          }
          frame "" {
          }
        }
        n562 = local write "cB_getObjectInfo"(FALSE ("cB_rotate")) -> ()
        n563 = Merge Errors(w1527) -> (w1529:errorcluster)
      }
      frame "deleteObject" {
        # "delete selected object"
        n564 = Unbundle By Name(w1552) -> ("3DPictureObjRef"=w1550:refnum<vi>, "addedObjs"=w1553:T1[], "selectedObj.Name"=w1545:string, "breadBoard_00"=w1546:cluster{"X":dbl, "Y":dbl, "Z":dbl})
        n565 = call-poly "Enqueue Message.vi"("error in (no error)"=w1548, "Message"="update3DPicture", "Message Queue"=w1544) -> ("error out"=w1547:errorcluster)  [unwired: 7 in, 1 out]
        n566 = case shown="Default" w1545 {
          selector: w1545 -> [w1556 _]
          tunnel: w1553 -> [w1571 _]
          tunnel: w1552 -> [w1575 w1594]
          tunnel: [w1561 w1594] -> w1551
          tunnel: w1550 -> [w1568 _]
          tunnel: w1546 -> [w1557 _]
          tunnel: w1544 -> [w1555 _]
          frame Default {
            n567 = call "findObj.vi"("inputObjName"=w1556, "inputObjArray"=w1571) -> ("index"=w1572:i32, "outputObj"=w1574:T1)  [unwired: 7 in, 1 out]
            n568 = Unbundle By Name(w1574) -> ("referenceNum"=w1569:refnum<vi>, "mountOn"=w1559:enum16{"yArm", "breadBoard"}, "hasPOI?"=w1565:bool)
            n569 = Format Into String(w1559) -> (resulting string=w1558:string)  [unwired: 3 in, 1 out]
            n570 = Equal?(x=w1559, y=enum16{"yArm", "breadBoard"}."yArm") -> (x = y?=w1566:bool)
            n571 = call <vilib>:"Find Object.vi"("Object Name"=w1558, "Scene Refnum"=w1568) -> ("Object Refnum"=w1567:refnum<vi>)  [unwired: 8 in, 1 out]
            n572 = And(x=w1565, y=w1566) -> (x .and. y?=w1564:bool)
            n573 = invoke class="SceneObject" method="Object.Remove Object"(reference=w1567, "Child"=w1569) -> (reference out=w1563:refnum<vi>)  [unwired: 2 in, 3 out]
            n574 = local read "emptyObj"() -> (w1573:T1)
            n575 = Delete From Array(array=w1571, index=w1572) -> (array with subset deleted=w1570:T1[])  [unwired: 1 in, 1 out]
            n576 = Bundle By Name(cluster=w1575, "addedObjs"=w1570, "selectedObj"=w1573) -> (w1562:T9)
            n577 = case shown="True" w1564 {
              tunnel: w1563 -> [_ w1593]
              tunnel: w1562 -> [w1576 w1592]
              tunnel: [w1576 w1590] -> w1561
              tunnel: w1557 -> [_ w1582]
              tunnel: w1555 -> [_ w1578]
              frame False {
              }
              frame True {
                n578 = local read "cB_visualizeXtrans"() -> (w1589:dbl)
                n579 = local read "cB_visualizeZtrans"() -> (w1588:dbl)
                n580 = local read "cB_visualizeYtrans"() -> (w1587:dbl)
                n581 = call <vilib>:"Get Translation.vi"("Scene Object"=w1593) -> ("Transformation:Get Translation"=w1584:cluster{"X":sgl, "Y":sgl, "Z":sgl})  [unwired: 8 in, 2 out]
                n582 = Bundle(cluster=T21 {"cB_visualizeXtrans"=0.0, "cB_visualizeYtrans"=0.0, "cB_visualizeZtrans"=0.0}, "cB_visualizeXtrans"=w1589, "cB_visualizeYtrans"=w1588, "cB_visualizeZtrans"=w1587) -> (w1585:T21)
                n583 = Subtract(x=w1584, y=w1585) -> (x-y=w1583:cluster{dbl, dbl, dbl})
                n584 = Subtract(x=w1583, y=w1582) -> (x-y=w1579:cluster{dbl, dbl, dbl})
                n585 = Subtract(x=T3 {"X"=0.0, "Y"=0.0, "Z"=0.0} ("POI_Home"), y=w1582) -> (x-y=w1580:cluster{"X":dbl, "Y":dbl, "Z":dbl})
                n586 = Bundle By Name(cluster=w1592, "yPOI_0"=w1580, "yPOI"=w1579, "yPOI_Added?"=FALSE ("POI_Added?")) -> (w1590:T9)
                n587 = call-poly "Enqueue Message.vi"("Message"="updateScanRegion", "Message Queue"=w1578) -> ()  [unwired: 8 in, 2 out]
              }
            }
          }
          frame "" {
          }
        }
        n588 = Merge Errors(w1547) -> (w1554:errorcluster)
      }
      frame "visualizeTranslation" {
        # "apply a visual translation"
        n589 = call-poly "Enqueue Message.vi"("error in (no error)"=w1606, "Message"="update3DPicture", "Message Queue"=w1604) -> ("error out"=w1605:errorcluster)  [unwired: 7 in, 1 out]
        n590 = local read "cB_visualizeXtrans"() -> (w1613:dbl)
        n591 = local read "cB_visualizeZtrans"() -> (w1612:dbl)
        n592 = local read "cB_visualizeYtrans"() -> (w1611:dbl)
        n593 = Unbundle By Name(w1607) -> ("yPOI_0"=w1595:cluster{"X":dbl, "Y":dbl, "Z":dbl}, "3DPictureObjRef"=w1609:refnum<vi>, "breadBoard_00"=w1598:cluster{"X":dbl, "Y":dbl, "Z":dbl})  [unwired: 1 out]
        n594 = Bundle(cluster=T21 {"cB_visualizeXtrans"=0.0, "cB_visualizeYtrans"=0.0, "cB_visualizeZtrans"=0.0}, "cB_visualizeXtrans"=w1613, "cB_visualizeYtrans"=w1612, "cB_visualizeZtrans"=w1611) -> (w1596:T21)
        n595 = Add(x=w1596, y=w1595) -> (x+y=w1597:cluster{dbl, dbl, dbl})
        n596 = Negate(x=w1597) -> (-x=w1600:cluster{dbl, dbl, dbl})
        n597 = Merge Errors(w1605) -> (w1614:errorcluster)
        n598 = call <vilib>:"Find Object.vi"("Object Name"="yArm", "Scene Refnum"=w1609) -> ("Object Refnum"=w1602:refnum<vi>)  [unwired: 8 in, 1 out]
        n599 = Add(x=w1600, y=w1598) -> (x+y=w1599:cluster{dbl, dbl, dbl})
        n600 = call "translateObj.vi"("POI_proj_Offset (0,0,0)"=w1599, "vector"=w1596, "Type"="ta", "Scene: Object"=w1602) -> ()  [unwired: 6 in, 2 out]
      }
      frame "revertToActualPos" {
        # "revert the visual translation back to the actual translation"
        n601 = call-poly "Enqueue Message.vi"("error in (no error)"=w1627, "Message"="update3DPicture", "Message Queue"=w1625) -> ("error out"=w1626:errorcluster)  [unwired: 7 in, 1 out]
        n602 = Unbundle By Name(w1632) -> ("3DPictureObjRef"=w1623:refnum<vi>, "yPOI"=w1615:cluster{"X":dbl, "Y":dbl, "Z":dbl}, "yPOI_0"=w1619:cluster{"X":dbl, "Y":dbl, "Z":dbl}, "breadBoard_00"=w1616:cluster{"X":dbl, "Y":dbl, "Z":dbl})
        n603 = local write "cB_revertToActualPos"(FALSE ("cB_revertToActualPos")) -> ()
        n604 = Subtract(x=w1615, y=w1619) -> (x-y=w1620:cluster{"X":dbl, "Y":dbl, "Z":dbl})
        n605 = Negate(x=w1615) -> (-x=w1618:cluster{"X":dbl, "Y":dbl, "Z":dbl})
        n606 = Add(x=w1618, y=w1616) -> (x+y=w1617:cluster{"X":dbl, "Y":dbl, "Z":dbl})
        n607 = call <vilib>:"Find Object.vi"("Object Name"="yArm", "Scene Refnum"=w1623) -> ("Object Refnum"=w1621:refnum<vi>)  [unwired: 8 in, 1 out]
        n608 = Merge Errors(w1626) -> (w1634:errorcluster)
        n609 = call "translateObj.vi"("POI_proj_Offset (0,0,0)"=w1617, "vector"=w1620, "Type"="ta", "Scene: Object"=w1621) -> ()  [unwired: 6 in, 2 out]
        n610 = Unbundle(w1620) -> ("X"=w1630:dbl, "Y"=w1628:dbl, "Z"=w1629:dbl)
        n611 = local write "cB_visualizeXtrans"(w1630) -> ()
        n612 = local write "cB_visualizeZtrans"(w1628) -> ()
        n613 = local write "cB_visualizeYtrans"(w1629) -> ()
      }
      frame "Initialize" {
        w1654 = string[] [] ("Strings []")
        w1666 = u16 11 ("pBot_scanNx")
        w1670 = sgl 0.0 ("pBot_scanningXmin")
        w1671 = sgl 1.0 ("pBot_scanningXmax")
        w1672 = TRUE ("needToHomeY?")
        w1685 = 0.0 ("pBot_tempSensor1")
        w1710 = string[] ["None"] ("Strings []")
        w1737 = string[] [] ("Strings []")
        w1636 = cluster{"X":dbl, "Y":dbl, "Z":dbl} {"X"=0.0, "Y"=0.0, "Z"=0.0} ("0 Vector")
        w1637 = cluster{"X":dbl, "Y":dbl, "Z":dbl} {"X"=25.4, "Y"=12.7, "Z"=12.7} ("breadBoardOriginOffset")
        w1739 = 1000 ("numberOfCommandLines")
        # "Location of breadboard origin in the 3D picture coordinate system."
        # "just for debugging stuff"
        # "Initialize - All initialization work should take place in this message, since other loops can potentially enqueue messages that execute immediately after this one."
        n614 = Current VI's Path() -> (path=w1781:path)
        n615 = Path To String(path=w1781) -> (string=w1780:string)
        n616 = local write "cB_plasmaBot"(TRUE ("cB_plasmaBot")) -> ()
        n617 = local write "cB_USB2000+"(FALSE ("cB_USB2000+")) -> ()
        n618 = local write "cB_3Dview"(FALSE ("cB_3Dview")) -> ()
        n619 = local write "cB_dataView"(FALSE ("cB_dataView")) -> ()
        n620 = Reverse String(1:w1780) -> (0:w1779:string)
        n621 = local write "cB_addObject"(FALSE ("cB_addObject")) -> ()
        n622 = control-ref of="3D Picture"() -> (w1760:refnum<vi>)
        n623 = property on="controlTab" class="TabCtl (strict)"("BG Color"=u32 2894892, "FG Color"=u32 131586) -> ()  [unwired: 2 in, 2 out]
        n624 = Match Pattern(string=w1779, regular expression="\\") -> (match substring=w1771:string, after substring=w1777:string)  [unwired: 1 in, 2 out]
        n625 = local write "pBot_xyMoveDisplay"("X/Y" ("pBot_xyMoveDisplay")) -> ()
        n626 = local write "pBot_zMoveDisplay"("Z" ("pBot_zMoveDisplay")) -> ()
        n627 = property on="3D Picture" class="SceneGraphDisp (strict)"("CameraController"=T25."Spherical" ("Camera Controller:Type"), "AutoProjection"=enum16{"None", "Perspective", "Orthographic"}."Perspective" ("Automatic Projection Mode"), "Background Color"=T2 {"Red"=0.0, "Green"=0.0, "Blue"=0.0, "Alpha"=0.0}) -> ()  [unwired: 2 in, 2 out]
        n628 = control-ref of="pBot_runScan"() -> (w1646:refnum<vi>)
        n629 = local write "1DdataGraph"(cluster{dbl[], dbl[]} {[], []}) -> ()
        n630 = control-ref of="pBot_sendCommand"() -> (w1734:refnum<vi>)
        n631 = control-ref of="pBot_yHome"() -> (w1733:refnum<vi>)
        n632 = control-ref of="pBot_xHome"() -> (w1732:refnum<vi>)
        n633 = control-ref of="pBot_zHome"() -> (w1731:refnum<vi>)
        n634 = control-ref of="pBot_yBack10"() -> (w1730:refnum<vi>)
        n635 = control-ref of="pBot_yBack1"() -> (w1729:refnum<vi>)
        n636 = control-ref of="pBot_yBack01"() -> (w1728:refnum<vi>)
        n637 = control-ref of="pBot_yForward01"() -> (w1727:refnum<vi>)
        n638 = control-ref of="pBot_yForward1"() -> (w1726:refnum<vi>)
        n639 = control-ref of="pBot_yForward10"() -> (w1725:refnum<vi>)
        n640 = control-ref of="pBot_xRight10"() -> (w1724:refnum<vi>)
        n641 = control-ref of="pBot_xRight1"() -> (w1723:refnum<vi>)
        n642 = control-ref of="pBot_xRight01"() -> (w1722:refnum<vi>)
        n643 = control-ref of="pBot_xLeft01"() -> (w1721:refnum<vi>)
        n644 = control-ref of="pBot_xLeft1"() -> (w1720:refnum<vi>)
        n645 = control-ref of="pBot_xLeft10"() -> (w1719:refnum<vi>)
        n646 = control-ref of="pBot_zUp10"() -> (w1718:refnum<vi>)
        n647 = control-ref of="pBot_zUp1"() -> (w1717:refnum<vi>)
        n648 = control-ref of="pBot_zUp01"() -> (w1716:refnum<vi>)
        n649 = control-ref of="pBot_zDown01"() -> (w1715:refnum<vi>)
        n650 = control-ref of="pBot_zDown1"() -> (w1714:refnum<vi>)
        n651 = control-ref of="pBot_zDown10"() -> (w1713:refnum<vi>)
        n652 = control-ref of="pBot_gcodeCommand"() -> (w1735:refnum<vi>)
        n653 = local write "controlTab"(T4."plasmaBot" ("controlTab")) -> ()
        n654 = Reverse String(1:w1777) -> (0:w1776:string)
        n655 = Concatenate Strings(w1776, w1771) -> (w1743:string)
        n656 = invoke class="SceneGraphDisp (strict)" method="Setup Camera"(reference=w1760, "Camera Position"=T3 {"X"=140.0, "Y"=350.0, "Z"=450.0}, "Target"=T3 {"X"=140.0, "Y"=100.0, "Z"=150.0}, "Up Direction"=T3 {"X"=0.0, "Y"=1.0, "Z"=0.0}) -> ()  [unwired: 2 in, 6 out]
        n657 = local write "pBot_scanNx"(w1666) -> ()
        n658 = local write "pBot_scanNy"(w1666) -> ()
        n659 = local write "pBot_scanNz"(w1666) -> ()
        n660 = call-poly <userlib>:"MGI Disable Enum (Small).vi"() -> ("Disabled & Grayed"=w1645:T22)
        n661 = control-ref of="cB_translateUp"() -> (w1752:refnum<vi>)
        n662 = control-ref of="cB_translateDown"() -> (w1753:refnum<vi>)
        n663 = control-ref of="cB_translateBack"() -> (w1754:refnum<vi>)
        n664 = control-ref of="cB_translateForward"() -> (w1757:refnum<vi>)
        n665 = control-ref of="cB_translateLeft"() -> (w1756:refnum<vi>)
        n666 = control-ref of="cB_translateRight"() -> (w1755:refnum<vi>)
        n667 = control-ref of="cB_visualizeXtrans"() -> (w1677:refnum<vi>)
        n668 = control-ref of="cB_visualizeYtrans"() -> (w1678:refnum<vi>)
        n669 = control-ref of="cB_visualizeZtrans"() -> (w1676:refnum<vi>)
        n670 = property on="3D Picture" class="SceneGraphDisp (strict)"("Visible"=TRUE) -> ()  [unwired: 2 in, 2 out]
        n671 = property on="1DdataGraph" class="XYGraph (strict)"("Visible"=FALSE) -> ()  [unwired: 2 in, 2 out]
        n672 = Build Array(TRUE ("cB_plasmaBot"), FALSE ("cB_USB2000+"), FALSE ("cB_3Dview"), FALSE ("cB_dataView")) -> (w1787:bool[])
        n673 = Concatenate Strings(w1743, "stlFiles" ("string"), w1771) -> (w1772:string)
        n674 = local write "pBot_scanningXmax"(w1671) -> ()
        n675 = local write "pBot_scanningXmin"(w1670) -> ()
        n676 = local write "pBot_scanningYmax"(w1671) -> ()
        n677 = local write "pBot_scanningYmin"(w1670) -> ()
        n678 = local write "pBot_scanningZmax"(w1671) -> ()
        n679 = local write "pBot_scanningZmin"(w1670) -> ()
        n680 = property class="Bool (strict)"(reference=w1646, "DisabledEnum"=w1645) -> ()  [unwired: 1 in, 2 out]
        n681 = String To Path(string=w1772) -> (path=w1742:path)
        n682 = Concatenate Strings(w1743, "objectInfo.ini" ("regular expression")) -> (w1774:string)
        n683 = local write "objCol_sel"(T2 {"Red"=1.0, "Green"=0.0, "Blue"=0.0, "Alpha"=1.0} ("deselectedObjCol")) -> ()
        n684 = local write "objCol_deSel"(T2 {"Red"=0.0, "Green"=1.0, "Blue"=0.0, "Alpha"=0.1} ("selectedObjCol")) -> ()
        n685 = Build Array(w1677, w1678, w1676) -> (w1675:refnum<vi>[])
        n686 = Build Array(w1754, w1757, w1756, w1755) -> (w1690:refnum<vi>[])
        n687 = Build Array(w1752, w1753) -> (w1689:refnum<vi>[])
        n688 = String To Path(string=w1774) -> (path=w1773:path)
        n689 = call-poly "Enqueue Message.vi"("error in (no error)"=w1800, "Message"="updateDisplay", "Message Queue"=w1797) -> ("error out"=w1702:errorcluster, "dup Message Queue"=w1700:refnum<queue>)  [unwired: 7 in]
        n690 = Build Array(w1735, w1734, w1733, w1732, w1731, w1730, w1729, w1728, w1727, w1726, w1725, w1724, w1723, w1722, w1721, w1720, w1719, w1718, w1717, w1716, w1715, w1714, w1713) -> (w1688:refnum<vi>[])
        n691 = call "setupScene.vi"("Model File Path"=w1742) -> ("reference out"=w1745:refnum<vi>)  [unwired: 10 in]
        n692 = call "loadObjectInfo.vi"("pathToSTLFiles"=w1742, "Path (dialog)"=w1773) -> ("error Out"=w1740:errorcluster, "availableObjects"=w1738:T1[], "objectNames"=w1766:string[])  [unwired: 7 in]
        n693 = Build Array(w1690, w1689, w1688) -> (w1687:refnum<vi>[][])
        n694 = call-poly "Enqueue Message.vi"("error in (no error)"=w1702, "Message"="testSomething", "Message Queue"=w1700) -> ("error out"=w1701:errorcluster)  [unwired: 7 in, 1 out]
        n695 = for {
          tunnel: w1687 -> [w1822] mode=indexing
          n696 = for {
            tunnel: w1822 -> [w1823] mode=indexing
            n697 = call-poly <userlib>:"MGI Disable Enum (Small).vi"() -> ("Disabled & Grayed"=w1826:T22)
            n698 = property class="Ctl"(reference=w1823, "DisabledEnum"=w1826) -> (reference out=w1824:refnum<vi>, "ClassID"=w1825:u32)  [unwired: 1 in, 1 out]
            n699 = case shown="8" w1825 {
              tunnel: w1824 -> [_ w1828]
              frame Default {
              }
              frame 8 {
                n700 = property class="Ctl"(reference=w1828, "Value"=FALSE) -> ()  [unwired: 1 in, 2 out]
              }
            }
          }
        }
        n701 = local write "3D Picture"(w1745) -> ()
        n702 = control-ref of="cB_realTimeInfoX"() -> (w1692:refnum<vi>)
        n703 = control-ref of="cB_realTimeInfoY"() -> (w1695:refnum<vi>)
        n704 = control-ref of="cB_realTimeInfoZ"() -> (w1694:refnum<vi>)
        n705 = control-ref of="cB_realTimeInfoT1"() -> (w1693:refnum<vi>)
        n706 = control-ref of="cB_realTimeInfoT2"() -> (w1686:refnum<vi>)
        n707 = Index Array(array=w1766, index=0) -> (element=w1765:string)
        n708 = local write "numberOfCommandLines"(w1739) -> ()
        n709 = control-ref of="3D Picture"() -> (w1635:refnum<vi>)
        n710 = local write "usb2000p_intTime"(u32 100 ("usb2000p_intTime")) -> ()
        n711 = local read "textColorRed"() -> (w1684:u32)
        n712 = call <vilib>:"Find Object.vi"("Object Name"="breadBoard", "Scene Refnum"=w1745) -> ("Object Refnum"=w1747:refnum<vi>)  [unwired: 8 in, 1 out]
        n713 = Build Array(w1692, w1695, w1694, w1693, w1686) -> (w1691:refnum<vi>[])
        n714 = property on="availibleObjectNames" class="CmbBox"("Strings[]"=w1766, "AllowUndefStrs"=FALSE ("Allow Undefined Strings"), "Value"=w1765) -> ()  [unwired: 2 in, 2 out]
        n715 = local read "emptyObj"() -> (w1741:T1)
        n716 = for {
          tunnel: w1675 -> [w1821] mode=indexing
          tunnel: dbl[] [285.0, 150.0, 150.0] -> [w1820] mode=indexing
          tunnel: dbl[] [0.0, 0.0, 0.0] -> [w1819] mode=indexing
          w1818 = u8 1 ("Response to Value Outside Limits:Minimum")
          n717 = property class="Knob (strict)"(reference=w1821, "Value"=0.0, "Maximum"=w1820, "Scale.Maximum"=w1820, "Scale.Minimum"=w1819, "Minimum"=w1819, "OutOfRngActMin"=w1818, "OutOfRngActMax"=w1818) -> ()  [unwired: 1 in, 2 out]
        }
        n718 = call <vilib>:"Get Translation.vi"("Scene Object"=w1747) -> ("Transformation:Get Translation"=w1639:cluster{"X":sgl, "Y":sgl, "Z":sgl})  [unwired: 8 in, 2 out]
        n719 = control-ref of="usb2000p_aquireSpectra"() -> (w1650:refnum<vi>)
        n720 = control-ref of="usb2000p_saveSpectra"() -> (w1648:refnum<vi>)
        n721 = control-ref of="usb2000p_continuous?"() -> (w1642:refnum<vi>)
        n722 = control-ref of="usb2000p_intTime"() -> (w1649:refnum<vi>)
        n723 = property on="controlPane" class="Pane"("Minimum Pane Size"=T24 {"Horizontal"=230, "Vertical"=448}) -> (error out=w1697:errorcluster)  [unwired: 2 in, 1 out]
        n724 = Add(x=w1637, y=w1639) -> (x+y=w1638:cluster{"X":dbl, "Y":dbl, "Z":dbl})
        n725 = Initialize Array(w1684, 5 ("dimension size")) -> (w1681:u32[])
        n726 = control-ref of="pBot_scanningXmin"() -> (w1664:refnum<vi>)
        n727 = control-ref of="pBot_scanningYmin"() -> (w1665:refnum<vi>)
        n728 = control-ref of="pBot_scanningZmin"() -> (w1663:refnum<vi>)
        n729 = control-ref of="pBot_scanningXmax"() -> (w1661:refnum<vi>)
        n730 = control-ref of="pBot_scanningYmax"() -> (w1662:refnum<vi>)
        n731 = control-ref of="pBot_scanningZmax"() -> (w1660:refnum<vi>)
        n732 = Build Array(w1642, w1649, w1650, w1648) -> (w1647:refnum<vi>[])
        n733 = for {
          tunnel: w1647 -> [w1803] mode=indexing
          n734 = call-poly <userlib>:"MGI Disable Enum (Small).vi"() -> ("Disabled & Grayed"=w1804:T22)
          n735 = property class="Ctl"(reference=w1803, "DisabledEnum"=w1804) -> (reference out=w1801:refnum<vi>, "ClassID"=w1802:u32)  [unwired: 1 in, 1 out]
          n736 = case shown="8" w1802 {
            tunnel: w1801 -> [_ w1806]
            frame Default {
            }
            frame 8 {
              n737 = property class="Ctl"(reference=w1806, "Value"=FALSE) -> ()  [unwired: 1 in, 2 out]
            }
          }
        }
        n738 = Build Array(w1664, w1665, w1663) -> (w1659:refnum<vi>[])
        n739 = Build Array(w1661, w1662, w1660) -> (w1658:refnum<vi>[])
        n740 = Bundle By Name(cluster=w1799, "yPOI_Added?"=FALSE ("pointOfInterestAdded?"), "yPOI"=w1636, "yPOI_0"=w1636, "breadBoardOriginOffset"=w1637, "breadBoard_00"=w1638, "3DPictureObjRef"=w1745, "objectNames"=w1766, "availableObjs"=w1738, "selectedObj"=w1741, "pathToSTLFiles"=w1742, "controlTabState"=w1787, "XYtranslateObjControls"=w1690, "ZtranslateObjControls"=w1689, "pBot_controls"=w1688, "commandLog"="", "pBotConnected?"=FALSE, "realTimeInfoControls"=w1691, "pBot_tempSensor1"=w1685, "pBot_tempSensor2"=w1685, "realTimeInfoTextColor"=w1681, "needToHomeY?"=w1672, "needToHomeXY?"=w1672, "transVisualizationControls"=w1675, "pBot_minScanRegion"=cluster{"X":sgl, "Y":sgl, "Z":sgl} {"X"=0.0, "Y"=0.0, "Z"=0.0}, "pBot_maxScanRegion"=cluster{"X":sgl, "Y":sgl, "Z":sgl} {"X"=1.0, "Y"=1.0, "Z"=1.0}, "pBot_scanN"=cluster{"X":u16, "Y":u16, "Z":u16} {"X"=11, "Y"=11, "Z"=11} ("pBot_numberScanRegionPoints"), "usb2000p_controlRefs"=w1647, "3DPictureRef"=w1635) -> (w1682:T9)
        n741 = case shown="No Error" w1740 {
          selector: w1740 -> [_ w1845]
          tunnel: w1739 -> [_ w1838]
          tunnel: w1738 -> [_ w1843]
          tunnel: w1682 -> [w1830 w1833]
          tunnel: [w1830 w1831] -> w1707
          frame No Error {
            n742 = local write "cB_commandLog"("") -> ()
          }
          frame Error {
            n743 = Unbundle(w1845) -> ("source"=w1844:string)  [unwired: 2 out]
            n744 = Array Size(array=w1843) -> (size(s)=w1840:i32)
            n745 = call "setCommandString.vi"("addLF? (T)"=TRUE ("addLF?"), "addTimeAndChevron? (T)"=TRUE ("addTimeAndChevron?"), "numLines"=w1838, "stringToAdd"=w1844, "UI Data In"=w1833) -> ("UI Data Out"=w1832:T9)  [unwired: 4 in, 2 out]
            n746 = Format Into String(format string="%d", initial string="Number of objects available to add: ", w1840) -> (resulting string=w1839:string)  [unwired: 1 in, 1 out]
            n747 = call "setCommandString.vi"("addLF? (T)"=TRUE ("addLF?"), "addTimeAndChevron? (T)"=FALSE ("addTimeAndChevron?"), "numLines"=w1838, "stringToAdd"=w1839, "UI Data In"=w1832) -> ("error out"=w1834:errorcluster, "UI Data Out"=w1831:T9, "outputCommandString"=w1835:string)  [unwired: 4 in]
            n748 = local write "cB_commandLog"(w1835) -> ()
            n749 = property on="cB_commandLog" class="Str"(error in=w1834, "Text.Scroll Position"=inf) -> ()  [unwired: 1 in, 2 out]
          }
        }
        n750 = local read "textColorGreen"() -> (w1651:u32)
        n751 = property on="pBot_ExperimentTabControl" class="TabCtl (strict)"(error in=w1697, "Position"=T23 {"Left"=0, "Top"=249}, "PaneWidth"=u32 230 ("Tab Control Pane Dimension:Width")) -> ()  [unwired: 1 in, 2 out]
        n752 = for {
          tunnel: w1659 -> [w1816] mode=indexing
          n753 = property class="DigNum (strict)"(reference=w1816, "Increment"=0.1 ("Data Entry Limits:Increment"), "OutOfRngActInc"=u8 1 ("Response to Value Outside Limits:Increment"), "Minimum"=0.0 ("Data Entry Limits:Minimum"), "OutOfRngActMin"=u8 1 ("Response to Value Outside Limits:Minimum")) -> ()  [unwired: 1 in, 2 out]
        }
        n754 = for {
          tunnel: w1658 -> [w1811] mode=indexing
          n755 = property class="DigNum (strict)"(reference=w1811, "Increment"=0.1 ("Data Entry Limits:Increment"), "OutOfRngActInc"=u8 1 ("Response to Value Outside Limits:Increment"), "Minimum"=0.0 ("Data Entry Limits:Minimum"), "OutOfRngActMin"=u8 1 ("Response to Value Outside Limits:Minimum")) -> ()  [unwired: 1 in, 2 out]
        }
        n756 = property on="usb2000p_ConnectButton" class="Bool (strict)"("BoolText.Text"="Connect" ("Boolean Text.Text"), "BoolText.TextColor"=w1651, "DisabledEnum"=T22."Enabled" ("Disabled")) -> ()  [unwired: 2 in, 2 out]
        n757 = local read "textColorGreen"() -> (w1640:u32)
        n758 = call "updateRealTimeInfo.vi"("UI_Data"=w1682) -> ()  [unwired: 11 in]
        n759 = local read "textColorGreen"() -> (w1706:u32)
        n760 = control-ref of="cB_getObjectInfo"() -> (w1748:refnum<vi>)
        n761 = control-ref of="cB_rotate"() -> (w1751:refnum<vi>)
        n762 = property on="pBot_runScan" class="Bool (strict)"("BoolText.Text"="Start scan" ("Boolean Text.Text"), "BoolText.TextColor"=w1640) -> ()  [unwired: 2 in, 2 out]
        n763 = call-poly <userlib>:"MGI Disable Enum (Small).vi"() -> ("Disabled & Grayed"=w1711:T22)
        n764 = call-poly <userlib>:"MGI Disable Enum (Small).vi"() -> ("Disabled & Grayed"=w1712:T22)
        n765 = Index Array(array=w1710) -> (element=w1709:string)  [unwired: 1 in]
        n766 = Index Array(array=w1737) -> (element=w1736:string)  [unwired: 1 in]
        n767 = Index Array(array=w1654) -> (element=w1655:string)  [unwired: 1 in]
        n768 = property class="Bool (strict)"(reference=w1748, "DisabledEnum"=w1711, "Value"=FALSE) -> ()  [unwired: 1 in, 2 out]
        n769 = property class="Bool (strict)"(reference=w1751, "DisabledEnum"=w1712, "Value"=FALSE) -> ()  [unwired: 1 in, 2 out]
        n770 = property on="pBot_ConnectButton" class="Bool (strict)"("BoolText.Text"="Connect" ("Boolean Text.Text"), "BoolText.TextColor"=w1706, "DisabledEnum"=T22."Enabled" ("Disabled")) -> ()  [unwired: 2 in, 2 out]
        n771 = property on="pBot_scanInstrument" class="CmbBox"("Strings[]"=w1710, "Value"=w1709) -> ()  [unwired: 2 in, 2 out]
        n772 = property on="pBot_VISAstrings" class="CmbBox"("Strings[]"=w1737, "Value"=w1736) -> ()  [unwired: 2 in, 2 out]
        n773 = property on="usb2000p_VISAstrings" class="CmbBox"("Strings[]"=w1654, "Value"=w1655) -> ()  [unwired: 2 in, 2 out]
      }
      frame "changeControlTab" {
        # "this changes the visible tab of the controlTab and updates the toggle buttons acting as the Tabs"
        n774 = local read "cB_plasmaBot"() -> (w1864:bool)
        n775 = local read "cB_USB2000+"() -> (w1867:bool)
        n776 = local read "cB_dataView"() -> (w1865:bool)
        n777 = local read "cB_3Dview"() -> (w1866:bool)
        n778 = Unbundle By Name(w1860) -> ("controlTabState"=w1863:bool[])
        n779 = Build Array(w1864, w1867, w1866, w1865) -> (w1859:bool[])
        n780 = Exclusive Or(1:w1863, 2:w1859) -> (0:w1849:bool[])
        n781 = Bundle By Name(cluster=w1860, "controlTabState"=w1849) -> (w1858:T9)
        n782 = Index Array(array=w1849, index=0) -> (element=w1854:bool)
        n783 = Index Array(array=w1849, index=1) -> (element=w1855:bool)
        n784 = Index Array(array=w1849, index=2) -> (element=w1856:bool)
        n785 = Index Array(array=w1849, index=3) -> (element=w1857:bool)
        n786 = Search 1D Array(1D array=w1849, element=TRUE) -> (index of element=w1861:i32)  [unwired: 1 in]
        n787 = local write "cB_plasmaBot"(w1854) -> ()
        n788 = local write "cB_USB2000+"(w1855) -> ()
        n789 = local write "cB_3Dview"(w1856) -> ()
        n790 = local write "cB_dataView"(w1857) -> ()
        n791 = local write "controlTab"(w1861) -> ()
        n792 = Merge Errors(w1869) -> (w1868:errorcluster)
      }
      frame "toggleView" {
        # "This changes the tab of the viewPane from the 3D Picture to the data"
        n793 = property on="3D Picture" class="SceneGraphDisp (strict)"() -> ("Visible"=w1873:bool)  [unwired: 2 in, 2 out]
        n794 = property on="1DdataGraph" class="XYGraph (strict)"() -> ("Visible"=w1871:bool)  [unwired: 2 in, 2 out]
        n795 = Not(x=w1871) -> (.not. x?=w1870:bool)
        n796 = Not(x=w1873) -> (.not. x?=w1872:bool)
        n797 = local write "cB_toggleView"(FALSE ("cB_toggleView")) -> ()
        n798 = property on="1DdataGraph" class="XYGraph (strict)"("Visible"=w1870) -> ()  [unwired: 2 in, 2 out]
        n799 = property on="3D Picture" class="SceneGraphDisp (strict)"("Visible"=w1872) -> ()  [unwired: 2 in, 2 out]
      }
      frame "updateDisplay" {
        # "Update Display - Convert the message data to a string to display in the Data Display indicator."
        n800 = Unbundle By Name(w1902) -> ("ZtranslateObjControls"=w1900:refnum<vi>[], "XYtranslateObjControls"=w1899:refnum<vi>[], "selectedObj.allowedMotion"=w1901:enum16{"XY", "Z"}, "selectedObj.Name"=w1897:string)
        n801 = case shown="Default" w1897 {
          tunnel: w1901 -> [w1907 _]
          tunnel: w1900 -> [w1906 w1939]
          tunnel: w1899 -> [w1905 w1938]
          frame Default {
            # "An object is selected; so, enable the appropriate buttons"
            n802 = case shown="Default" w1907 {
              tunnel: w1906 -> [w1912 w1923 w1933]
              tunnel: w1905 -> [w1913 w1922 w1932]
              frame "XY" {
                n803 = for {
                  tunnel: w1912 -> [w1916] mode=indexing
                  n804 = property class="Bool (strict)"(reference=w1916, "DisabledEnum"=T22."Disabled and Grayed Out" ("Disabled")) -> ()  [unwired: 1 in, 2 out]
                }
                n805 = for {
                  tunnel: w1913 -> [w1915] mode=indexing
                  n806 = property class="Bool (strict)"(reference=w1915, "DisabledEnum"=T22."Enabled" ("Disabled")) -> ()  [unwired: 1 in, 2 out]
                }
                n807 = control-ref of="cB_rotate"() -> (w1911:refnum<vi>)
                n808 = control-ref of="cB_getObjectInfo"() -> (w1909:refnum<vi>)
                n809 = property class="Bool (strict)"(reference=w1911, "DisabledEnum"=T22."Enabled" ("Disabled")) -> ()  [unwired: 1 in, 2 out]
                n810 = property class="Bool (strict)"(reference=w1909, "DisabledEnum"=T22."Enabled" ("Disabled")) -> ()  [unwired: 1 in, 2 out]
              }
              frame "Z" {
                n811 = for {
                  tunnel: w1923 -> [w1926] mode=indexing
                  n812 = property class="Bool (strict)"(reference=w1926, "DisabledEnum"=T22."Enabled" ("Disabled")) -> ()  [unwired: 1 in, 2 out]
                }
                n813 = for {
                  tunnel: w1922 -> [w1925] mode=indexing
                  n814 = property class="Bool (strict)"(reference=w1925, "DisabledEnum"=T22."Disabled and Grayed Out" ("Disabled")) -> ()  [unwired: 1 in, 2 out]
                }
                n815 = control-ref of="cB_rotate"() -> (w1921:refnum<vi>)
                n816 = control-ref of="cB_getObjectInfo"() -> (w1919:refnum<vi>)
                n817 = property class="Bool (strict)"(reference=w1921, "DisabledEnum"=T22."Enabled" ("Disabled")) -> ()  [unwired: 1 in, 2 out]
                n818 = property class="Bool (strict)"(reference=w1919, "DisabledEnum"=T22."Enabled" ("Disabled")) -> ()  [unwired: 1 in, 2 out]
              }
              frame Default {
                n819 = for {
                  tunnel: w1933 -> [w1936] mode=indexing
                  n820 = property class="Bool (strict)"(reference=w1936, "DisabledEnum"=T22."Disabled and Grayed Out" ("Disabled")) -> ()  [unwired: 1 in, 2 out]
                }
                n821 = for {
                  tunnel: w1932 -> [w1935] mode=indexing
                  n822 = property class="Bool (strict)"(reference=w1935, "DisabledEnum"=T22."Disabled and Grayed Out" ("Disabled")) -> ()  [unwired: 1 in, 2 out]
                }
                n823 = control-ref of="cB_rotate"() -> (w1931:refnum<vi>)
                n824 = control-ref of="cB_getObjectInfo"() -> (w1929:refnum<vi>)
                n825 = property class="Bool (strict)"(reference=w1931, "DisabledEnum"=T22."Disabled and Grayed Out" ("Disabled")) -> ()  [unwired: 1 in, 2 out]
                n826 = property class="Bool (strict)"(reference=w1929, "DisabledEnum"=T22."Disabled and Grayed Out" ("Disabled")) -> ()  [unwired: 1 in, 2 out]
              }
            }
          }
          frame "" {
            # "An object is not selected; so, disable the object translate/rotate/info buttons"
            n827 = for {
              tunnel: w1939 -> [w1946] mode=indexing
              n828 = property class="Bool (strict)"(reference=w1946, "DisabledEnum"=T22."Disabled and Grayed Out" ("Disabled")) -> ()  [unwired: 1 in, 2 out]
            }
            n829 = for {
              tunnel: w1938 -> [w1945] mode=indexing
              n830 = property class="Bool (strict)"(reference=w1945, "DisabledEnum"=T22."Disabled and Grayed Out" ("Disabled")) -> ()  [unwired: 1 in, 2 out]
            }
            n831 = control-ref of="cB_rotate"() -> (w1943:refnum<vi>)
            n832 = control-ref of="cB_getObjectInfo"() -> (w1941:refnum<vi>)
            n833 = property class="Bool (strict)"(reference=w1943, "DisabledEnum"=T22."Disabled and Grayed Out" ("Disabled")) -> ()  [unwired: 1 in, 2 out]
            n834 = property class="Bool (strict)"(reference=w1941, "DisabledEnum"=T22."Disabled and Grayed Out" ("Disabled")) -> ()  [unwired: 1 in, 2 out]
          }
        }
        n835 = property on="viewPane" class="Pane"() -> ("ContentBnds"=w1889:T27)  [unwired: 2 in, 2 out]
        n836 = Unbundle By Name(w1889) -> ("Left"=w1886:i16, "Top"=w1879:i16, "Right"=w1887:i16, "Bottom"=w1888:i16)
        n837 = Merge Errors(w1898) -> (w1904:errorcluster)
        n838 = Subtract(x=w1888, y=w1879) -> (x-y=w1885:i16)
        n839 = Subtract(x=w1887, y=w1886) -> (x-y=w1884:i16)
        n840 = Subtract(x=w1885, y=i16 75) -> (x-y=w1880:i16)
        n841 = property on="3D Picture" class="SceneGraphDisp (strict)" props=["Left", "Top", "ContentBounds:Height", "Content Bounds.Width", "Visible"]("Left"=w1886, "Top"=w1879, "ContentBounds:Height"=w1885, "Content Bounds.Width"=w1884) -> ()  [unwired: 2 in, 3 out]
        n842 = Subtract(x=w1884, y=i16 100) -> (x-y=w1881:i16)
        n843 = Add(x=i16 10, y=w1879) -> (x+y=w1877:i16)
        n844 = property on="1DdataGraph" class="XYGraph (strict)"("Left"=w1886, "Top"=w1877, "Height"=w1880, "Width"=w1881) -> ()  [unwired: 2 in, 2 out]
        n845 = property on="viewInfoPane" class="Pane"() -> ("ContentBnds"=w1903:T27)  [unwired: 2 in, 2 out]
        n846 = property on="pBot_ExperimentTabControl" class="TabCtl (strict)"() -> ("Top"=w1894:i32)  [unwired: 2 in, 2 out]
        n847 = property on="controlPane" class="Pane"() -> ("ContentBnds"=w1896:T27)  [unwired: 2 in, 2 out]
        n848 = Unbundle By Name(w1896) -> ("Bottom"=w1895:i16)
        n849 = Unbundle By Name(w1903) -> ("Right"=w1890:i16)  [unwired: 1 out]
        n850 = Subtract(x=w1895, y=w1894) -> (x-y=w1893:i32)
        n851 = property on="cB_toggleView" class="Bool (strict)"() -> ("Width"=w1892:u32)  [unwired: 2 in, 2 out]
        n852 = property on="pBot_ExperimentTabControl" class="TabCtl (strict)"("PaneHeight"=w1893) -> ()  [unwired: 2 in, 2 out]
        n853 = Subtract(x=w1890, y=w1892) -> (x-y=w1891:u32)
        n854 = property on="cB_toggleView" class="Bool (strict)"("Left"=w1891) -> ()  [unwired: 2 in, 2 out]
      }
      frame "pBot_getInstruments" {
        w1955 = T28 2 items=["Canonical Names Only"=0, "Aliases Only"=2, "Include Matching Aliases"=3, "Include All Aliases"=4] ("Search Mode")
        # "Don't show anything other than COM ports. For debugging, you might want to switch the enabled and the disabled to also show other serial ports, such as the printrport LPT1"
        n855 = VISA Find Resource(10:w1955, 11:"ASRL[0-9]*::?*INSTR" ("expression (\"?*\")")) -> (3:w1954:string[])  [unwired: 1 in, 2 out]
        n856 = for {
          tunnel: w1954 -> [w1971] mode=indexing
          shift-right: [w1973] -> w1950
          shift-left: string[] [] -> [w1974]
          n857 = String Subset(string=w1971, length (rest)=3 ("length (rest)")) -> (substring=w1972:string)  [unwired: 1 in]
          n858 = Equal?(x=w1972, y="COM" ("expression (\"?*\")")) -> (x = y?=w1975:bool)
          n859 = case shown="False" w1975 {
            tunnel: w1974 -> [w1980 w1983]
            tunnel: [w1978 w1981] -> w1973
            tunnel: w1971 -> [w1979 w1982]
            frame True {
              n860 = Build Array (concatenate)(w1980, w1979) -> (w1978:string[])
            }
            frame False {
              n861 = disable-structure shown="Disabled" {
                disable-tunnel: w1983 -> [w1986 w1987]
                disable-tunnel: w1982 -> [w1985 _]
                disable-tunnel: [w1984 w1987] -> w1981
                frame Disabled {
                  n862 = Build Array (concatenate)(w1986, w1985) -> (w1984:string[])
                }
                frame Enabled {
                }
              }
            }
          }
        }
        n863 = Array Size(array=w1950) -> (size(s)=w1952:i32)
        n864 = Not Equal To 0?(x=w1952) -> (x != 0?=w1951:bool)
        n865 = case shown="True" w1951 {
          tunnel: w1950 -> [_ w1970]
          tunnel: w1949 -> [w1959 w1967]
          tunnel: [w1958 w1967] -> w1948
          frame False {
            n866 = local read "numberOfCommandLines"() -> (w1964:i32)
            n867 = call "setCommandString.vi"("addLF? (T)"=TRUE ("addLF?"), "addTimeAndChevron? (T)"=TRUE ("addTimeAndChevron?"), "numLines"=w1964, "stringToAdd"="No COM ports found!", "UI Data In"=w1959) -> ("error out"=w1960:errorcluster, "UI Data Out"=w1958:T9, "outputCommandString"=w1962:string)  [unwired: 4 in]
            n868 = local write "cB_commandLog"(w1962) -> ()
            n869 = property on="cB_commandLog" class="Str"(error in=w1960, "Text.Scroll Position"=inf) -> ()  [unwired: 1 in, 2 out]
          }
          frame True {
            n870 = Index Array(array=w1970, index=0) -> (element=w1968:string)
            n871 = property on="pBot_VISAstrings" class="CmbBox"("Strings[]"=w1970, "Value"=w1968) -> ()  [unwired: 2 in, 2 out]
          }
        }
      }
      frame "usb2000p_getInstruments" {
        w1995 = T28 2 items=["Canonical Names Only"=0, "Aliases Only"=2, "Include Matching Aliases"=3, "Include All Aliases"=4] ("Search Mode")
        # "Don't show anything other than COM ports. For debugging, you might want to switch the enabled and the disabled to also show other serial ports, such as the printrport LPT1"
        n872 = VISA Find Resource(10:w1995) -> (3:w1994:string[])  [unwired: 2 in, 2 out]
        n873 = for {
          tunnel: w1994 -> [w2009] mode=indexing
          shift-right: [w2011] -> w1990
          shift-left: string[] [] -> [w2012]
          n874 = String Subset(string=w2009, length (rest)=3 ("length (rest)")) -> (substring=w2010:string)  [unwired: 1 in]
          n875 = Equal?(x=w2010, y="USB" ("expression (\"?*\")")) -> (x = y?=w2013:bool)
          n876 = case shown="False" w2013 {
            tunnel: w2012 -> [w2018 w2021]
            tunnel: [w2016 w2019] -> w2011
            tunnel: w2009 -> [w2017 w2020]
            frame True {
              n877 = Build Array (concatenate)(w2018, w2017) -> (w2016:string[])
            }
            frame False {
              n878 = disable-structure shown="Disabled" {
                disable-tunnel: w2021 -> [w2024 w2025]
                disable-tunnel: w2020 -> [w2023 _]
                disable-tunnel: [w2022 w2025] -> w2019
                frame Disabled {
                  n879 = Build Array (concatenate)(w2024, w2023) -> (w2022:string[])
                }
                frame Enabled {
                }
              }
            }
          }
        }
        n880 = Array Size(array=w1990) -> (size(s)=w1992:i32)
        n881 = Not Equal To 0?(x=w1992) -> (x != 0?=w1991:bool)
        n882 = case shown="True" w1991 {
          tunnel: w1990 -> [_ w2008]
          tunnel: w1989 -> [w1999 w2005]
          tunnel: [w1998 w2005] -> w1988
          frame False {
            n883 = local read "numberOfCommandLines"() -> (w2002:i32)
            n884 = call "setCommandString.vi"("addLF? (T)"=TRUE ("addLF?"), "addTimeAndChevron? (T)"=TRUE ("addTimeAndChevron?"), "numLines"=w2002, "stringToAdd"="No USB devices found!", "UI Data In"=w1999) -> ("UI Data Out"=w1998:T9, "outputCommandString"=w1997:string)  [unwired: 4 in, 1 out]
            n885 = property on="cB_commandLog" class="Str"("Text.Scroll Position"=inf, "Text.Text"=w1997) -> ()  [unwired: 2 in, 2 out]
          }
          frame True {
            n886 = Index Array(array=w2008, index=0) -> (element=w2006:string)
            n887 = property on="usb2000p_VISAstrings" class="CmbBox"("Strings[]"=w2008, "Value"=w2006) -> ()  [unwired: 2 in, 2 out]
          }
        }
      }
      frame "usb2000p_tryToConnect" {
        # "This is a general instrument. It needs a name, a VISA address and a 1D array size for the data it collects. If this instrument is already connected, then it will be present in the UI_Data.connectedInstruments array."
        n888 = Unbundle By Name(w2027) -> ("connectedInstruments"=w2033:T7[])
        n889 = local write "usb2000p_ConnectButton"(FALSE ("usb2000p_ConnectButton")) -> ()
        n890 = for {
          tunnel: w2033 -> [w2058] mode=indexing
          tunnel: "USB2000p" ("instrumentName") -> [w2060]
          tunnel: [w2059] -> w2031
          tunnel: [w2058] -> w2029
          stop <- w2059 stop-if-true
          n891 = Unbundle By Name(w2058) -> ("Name"=w2061:string)
          n892 = Equal?(x=w2061, y=w2060) -> (x = y?=w2059:bool)
        }
        n893 = case shown="False" w2031 {
          tunnel: w2030 -> [w2038 w2057]
          tunnel: w2029 -> [_ w2055]
          tunnel: w2027 -> [w2036 w2054]
          tunnel: [w2035 w2054] -> w2026
          frame False {
            # "Object is not connected, try to connect"
            n894 = property on="usb2000p_VISAstrings" class="CmbBox"() -> ("Value"=w2037:string)  [unwired: 2 in, 2 out]
            n895 = case shown="Default" w2037 {
              selector: w2037 -> [w2040 _]
              tunnel: w2038 -> [w2043 _]
              tunnel: w2036 -> [w2039 w2048]
              tunnel: [w2039 w2047] -> w2035
              frame Default {
                n896 = Bundle(cluster=T7 {"Name"="", "VISAname"="", "1D_dataArraySize"=0, "extraInfo"=variant, "error"={"status"=FALSE, "code"=0, "source"=""}} ("instrumentInfo"), "Name"="USB2000p", "VISAname"=w2040) -> (w2042:T7)  [unwired: 3 in]
                n897 = call-poly "Enqueue Message.vi"("Message Data"=w2042, "Message"="usb2000p_Connect", "Message Queue"=w2043) -> ()  [unwired: 7 in, 2 out]
              }
              frame "" {
                n898 = local read "numberOfCommandLines"() -> (w2051:i32)
                n899 = call "setCommandString.vi"("addLF? (T)"=TRUE ("addLF?"), "addTimeAndChevron? (T)"=TRUE ("addTimeAndChevron?"), "numLines"=w2051, "stringToAdd"="Error! You must first select the USB2000+ port.", "UI Data In"=w2048) -> ("UI Data Out"=w2047:T9, "outputCommandString"=w2046:string)  [unwired: 4 in, 1 out]
                n900 = property on="cB_commandLog" class="Str"("Text.Scroll Position"=inf, "Text.Text"=w2046) -> ()  [unwired: 2 in, 2 out]
              }
            }
          }
          frame True {
            # "Object is connected, try to disconnect"
            n901 = call-poly "Enqueue Message.vi"("Message Data"=w2055, "Message"="usb2000p_Disconnect", "Message Queue"=w2057) -> ()  [unwired: 7 in, 2 out]
          }
        }
      }
      frame "usb2000p_connected?" {
        n902 = Variant To Data(error in=w2077, type=T7 {"Name"="", "VISAname"="", "1D_dataArraySize"=0, "extraInfo"=variant, "error"={"status"=FALSE, "code"=0, "source"=""}} ("instrumentInfo"), Variant=w2076) -> (data=w2073:T7)  [unwired: 1 out]
        n903 = Unbundle By Name(w2073) -> ("error"=w2074:errorcluster)
        n904 = case shown="No Error" w2074 {
          selector: w2074 -> [_ w2110]
          tunnel: w2073 -> [w2086 _]
          tunnel: w2072 -> [w2084 w2101]
          tunnel: [w2093 w2103] -> w2066
          tunnel: ["Connected to USB2000+" ("source") w2102] -> w2065
          tunnel: w2062 -> [w2082 _]
          frame No Error {
            n905 = Unbundle By Name(w2086) -> ("Name"=w2088:string, "extraInfo"=w2087:variant)
            n906 = Unbundle By Name(w2084) -> ("usb2000p_controlRefs"=w2083:refnum<vi>[])
            n907 = local read "textColorRed"() -> (w2091:u32)
            n908 = property on="pBot_scanInstrument" class="CmbBox"() -> ("Strings[]"=w2090:string[])  [unwired: 2 in, 2 out]
            n909 = Variant To Data(type=dbl[] [] ("Wavelengths"), Variant=w2087) -> (data=w2078:dbl[])  [unwired: 1 in, 1 out]
            n910 = in-place {
              in-place-border: w2086 -> [w2097]
              in-place-border: w2078 -> [w2096]
              n911 = in-place-cluster #9(w2084) -> ("connectedInstruments"=w2099:T7[])  [unwired: 1 out]
              n912 = Build Array (concatenate)(w2099, w2097) -> (w2098:T7[])
              n913 = in-place-cluster #9("Wavelengths"=w2096, "connectedInstruments"=w2098) -> (w2093:T9)
            }
            n914 = property on="usb2000p_ConnectButton" class="Bool (strict)"("BoolText.Text"="Disconnect" ("Boolean Text.Text"), "BoolText.TextColor"=w2091) -> ()  [unwired: 2 in, 2 out]
            n915 = Build Array (concatenate)(w2090, w2088) -> (w2089:string[])
            n916 = property on="pBot_scanInstrument" class="CmbBox"("Strings[]"=w2089) -> ()  [unwired: 2 in, 2 out]
            n917 = local read "usb2000p_intTime"() -> (w2080:u32)
            n918 = for {
              tunnel: w2083 -> [w2095] mode=indexing
              n919 = property class="Ctl"(reference=w2095, "DisabledEnum"=T22."Enabled" ("Disabled")) -> ()  [unwired: 1 in, 2 out]
            }
            n920 = call-poly "Enqueue Message.vi"("Message Data"=w2080, "Message"="usb2000p_setIntegrationTime", "Message Queue"=w2082) -> ()  [unwired: 7 in, 2 out]
          }
          frame Error {
            # "If there is an error, either there was a real error, or it was sucessfully disconnected"
            n921 = in-place {
              n922 = in-place-cluster #10(w2101) -> ("connectedInstruments"=w2118:T7[])
              n923 = for {
                tunnel: w2118 -> [w2122] mode=indexing
                tunnel: "USB2000p" ("instrumentName") -> [w2124]
                tunnel: [w2123] -> _
                tunnel: [w2121] -> w2119
                i -> [w2121]
                stop <- w2123 stop-if-true
                n924 = Unbundle By Name(w2122) -> ("Name"=w2125:string)
                n925 = Equal?(x=w2125, y=w2124) -> (x = y?=w2123:bool)
              }
              n926 = Delete From Array(array=w2118, index=w2119) -> (array with subset deleted=w2117:T7[])  [unwired: 1 in, 1 out]
              n927 = in-place-cluster #10("connectedInstruments"=w2117) -> (w2103:T9)
            }
            n928 = Unbundle By Name(w2101) -> ("usb2000p_controlRefs"=w2100:refnum<vi>[])
            n929 = Unbundle By Name(w2110) -> ("source"=w2102:string)
            n930 = property on="pBot_scanInstrument" class="CmbBox"() -> ("Strings[]"=w2105:string[])  [unwired: 2 in, 2 out]
            n931 = local read "textColorGreen"() -> (w2108:u32)
            n932 = for {
              tunnel: w2105 -> [w2113] mode=indexing
              tunnel: "USB2000p" ("instrumentName") -> [w2116]
              tunnel: [w2115] -> _
              tunnel: [w2114] -> w2106
              i -> [w2114]
              stop <- w2115 stop-if-true
              n933 = Equal?(x=w2113, y=w2116) -> (x = y?=w2115:bool)
            }
            n934 = for {
              tunnel: w2100 -> [w2111] mode=indexing
              n935 = call-poly <userlib>:"MGI Disable Enum (Small).vi"() -> ("Disabled & Grayed"=w2112:T22)
              n936 = property class="Ctl"(reference=w2111, "DisabledEnum"=w2112) -> ()  [unwired: 1 in, 2 out]
            }
            n937 = property on="usb2000p_ConnectButton" class="Bool (strict)"("BoolText.Text"="Connect" ("Boolean Text.Text"), "BoolText.TextColor"=w2108) -> ()  [unwired: 2 in, 2 out]
            n938 = Delete From Array(array=w2105, index=w2106) -> (array with subset deleted=w2104:string[])  [unwired: 1 in, 1 out]
            n939 = property on="pBot_scanInstrument" class="CmbBox"("Strings[]"=w2104) -> ()  [unwired: 2 in, 2 out]
          }
        }
        n940 = local read "numberOfCommandLines"() -> (w2063:i32)
        n941 = call "setCommandString.vi"("addLF? (T)"=TRUE ("addLF?"), "addTimeAndChevron? (T)"=TRUE ("addTimeAndChevron?"), "numLines"=w2063, "stringToAdd"=w2065, "UI Data In"=w2066) -> ("UI Data Out"=w2064:T9, "outputCommandString"=w2067:string)  [unwired: 4 in, 1 out]
        n942 = property on="cB_commandLog" class="Str"("Text.Scroll Position"=inf, "Text.Text"=w2067) -> ()  [unwired: 2 in, 2 out]
      }
      frame "usb2000p_setIntegrationTime" {
        n943 = local read "usb2000p_intTime"() -> (w2126:u32)
        n944 = call-poly "Enqueue Message.vi"("Message Data"=w2126, "Message"="usb2000p_setIntegrationTime" ("expression (\"?*\")"), "Message Queue"=w2128) -> ()  [unwired: 7 in, 2 out]
      }
      frame "usb2000p_acquireSpec" {
        n945 = call-poly "Enqueue Message.vi"("Message"="usb2000p_acquireSpec", "Message Queue"=w2133) -> ()  [unwired: 8 in, 2 out]
        n946 = local write "usb2000p_aquireSpectra"(FALSE ("usb2000p_saveSpectra")) -> ()
      }
      frame "connectToPBot" {
        n947 = Variant To Data(error in=w2148, type=T11 {"Message"="equip", "error constant"={"status"=FALSE, "code"=0, "source"=""}, "disconnectPBot_Event"=refnum}, Variant=w2147) -> (data=w2146:T11, error out=w2140:errorcluster)
        n948 = Unbundle(w2146) -> ("Message"=w2145:string, "error constant"=w2144:errorcluster, "disconnectPBot_Event"=w2137:refnum<user-event>)
        n949 = case shown="\"equip\"" w2145 {
          selector: w2145 -> [w2152 _ _]
          tunnel: w2143 -> [w2153 w2165 w2202]
          tunnel: w2149 -> [_ w2166 w2199]
          tunnel: w2144 -> [_ _ w2212]
          tunnel: [w2153 w2164 w2204] -> w2142
          tunnel: [w2151 _ _] -> w2139
          tunnel: w2137 -> [_ _ w2200]
          tunnel: w2136 -> [_ w2161 _]
          frame Default {
            n950 = xnode "Error Ring"("parameter 0"=w2152) -> ("error out"=w2151:errorcluster)
          }
          frame "event" {
            # "determine if we are already connected or not"
            # "The event was called by the Event Handeling Loop"
            n951 = Unbundle By Name(w2165) -> ("disconnectPBot_Event"=w2163:refnum<user-event>, "pBotConnected?"=w2167:bool, "isScanning?"=w2162:bool)
            n952 = case shown="False" w2167 {
              tunnel: w2166 -> [w2170 w2190]
              tunnel: w2165 -> [w2169 w2194]
              tunnel: [w2168 w2194] -> w2164
              tunnel: w2163 -> [_ w2193]
              tunnel: w2162 -> [_ w2186]
              tunnel: w2161 -> [_ w2185]
              frame False {
                # "The user hit Connect (we are not connected), so lets tell the Equipment Control Loop to try and connect"
                n953 = property on="pBot_VISAstrings" class="CmbBox"() -> ("Value"=w2171:string)  [unwired: 2 in, 2 out]
                n954 = case shown="Default" w2171 {
                  selector: w2171 -> [w2173 _]
                  tunnel: w2170 -> [w2175 _]
                  tunnel: w2169 -> [w2172 w2177]
                  tunnel: [w2172 w2176] -> w2168
                  frame Default {
                    n955 = call-poly "Enqueue Message.vi"("Message Data"=w2173, "Message"="connectToPBot", "Message Queue"=w2175) -> ()  [unwired: 7 in, 2 out]
                  }
                  frame "" {
                    n956 = local read "numberOfCommandLines"() -> (w2181:i32)
                    n957 = call "setCommandString.vi"("addLF? (T)"=TRUE ("addLF?"), "addTimeAndChevron? (T)"=TRUE ("addTimeAndChevron?"), "numLines"=w2181, "stringToAdd"="Error! You must first select the plasmaBot's port.", "UI Data In"=w2177) -> ("error out"=w2184:errorcluster, "UI Data Out"=w2176:T9, "outputCommandString"=w2178:string)  [unwired: 4 in]
                    n958 = local write "cB_commandLog"(w2178) -> ()
                    n959 = property on="cB_commandLog" class="Str"(error in=w2184, "Text.Scroll Position"=inf) -> ()  [unwired: 1 in, 2 out]
                  }
                }
              }
              frame True {
                # "We are connected, (the user clicked Disconnect) so we will tell the ECL to try and disconnect"
                n960 = Generate User Event(priority (normal)=usereventprio."high priority", user event=w2193, event data cluster=TRUE ("event data")) -> (error out=w2188:errorcluster)  [unwired: 1 in, 1 out]
                n961 = Flush Queue(queue=w2190, error in (no error)=w2188) -> (queue out=w2189:refnum<queue>, error out=w2187:errorcluster)  [unwired: 1 out]
                n962 = call-poly "Enqueue Message.vi"("error in (no error)"=w2187, "Message"="disconnectFromPBot", "Message Queue"=w2189) -> ()  [unwired: 7 in, 2 out]
                n963 = case shown="True" w2186 {
                  tunnel: w2185 -> [_ w2196]
                  frame False {
                  }
                  frame True {
                    n964 = call-poly "Enqueue Message.vi"("Message Data"=errorcluster {"status"=TRUE, "code"=0, "source"="Scan terminated successfully!"} ("error constant"), "Message"="scanComplete", "Message Queue"=w2196) -> ()  [unwired: 7 in, 2 out]
                  }
                }
              }
            }
          }
          frame "equip" {
            # "The event was called by the Equipment Control Loop  -  depending on the error cluster in we determin if we sucessfully connected to the plasmaBot or not"
            n965 = Unbundle By Name(w2202) -> ("pBotConnected?"=w2201:bool)
            n966 = case shown="False" w2201 {
              tunnel: w2212 -> [w2218 w2238]
              tunnel: [w2217 w2236] -> w2205
              tunnel: [w2216 w2235] -> w2203
              tunnel: w2202 -> [w2215 w2237]
              tunnel: w2200 -> [w2214 _]
              tunnel: w2199 -> [w2213 _]
              frame False {
                # "The ECL returned from us asking it to connect to the plasmaBot. If there is no error than we sucessfully connected. If there is an error, then we did not sucessfully connect."
                n967 = case shown="No Error" w2218 {
                  selector: w2218 -> [_ w2234]
                  tunnel: ["Connected to plasmaBot" ("Boolean Text.Text") w2233] -> w2217
                  tunnel: w2215 -> [w2222 w2232]
                  tunnel: [w2223 w2232] -> w2216
                  tunnel: w2214 -> [w2224 _]
                  tunnel: w2213 -> [w2220 _]
                  frame No Error {
                    # "Do stuff with the EEPROM settings returned here after the EEPROM has been set to the correct values. For example load in M212 and use it as the yPOI_Home to change homePos_offset to the correct value."
                    n968 = Unbundle By Name(w2222) -> ("pBot_controls"=w2226:refnum<vi>[])
                    n969 = local read "textColorRed"() -> (w2227:u32)
                    n970 = for {
                      tunnel: w2226 -> [w2230] mode=indexing
                      n971 = property class="Ctl"(reference=w2230, "DisabledEnum"=T22."Enabled" ("Disabled")) -> ()  [unwired: 1 in, 2 out]
                    }
                    n972 = property on="pBot_ConnectButton" class="Bool (strict)"("BoolText.Text"="Disconnect" ("Boolean Text.Text"), "BoolText.TextColor"=w2227) -> ()  [unwired: 2 in, 2 out]
                    n973 = call-poly <userlib>:"MGI Disable Enum (Small).vi"() -> ("Enabled"=w2219:T22)
                    n974 = property on="pBot_runScan" class="Bool (strict)"("DisabledEnum"=w2219) -> ()  [unwired: 2 in, 2 out]
                    n975 = Bundle By Name(cluster=w2222, "pBotConnected?"=TRUE, "disconnectPBot_Event"=w2224) -> (w2223:T9)
                    n976 = call-poly "Enqueue Message.vi"("Message"="getCurrentInfo", "Message Queue"=w2220) -> ()  [unwired: 8 in, 2 out]
                  }
                  frame Error {
                    n977 = Unbundle(w2234) -> ("source"=w2233:string)  [unwired: 2 out]
                  }
                }
              }
              frame True {
                # "The ECL returned from us asking it to disconnect from the plasmaBot. If there is no error, then we sucessfully disconnected. If there is an error, then we did not sucessfully disconnect."
                n978 = case shown="No Error" w2238 {
                  selector: w2238 -> [w2244 w2251]
                  tunnel: w2237 -> [w2242 w2252]
                  tunnel: [w2243 w2250] -> w2236
                  tunnel: [w2240 w2257] -> w2235
                  frame No Error {
                    n979 = Unbundle By Name(w2242) -> ("pBot_controls"=w2245:refnum<vi>[])
                    n980 = Unbundle(w2244) -> ("source"=w2243:string)  [unwired: 2 out]
                    n981 = for {
                      tunnel: w2245 -> [w2249] mode=indexing
                      n982 = call-poly <userlib>:"MGI Disable Enum (Small).vi"() -> ("Disabled & Grayed"=w2248:T22)
                      n983 = property class="Ctl"(reference=w2249, "DisabledEnum"=w2248) -> ()  [unwired: 1 in, 2 out]
                    }
                    n984 = local read "textColorGreen"() -> (w2246:u32)
                    n985 = call-poly <userlib>:"MGI Disable Enum (Small).vi"() -> ("Disabled & Grayed"=w2239:T22)
                    n986 = property on="pBot_runScan" class="Bool (strict)"("DisabledEnum"=w2239) -> ()  [unwired: 2 in, 2 out]
                    n987 = property on="pBot_ConnectButton" class="Bool (strict)"("BoolText.Text"="Connect" ("Boolean Text.Text"), "BoolText.TextColor"=w2246) -> ()  [unwired: 2 in, 2 out]
                    n988 = Bundle By Name(cluster=w2242, "pBotConnected?"=FALSE) -> (w2240:T9)
                  }
                  frame Error {
                    n989 = Unbundle(w2251) -> ("source"=w2250:string)  [unwired: 2 out]
                    n990 = Unbundle By Name(w2252) -> ("pBot_controls"=w2254:refnum<vi>[])
                    n991 = for {
                      tunnel: w2254 -> [w2260] mode=indexing
                      n992 = call-poly <userlib>:"MGI Disable Enum (Small).vi"() -> ("Disabled & Grayed"=w2259:T22)
                      n993 = property class="Ctl"(reference=w2260, "DisabledEnum"=w2259) -> ()  [unwired: 1 in, 2 out]
                    }
                    n994 = local read "textColorRed"() -> (w2255:u32)
                    n995 = call-poly <userlib>:"MGI Disable Enum (Small).vi"() -> ("Disabled & Grayed"=w2253:T22)
                    n996 = property on="pBot_ConnectButton" class="Bool (strict)"("BoolText.Text"="Error" ("Boolean Text.Text"), "BoolText.TextColor"=w2255, "DisabledEnum"=w2253) -> ()  [unwired: 2 in, 2 out]
                    n997 = Bundle By Name(cluster=w2252, "pBotConnected?"=FALSE) -> (w2257:T9)
                  }
                }
              }
            }
            n998 = local read "numberOfCommandLines"() -> (w2208:i32)
            n999 = call "setCommandString.vi"("addLF? (T)"=TRUE ("addLF?"), "addTimeAndChevron? (T)"=TRUE ("addTimeAndChevron?"), "numLines"=w2208, "stringToAdd"=w2205, "UI Data In"=w2203) -> ("error out"=w2211:errorcluster, "UI Data Out"=w2204:T9, "outputCommandString"=w2206:string)  [unwired: 4 in]
            n1000 = local write "cB_commandLog"(w2206) -> ()
            n1001 = property on="cB_commandLog" class="Str"(error in=w2211, "Text.Scroll Position"=inf) -> ()  [unwired: 1 in, 2 out]
          }
        }
        n1002 = local write "pBot_ConnectButton"(FALSE ("pBot_ConnectButton")) -> ()
        n1003 = Merge Errors(w2139, w2140) -> (w2141:errorcluster)
      }
      frame "sendGCodeCommand" {
        n1004 = Variant To Data(error in=w2274, type="", Variant=w2273) -> (data=w2269:string, error out=w2263:errorcluster)
        n1005 = call <vilib>:"Trim Whitespace.vi"("string"=w2269) -> ("trimmed string"=w2266:string)  [unwired: 1 in]
        n1006 = Scan From String(format string="%s ", input string=w2266, error in=w2263) -> (remaining string=w2264:string, error out=w2262:errorcluster, output 1=w2265:string)  [unwired: 2 in, 1 out]
        n1007 = case shown="Default" w2265 {
          tunnel: w2283 -> [_ _ _ w2382]
          tunnel: [w2288 w2340 w2367 w2372] -> w2282
          tunnel: [w2289 w2348 w2369 w2374] -> w2275
          tunnel: w2262 -> [w2288 w2343 w2367 w2381]
          tunnel: w2266 -> [_ w2348 _ w2373]
          tunnel: w2272 -> [w2287 w2350 w2368 w2377]
          tunnel: w2264 -> [w2285 w2346 w2370 _]
          tunnel: [w2287 w2349 w2368 w2371] -> w2268
          tunnel: w2261 -> [_ w2339 _ _]
          frame "get" {
            # "Thiw will allow me an internal way of getting some values, but I wont tell people about it"
            n1008 = Scan From String(format string="%s ", input string=w2285) -> (output 1=w2284:string)  [unwired: 3 in, 3 out]
            n1009 = case shown="\"yPOI\"" w2284 {
              tunnel: w2287 -> [_ w2298 w2306 w2314 w2322 w2330 w2338]
              tunnel: ["" w2291 w2299 w2308 w2316 w2324 w2332] -> w2289
              frame "False", Default {
              }
              frame "yPOI" {
                n1010 = Unbundle By Name(w2298) -> ("yPOI"=w2292:cluster{"X":dbl, "Y":dbl, "Z":dbl})
                n1011 = Unbundle(w2292) -> ("X"=w2297:dbl, "Y"=w2295:dbl, "Z"=w2296:dbl)
                n1012 = Format Into String(format string="X %f Y %f Z %f", initial string="yPOI_Current", w2297, w2296, w2295) -> (resulting string=w2291:string)  [unwired: 1 in, 1 out]
              }
              frame "yPOI_0" {
                n1013 = Unbundle By Name(w2306) -> ("yPOI_0"=w2301:cluster{"X":dbl, "Y":dbl, "Z":dbl})
                n1014 = Unbundle(w2301) -> ("X"=w2305:dbl, "Y"=w2303:dbl, "Z"=w2304:dbl)
                n1015 = Format Into String(format string="X %f Y %f Z %f", initial string="yPOI_0: ", w2305, w2304, w2303) -> (resulting string=w2299:string)  [unwired: 1 in, 1 out]
              }
              frame "breadBoard_00" {
                n1016 = Unbundle By Name(w2314) -> ("breadBoard_00"=w2313:cluster{"X":dbl, "Y":dbl, "Z":dbl})
                n1017 = Unbundle(w2313) -> ("X"=w2312:dbl, "Y"=w2310:dbl, "Z"=w2311:dbl)
                n1018 = Format Into String(format string="X %f Y %f Z %f", initial string="breadBoard_00: ", w2312, w2311, w2310) -> (resulting string=w2308:string)  [unwired: 1 in, 1 out]
              }
              frame "pBot_homeOffset" {
                n1019 = Unbundle By Name(w2322) -> ("pBot_homeOffset"=w2321:cluster{"X":dbl, "Y":dbl, "Z":dbl})
                n1020 = Unbundle(w2321) -> ("X"=w2320:dbl, "Y"=w2318:dbl, "Z"=w2319:dbl)
                n1021 = Format Into String(format string="X %f Y %f Z %f", initial string="pBot_homeOffset: ", w2320, w2319, w2318) -> (resulting string=w2316:string)  [unwired: 1 in, 1 out]
              }
              frame "pBot_minPos" {
                n1022 = Unbundle By Name(w2330) -> ("pBot_minPos"=w2329:cluster{"X":dbl, "Y":dbl, "Z":dbl})
                n1023 = Unbundle(w2329) -> ("X"=w2328:dbl, "Y"=w2326:dbl, "Z"=w2327:dbl)
                n1024 = Format Into String(format string="X %f Y %f Z %f", initial string="pBot_minPos", w2328, w2327, w2326) -> (resulting string=w2324:string)  [unwired: 1 in, 1 out]
              }
              frame "pBot_maxPos" {
                n1025 = Unbundle By Name(w2338) -> ("pBot_maxPos"=w2337:cluster{"X":dbl, "Y":dbl, "Z":dbl})
                n1026 = Unbundle(w2337) -> ("X"=w2336:dbl, "Y"=w2334:dbl, "Z"=w2335:dbl)
                n1027 = Format Into String(format string="X %f Y %f Z %f", initial string="pBot_maxPos: ", w2336, w2335, w2334) -> (resulting string=w2332:string)  [unwired: 1 in, 1 out]
              }
            }
          }
          frame "set" {
            n1028 = Scan From String(format string="%s ", input string=w2346, error in=w2343) -> (remaining string=w2344:string, error out=w2341:errorcluster, output 1=w2345:string)  [unwired: 2 in, 1 out]
            n1029 = case shown="\"breadboard_pos\"" w2345 {
              tunnel: w2344 -> [_ w2363]
              tunnel: w2350 -> [w2352 w2364]
              tunnel: [w2352 w2364] -> w2349
              tunnel: [errorcluster {"status"=FALSE, "code"=0, "source"=""} ("error out") w2355] -> w2340
              tunnel: w2339 -> [_ w2365]
              tunnel: w2341 -> [_ w2355]
              frame Default {
              }
              frame "breadboard_pos" {
                # "set breadboard_pos X# Y# Z#\nSet the current location of the breadboard (in inches) relative to the 0,0 breadboard hole. X, Y, and Z are all optional (the current breadboard location will be used if one of them is not specified.)"
                n1030 = Unbundle By Name(w2364) -> ("yPOI"=w2357:cluster{"X":dbl, "Y":dbl, "Z":dbl}, "breadBoard_00"=w2358:cluster{"X":dbl, "Y":dbl, "Z":dbl})
                n1031 = call "string2vec.vi"("Default (nan,nan,nan)"=w2358, "input string"=w2363) -> ("isDefault"=w2353:cluster{bool, bool, bool}, "output"=w2359:cluster{"X":dbl, "Y":dbl, "Z":dbl})  [unwired: 8 in]
                n1032 = call "poly1.vi"("mask"=w2353, "Translation (0,0,0)"=w2357, "Multiplier (1,1,1)"=cluster{"X":dbl, "Y":dbl, "Z":dbl} {"X"=-25.4, "Y"=-25.4, "Z"=-25.4} ("Into to mm (minus)"), "input vector"=w2359) -> ("output"=w2361:cluster{"X":dbl, "Y":dbl, "Z":dbl})  [unwired: 6 in, 1 out]
                n1033 = call "vec2string.vi"("input vector"=w2361) -> ("output string"=w2362:string)  [unwired: 10 in]
                n1034 = Concatenate Strings("M206 " ("string"), w2362) -> (w2354:string)
                n1035 = call-poly "Enqueue Message.vi"("Message Data"=w2354, "Message"="sendGCodeCommand", "Message Queue"=w2365) -> ()  [unwired: 7 in, 2 out]
              }
            }
            n1036 = call-poly "Enqueue Message.vi"("Message"="update3DPicture", "Message Queue"=w2339) -> ()  [unwired: 8 in, 2 out]
          }
          frame "help" {
            # "help code"
            n1037 = call "gCode_Help.vi"("Input String"=w2370) -> ("stringOut"=w2369:string)  [unwired: 10 in]
          }
          frame Default {
            # "normal g-code ---- well not a \"get\" or a \"help\""
            n1038 = Get Queue Status(queue=w2382, error in (no error)=w2381) -> (queue out=w2378:refnum<queue>, error out=w2372:errorcluster, # elements in queue=w2379:i32)  [unwired: 1 in, 5 out]
            n1039 = Greater Than 0?(x=w2379) -> (x > 0?=w2380:bool)
            n1040 = call "gCode_AnalizeAndSend.vi"("UI_Data"=w2377, "Input String"=w2373, "Equip_Queue"=w2378) -> ("errorOut"=w2376:errorcluster, "UI_Data out"=w2371:T9)  [unwired: 7 in]
            n1041 = case shown="True" w2380 {
              tunnel: w2379 -> [_ w2394]
              tunnel: ["" w2393] -> w2375
              frame False {
              }
              frame True {
                n1042 = Format Into String(format string="...%d commands waiting.....", w2394) -> (resulting string=w2393:string)  [unwired: 2 in, 1 out]
              }
            }
            n1043 = case shown="No Error" w2376 {
              selector: w2376 -> [_ w2391]
              tunnel: w2375 -> [w2385 w2390]
              tunnel: w2373 -> [w2384 w2387]
              tunnel: [w2383 w2389] -> w2374
              frame No Error {
                n1044 = Concatenate Strings(w2384, w2385) -> (w2383:string)
              }
              frame Error {
                w2386 = "\n"
                n1045 = Unbundle(w2391) -> ("source"=w2388:string)  [unwired: 2 out]
                n1046 = Concatenate Strings(w2387, w2386, w2388, w2386, w2390) -> (w2389:string)
              }
            }
          }
        }
        n1047 = local read "numberOfCommandLines"() -> (w2278:i32)
        n1048 = local write "pBot_sendCommand"(FALSE ("pBot_sendCommand")) -> ()
        n1049 = local write "pBot_gcodeCommand"("") -> ()
        n1050 = call "setCommandString.vi"("numLines"=w2278, "stringToAdd"=w2275, "UI Data In"=w2268) -> ("error out"=w2280:errorcluster, "UI Data Out"=w2276:T9, "outputCommandString"=w2277:string)  [unwired: 6 in]
        n1051 = local write "cB_commandLog"(w2277) -> ()
        n1052 = property on="cB_commandLog" class="Str"(error in=w2280, "Text.Scroll Position"=inf) -> ()  [unwired: 1 in, 2 out]
      }
      frame "recieveMessageFromPBot" {
        n1053 = Variant To Data(error in=w2412, type=T15 {"commandID"=" ", "gCode"=" ", "extraInfo"=" ", "originatingCommandID"=" ", "error"={"status"=FALSE, "code"=0, "source"=""}}, Variant=w2411) -> (data=w2409:T15, error out=w2410:errorcluster)
        n1054 = call "gCode_analyseReceivedMessage.vi"("UI_Data"=w2408, "pBotMessageData"=w2409) -> ("error Out"=w2403:errorcluster, "UI_Data Out"=w2399:T9, "messageOut"=w2404:string)  [unwired: 7 in]
        n1055 = local read "numberOfCommandLines"() -> (w2406:i32)
        n1056 = call "setCommandString.vi"("addLF_onlyIfNeeded? (T)"=TRUE, "addLF? (T)"=TRUE ("addLF?"), "addTimeAndChevron? (T)"=TRUE ("addTimeAndChevron?"), "numLines"=w2406, "stringToAdd"=w2404, "UI Data In"=w2399) -> ("UI Data Out"=w2402:T9, "outputCommandString"=w2397:string)  [unwired: 3 in, 1 out]
        n1057 = property on="cB_commandLog" class="Str"("Text.Text"=w2397, "Text.Scroll Position"=inf) -> ()  [unwired: 2 in, 2 out]
        n1058 = case shown="Error" w2403 {
          selector: w2403 -> [_ w2419]
          tunnel: w2402 -> [w2413 w2420]
          tunnel: [w2413 w2417] -> w2400
          frame No Error {
          }
          frame Error {
            n1059 = Unbundle(w2419) -> ("source"=w2418:string)  [unwired: 2 out]
            n1060 = local read "numberOfCommandLines"() -> (w2422:i32)
            n1061 = call "setCommandString.vi"("addLF_onlyIfNeeded? (T)"=TRUE, "addLF? (T)"=TRUE ("addLF?"), "addTimeAndChevron? (T)"=TRUE ("addTimeAndChevron?"), "numLines"=w2422, "stringToAdd"=w2418, "UI Data In"=w2420) -> ("UI Data Out"=w2417:T9, "outputCommandString"=w2414:string)  [unwired: 3 in, 1 out]
            n1062 = property on="cB_commandLog" class="Str"("Text.Text"=w2414, "Text.Scroll Position"=inf) -> ()  [unwired: 2 in, 2 out]
          }
        }
      }
      frame "getCurrentInfo" {
        n1063 = Variant To Data(error in=w2435, type=T16 {"currentPos"={"X"=0.0, "Y"=0.0, "Z"=0.0}, "temperature"=0.0, "error constant"={"status"=FALSE, "code"=0, "source"=""}}, Variant=w2434) -> (data=w2431:T16, error out=w2426:errorcluster)
        n1064 = Unbundle(w2431) -> ("currentPos"=w2429:cluster{"X":dbl, "Y":dbl, "Z":dbl}, "temperature"=w2428:dbl, "error constant"=w2430:errorcluster)
        n1065 = case shown="No Error" w2430 {
          selector: w2430 -> [_ w2465]
          tunnel: w2433 -> [w2459 w2464]
          tunnel: w2429 -> [w2438 _]
          tunnel: w2428 -> [w2444 _]
          tunnel: [w2447 w2463] -> w2427
          tunnel: w2426 -> [w2451 w2462]
          tunnel: [w2450 w2462] -> w2425
          tunnel: w2424 -> [w2449 _]
          frame No Error {
            n1066 = Unbundle By Name(w2459) -> ("realTimeInfoTextColor"=w2458:u32[], "textColorGray"=w2457:u32, "yPOI_0"=w2442:cluster{"X":dbl, "Y":dbl, "Z":dbl}, "3DPictureObjRef"=w2443:refnum<vi>, "transVisualizationControls"=w2445:refnum<vi>[], "breadBoard_00"=w2440:cluster{"X":dbl, "Y":dbl, "Z":dbl})
            n1067 = call-poly "flipYZ.vi"("pointIn"=w2438) -> ("pointOut"=w2437:cluster{"X":dbl, "Y":dbl, "Z":dbl})  [unwired: 10 in]
            n1068 = Cluster To Array(cluster=w2437) -> (array=w2446:dbl[])
            n1069 = for {
              tunnel: w2445 -> [w2461] mode=indexing
              tunnel: w2446 -> [w2460] mode=indexing
              n1070 = property class="Knob (strict)"(reference=w2461, "Value"=w2460) -> ()  [unwired: 1 in, 2 out]
            }
            n1071 = Replace Array Subset(array=w2458, new element=w2457, index=3) -> (w2455:u32[])
            n1072 = call-poly "Enqueue Message.vi"("error in (no error)"=w2451, "Message"="update3DPicture", "Message Queue"=w2449) -> ("error out"=w2450:errorcluster)  [unwired: 7 in, 1 out]
            n1073 = call <vilib>:"Find Object.vi"("Object Name"="yArm", "Scene Refnum"=w2443) -> ("Object Refnum"=w2453:refnum<vi>)  [unwired: 8 in, 1 out]
            n1074 = Add(x=w2438, y=w2442) -> (x+y=w2436:cluster{"X":dbl, "Y":dbl, "Z":dbl})
            n1075 = Bundle By Name(cluster=w2459, "pBot_tempSensor1"=w2444, "realTimeInfoTextColor"=w2455, "yPOI"=w2436) -> (w2447:T9)
            n1076 = Negate(x=w2436) -> (-x=w2441:cluster{"X":dbl, "Y":dbl, "Z":dbl})
            n1077 = Add(x=w2441, y=w2440) -> (x+y=w2439:cluster{"X":dbl, "Y":dbl, "Z":dbl})
            n1078 = call "translateObj.vi"("POI_proj_Offset (0,0,0)"=w2439, "vector"=w2438, "Type"="ta", "Scene: Object"=w2453) -> ()  [unwired: 6 in, 2 out]
            n1079 = call "updateRealTimeInfo.vi"("UI_Data"=w2447) -> ()  [unwired: 11 in]
          }
          frame Error {
            n1080 = Unbundle(w2465) -> ("source"=w2469:string)  [unwired: 2 out]
            n1081 = local read "numberOfCommandLines"() -> (w2471:i32)
            n1082 = call "setCommandString.vi"("addLF_onlyIfNeeded? (T)"=TRUE, "addLF? (T)"=TRUE ("addLF?"), "addTimeAndChevron? (T)"=TRUE ("addTimeAndChevron?"), "numLines"=w2471, "stringToAdd"=w2469, "UI Data In"=w2464) -> ("UI Data Out"=w2463:T9, "outputCommandString"=w2466:string)  [unwired: 3 in, 1 out]
            n1083 = property on="cB_commandLog" class="Str"("Text.Text"=w2466, "Text.Scroll Position"=inf) -> ()  [unwired: 2 in, 2 out]
          }
        }
      }
      frame "updateXYmoveDisplay" {
        n1084 = Variant To Data(error in=w2478, type="", Variant=w2477) -> (data=w2475:string, error out=w2474:errorcluster)
        n1085 = property on="pBot_xyMoveDisplay" class="Str"(error in=w2474, "Text.Text"=w2475) -> (error out=w2473:errorcluster)  [unwired: 1 in, 1 out]
      }
      frame "updateZmoveDisplay" {
        n1086 = Variant To Data(error in=w2485, type="", Variant=w2484) -> (data=w2482:string, error out=w2481:errorcluster)
        n1087 = property on="pBot_zMoveDisplay" class="Str"(error in=w2481, "Text.Text"=w2482) -> (error out=w2480:errorcluster)  [unwired: 1 in, 1 out]
      }
      frame "homePBotAxis" {
        n1088 = Variant To Data(error in=w2496, type=enum16{"Y", "X", "Z"}."Y", Variant=w2495) -> (data=w2490:enum16{"Y", "X", "Z"}, error out=w2491:errorcluster)
        n1089 = case shown="\"X\"" w2490 {
          tunnel: w2493 -> [w2507 w2509 w2534]
          tunnel: [w2506 w2508 w2536] -> w2492
          tunnel: w2489 -> [w2504 w2513 w2537]
          tunnel: [w2497 w2511 w2532] -> w2487
          frame "Y" {
            n1090 = Bundle By Name(cluster=w2507, "needToHomeY?"=FALSE) -> (w2506:T9)
            n1091 = Bundle By Name(cluster=T15 {"commandID"=" ", "gCode"=" ", "extraInfo"=" ", "originatingCommandID"=" ", "error"={"status"=FALSE, "code"=0, "source"=""}} ("pBotMessageData"), "gCode"="G28 Y0" ("Message"), "commandID"="homeY" ("extraInfo")) -> (w2499:T15)
            n1092 = call-poly "Enqueue Message.vi"("Message Data"=w2499, "Message"="sendGCodeCommand", "Message Queue"=w2504) -> ("dup Message Queue"=w2497:refnum<queue>)  [unwired: 7 in, 1 out]
            n1093 = local write "pBot_yHome"(FALSE ("pBot_yHome")) -> ()
          }
          frame "Z" {
            n1094 = local write "pBot_zHome"(FALSE ("pBot_yHome")) -> ()
            n1095 = Unbundle By Name(w2509) -> ("needToHomeXY?"=w2510:bool)
            n1096 = case shown="True" w2510 {
              tunnel: w2513 -> [w2520 w2531]
              tunnel: [w2515 w2531] -> w2511
              tunnel: w2509 -> [w2514 w2523]
              tunnel: [w2514 w2522] -> w2508
              frame False {
                n1097 = Bundle By Name(cluster=T15 {"commandID"=" ", "gCode"=" ", "extraInfo"=" ", "originatingCommandID"=" ", "error"={"status"=FALSE, "code"=0, "source"=""}} ("pBotMessageData"), "gCode"="G28 Z0" ("Message"), "commandID"="homeZ" ("extraInfo")) -> (w2516:T15)
                n1098 = call-poly "Enqueue Message.vi"("Message Data"=w2516, "Message"="sendGCodeCommand", "Message Queue"=w2520) -> ("dup Message Queue"=w2515:refnum<queue>)  [unwired: 7 in, 1 out]
              }
              frame True {
                n1099 = local read "numberOfCommandLines"() -> (w2528:i32)
                n1100 = call "setCommandString.vi"("addLF_onlyIfNeeded? (T)"=TRUE, "addLF? (T)"=TRUE ("addLF?"), "addTimeAndChevron? (T)"=TRUE ("addTimeAndChevron?"), "numLines"=w2528, "stringToAdd"="Home Y/X before Z", "UI Data In"=w2523) -> ("UI Data Out"=w2522:T9, "outputCommandString"=w2524:string)  [unwired: 3 in, 1 out]
                n1101 = property on="cB_commandLog" class="Str"("Text.Text"=w2524, "Text.Scroll Position"=inf) -> ()  [unwired: 2 in, 2 out]
              }
            }
          }
          frame "X" {
            n1102 = Unbundle By Name(w2534) -> ("needToHomeY?"=w2533:bool)
            n1103 = local write "pBot_xHome"(FALSE ("pBot_yHome")) -> ()
            n1104 = case shown="False" w2533 {
              tunnel: w2537 -> [w2543 w2548]
              tunnel: w2534 -> [w2540 w2552]
              tunnel: [w2538 w2550] -> w2536
              tunnel: [w2541 w2548] -> w2532
              frame False {
                n1105 = Bundle By Name(cluster=T15 {"commandID"=" ", "gCode"=" ", "extraInfo"=" ", "originatingCommandID"=" ", "error"={"status"=FALSE, "code"=0, "source"=""}} ("pBotMessageData"), "gCode"="G28 X0" ("Message"), "commandID"="homeX" ("extraInfo")) -> (w2544:T15)
                n1106 = call-poly "Enqueue Message.vi"("Message Data"=w2544, "Message"="sendGCodeCommand", "Message Queue"=w2543) -> ("dup Message Queue"=w2541:refnum<queue>)  [unwired: 7 in, 1 out]
                n1107 = Bundle By Name(cluster=w2540, "needToHomeXY?"=FALSE) -> (w2538:T9)
              }
              frame True {
                n1108 = local read "numberOfCommandLines"() -> (w2555:i32)
                n1109 = call "setCommandString.vi"("addLF_onlyIfNeeded? (T)"=TRUE, "addLF? (T)"=TRUE ("addLF?"), "addTimeAndChevron? (T)"=TRUE ("addTimeAndChevron?"), "numLines"=w2555, "stringToAdd"="Home Y before X", "UI Data In"=w2552) -> ("UI Data Out"=w2550:T9, "outputCommandString"=w2549:string)  [unwired: 3 in, 1 out]
                n1110 = property on="cB_commandLog" class="Str"("Text.Text"=w2549, "Text.Scroll Position"=inf) -> ()  [unwired: 2 in, 2 out]
              }
            }
          }
        }
        n1111 = call-poly "Enqueue Message.vi"("Message"="getCurrentInfo", "Message Queue"=w2487) -> ()  [unwired: 8 in, 2 out]
      }
      frame "moveRelative" {
        w2558 = TRUE ("needToHomeY?")
        w2567 = "sendGCodeCommand" ("Message")
        # "turn all of the boolian pBot_controls to false. I don't think this will give an error but if it does give some weird errors then i'll need to seperate the relative motion controls from the others and then just set all of the relative motion controls to false"
        n1112 = Variant To Data(error in=w2575, type=T12 {"Direction"=enum."Y", "Amount"=-0.1} ("relativeMoveData"), Variant=w2574) -> (data=w2572:T12, error out=w2562:errorcluster)
        n1113 = Unbundle By Name(w2572) -> ("Amount"=w2568:dbl, "Direction"=w2569:enum16{"Y", "X", "Z"})
        n1114 = Unbundle By Name(w2560) -> ("pBot_controls"=w2559:refnum<vi>[])
        n1115 = call-poly "Enqueue Message.vi"("Message Data"="G91" ("Message"), "Message"=w2567, "Message Queue"=w2571) -> ("dup Message Queue"=w2566:refnum<queue>)  [unwired: 7 in, 1 out]
        n1116 = case shown="\"Z\"" w2569 {
          tunnel: w2568 -> [w2585 w2591 w2597]
          tunnel: w2567 -> [w2581 w2587 w2593]
          tunnel: w2566 -> [w2584 w2590 w2596]
          tunnel: [w2582 w2588 w2594] -> w2565
          tunnel: [w2581 w2587 w2593] -> w2564
          frame "X" {
            n1117 = Format Into String(format string="G1 X%0.3f", w2585) -> (resulting string=w2583:string)  [unwired: 2 in, 1 out]
            n1118 = call-poly "Enqueue Message.vi"("Message Data"=w2583, "Message"=w2581, "Message Queue"=w2584) -> ("dup Message Queue"=w2582:refnum<queue>)  [unwired: 7 in, 1 out]
          }
          frame "Y" {
            n1119 = Format Into String(format string="G1 Y%0.3f", w2591) -> (resulting string=w2589:string)  [unwired: 2 in, 1 out]
            n1120 = call-poly "Enqueue Message.vi"("Message Data"=w2589, "Message"=w2587, "Message Queue"=w2590) -> ("dup Message Queue"=w2588:refnum<queue>)  [unwired: 7 in, 1 out]
          }
          frame "Z" {
            n1121 = Format Into String(format string="G1 Z%0.3f", w2597) -> (resulting string=w2595:string)  [unwired: 2 in, 1 out]
            n1122 = call-poly "Enqueue Message.vi"("Message Data"=w2595, "Message"=w2593, "Message Queue"=w2596) -> ("dup Message Queue"=w2594:refnum<queue>)  [unwired: 7 in, 1 out]
          }
        }
        n1123 = for {
          tunnel: w2559 -> [w2576] mode=indexing
          n1124 = property class="Ctl"(reference=w2576) -> (reference out=w2577:refnum<vi>, "ClassID"=w2578:u32)  [unwired: 1 in, 1 out]
          n1125 = case shown="8" w2578 {
            tunnel: w2577 -> [_ w2580]
            frame Default {
            }
            frame 8 {
              n1126 = property class="Ctl"(reference=w2580, "Value"=FALSE) -> ()  [unwired: 1 in, 2 out]
            }
          }
        }
        n1127 = call-poly "Enqueue Message.vi"("Message Data"="G90" ("Message"), "Message"=w2564, "Message Queue"=w2565) -> ()  [unwired: 7 in, 2 out]
        n1128 = Bundle By Name(cluster=w2560, "needToHomeXY?"=w2558, "needToHomeY?"=w2558) -> (w2561:T9)
      }
      frame "updateScanRegion" {
        n1129 = local read "pBot_scanningXmax"() -> (w2606:sgl)
        n1130 = local read "pBot_scanningYmax"() -> (w2607:sgl)
        n1131 = local read "pBot_scanningZmax"() -> (w2605:sgl)
        n1132 = local read "pBot_scanningXmin"() -> (w2603:sgl)
        n1133 = local read "pBot_scanningYmin"() -> (w2604:sgl)
        n1134 = local read "pBot_scanningZmin"() -> (w2602:sgl)
        n1135 = local read "pBot_scanNx"() -> (w2622:u16)
        n1136 = local read "pBot_scanNy"() -> (w2623:u16)
        n1137 = local read "pBot_scanNz"() -> (w2621:u16)
        n1138 = Bundle(cluster=cluster{"X":u16, "Y":u16, "Z":u16} {"X"=0, "Y"=0, "Z"=0} ("unsigned 32bit integer"), "X"=w2622, "Y"=w2623, "Z"=w2621) -> (w2620:cluster{"X":u16, "Y":u16, "Z":u16})
        n1139 = Bundle(cluster=cluster{"X":sgl, "Y":sgl, "Z":sgl} {"X"=0.0, "Y"=0.0, "Z"=0.0} ("pBot_minScanRegion"), "X"=w2603, "Y"=w2604, "Z"=w2602) -> (w2600:cluster{"X":sgl, "Y":sgl, "Z":sgl})
        n1140 = Bundle(cluster=cluster{"X":sgl, "Y":sgl, "Z":sgl} {"X"=0.0, "Y"=0.0, "Z"=0.0} ("pBot_maxScanRegion"), "X"=w2606, "Y"=w2607, "Z"=w2605) -> (w2599:cluster{"X":sgl, "Y":sgl, "Z":sgl})
        n1141 = Less Or Equal?(x=w2599, y=w2600) -> (x <= y?=w2627:cluster{"X":bool, "Y":bool, "Z":bool})
        n1142 = Cluster To Array(cluster=w2627) -> (array=w2626:bool[])
        n1143 = Or Array Elements(Boolean array=w2626) -> (logical OR=w2625:bool)
        n1144 = case shown="False" w2625 {
          tunnel: w2601 -> [w2660 w2670]
          tunnel: w2599 -> [w2652 _]
          tunnel: w2600 -> [w2651 _]
          tunnel: [w2650 w2670] -> w2610
          tunnel: w2620 -> [w2632 _]
          tunnel: [w2631 "The maximum must be greater than or equal to the smaller value. The maximum resolution is about 0.1 mm."] -> w2608
          tunnel: w2619 -> [w2648 _]
          tunnel: w2618 -> [w2647 w2669]
          tunnel: [w2646 w2669] -> w2617
          frame False {
            n1145 = Unbundle By Name(w2660) -> ("3DPictureObjRef"=w2666:refnum<vi>, "yPOI_0"=w2638:cluster{"X":dbl, "Y":dbl, "Z":dbl})
            n1146 = Add(x=w2652, y=w2651) -> (x+y=w2661:cluster{"X":sgl, "Y":sgl, "Z":sgl})
            n1147 = Subtract(x=w2652, y=w2651) -> (x-y=w2643:cluster{"X":sgl, "Y":sgl, "Z":sgl})
            n1148 = Add(x=sgl 1.1920929e-07, y=w2643) -> (x+y=w2642:cluster{"X":sgl, "Y":sgl, "Z":sgl})
            n1149 = Divide(x=w2661, y=sgl 2.0) -> (x/y=w2654:cluster{"X":sgl, "Y":sgl, "Z":sgl})
            n1150 = Multiply(x=w2643, y=10.0) -> (x*y=w2658:cluster{"X":dbl, "Y":dbl, "Z":dbl})
            n1151 = call-poly "flipYZ.vi"("pointIn"=w2654) -> ("pointOut"=w2640:cluster{"X":sgl, "Y":sgl, "Z":sgl})  [unwired: 10 in]
            n1152 = Round Toward -Infinity(1:w2658) -> (0:w2645:cluster{"X":dbl, "Y":dbl, "Z":dbl})
            n1153 = call <vilib>:"Find Object.vi"("Object Name"="scanRegion", "Scene Refnum"=w2666) -> ("Object Refnum"=w2664:refnum<vi>)  [unwired: 8 in, 1 out]
            n1154 = call-poly "flipYZ.vi"("pointIn"=w2642) -> ("pointOut"=w2653:cluster{"X":sgl, "Y":sgl, "Z":sgl})  [unwired: 10 in]
            n1155 = To Unsigned Word Integer(number=w2645) -> (unsigned 16bit integer=w2644:cluster{"X":u16, "Y":u16, "Z":u16})
            n1156 = call <vilib>:"Set Scale.vi"("Scale"=w2653, "Scene Object"=w2664) -> ("error out"=w2663:errorcluster)  [unwired: 8 in, 1 out]
            n1157 = Increment(x=w2644) -> (x+1=w2630:cluster{"X":u16, "Y":u16, "Z":u16})
            n1158 = Add(x=w2638, y=w2640) -> (x+y=w2639:cluster{"X":dbl, "Y":dbl, "Z":dbl})
            n1159 = call <vilib>:"Set Translation.vi"("error in (no error)"=w2663, "Translation"=w2639, "Scene Object"=w2664) -> ()  [unwired: 7 in, 2 out]
            n1160 = In Range and Coerce(upper limit=w2630, x=w2632, lower limit=u16 1) -> (coerced(x)=w2633:cluster{"X":u16, "Y":u16, "Z":u16}, In Range?=w2636:cluster{"X":bool, "Y":bool, "Z":bool})
            n1161 = call-poly "Enqueue Message.vi"("error in (no error)"=w2647, "Message"="update3DPicture", "Message Queue"=w2648) -> ("error out"=w2646:errorcluster)  [unwired: 7 in, 1 out]
            n1162 = Cluster To Array(cluster=w2636) -> (array=w2635:bool[])
            n1163 = And Array Elements(Boolean array=w2635) -> (logical AND=w2634:bool)
            n1164 = Unbundle(w2633) -> ("X"=w2656:u16, "Y"=w2657:u16, "Z"=w2655:u16)
            n1165 = case shown="False" w2634 {
              tunnel: ["Warning! Number of scan points adjusted. \nThe step size must be at least 0.1 (which is about the resolution of the instrument), and the number of scan points in each dimension must be greater than 0." ""] -> w2631
              frame False {
              }
              frame True {
              }
            }
            n1166 = local write "pBot_scanNx"(w2656) -> ()
            n1167 = local write "pBot_scanNy"(w2657) -> ()
            n1168 = local write "pBot_scanNz"(w2655) -> ()
            n1169 = Bundle By Name(cluster=w2660, "pBot_maxScanRegion"=w2652, "pBot_minScanRegion"=w2651, "pBot_scanN"=w2633) -> (w2650:T9)
          }
          frame True {
            n1170 = Unbundle By Name(w2670) -> ("pBot_maxScanRegion"=w2683:cluster{"X":sgl, "Y":sgl, "Z":sgl}, "pBot_minScanRegion"=w2682:cluster{"X":sgl, "Y":sgl, "Z":sgl}, "pBot_scanN"=w2681:cluster{"X":u16, "Y":u16, "Z":u16})
            n1171 = Unbundle(w2683) -> ("X"=w2680:sgl, "Y"=w2679:sgl, "Z"=w2678:sgl)
            n1172 = Unbundle(w2682) -> ("X"=w2677:sgl, "Y"=w2676:sgl, "Z"=w2675:sgl)
            n1173 = Unbundle(w2681) -> ("X"=w2674:u16, "Y"=w2673:u16, "Z"=w2672:u16)
            n1174 = local write "pBot_scanningXmax"(w2680) -> ()
            n1175 = local write "pBot_scanningYmax"(w2679) -> ()
            n1176 = local write "pBot_scanningZmax"(w2678) -> ()
            n1177 = local write "pBot_scanningXmin"(w2677) -> ()
            n1178 = local write "pBot_scanningYmin"(w2676) -> ()
            n1179 = local write "pBot_scanningZmin"(w2675) -> ()
            n1180 = local write "pBot_scanNx"(w2674) -> ()
            n1181 = local write "pBot_scanNy"(w2673) -> ()
            n1182 = local write "pBot_scanNz"(w2672) -> ()
          }
        }
        n1183 = local read "numberOfCommandLines"() -> (w2614:i32)
        n1184 = call "setCommandString.vi"("addLF_onlyIfNeeded? (T)"=TRUE, "addLF? (T)"=TRUE ("addLF?"), "addTimeAndChevron? (T)"=TRUE ("addTimeAndChevron?"), "numLines"=w2614, "stringToAdd"=w2608, "UI Data In"=w2610) -> ("UI Data Out"=w2609:T9, "outputCommandString"=w2611:string)  [unwired: 3 in, 1 out]
        n1185 = property on="cB_commandLog" class="Str"("Text.Text"=w2611, "Text.Scroll Position"=inf) -> ()  [unwired: 2 in, 2 out]
      }
      frame "startScan" {
        # "Change the start scan button boolian text to stop scan.\ncreate a 3D array with all of the positions of the scan\nsend this 3D array along with the string of the instument to use as message data to the Equip Loop with the message \"startScan\""
        # "initiate a scan"
        n1186 = Unbundle By Name(w2695) -> ("yPOI"=w2691:cluster{"X":dbl, "Y":dbl, "Z":dbl}, "yPOI_0"=w2690:cluster{"X":dbl, "Y":dbl, "Z":dbl}, "pBot_maxScanRegion"=w2696:cluster{"X":sgl, "Y":sgl, "Z":sgl}, "pBot_minScanRegion"=w2697:cluster{"X":sgl, "Y":sgl, "Z":sgl}, "pBot_scanN"=w2698:cluster{"X":u16, "Y":u16, "Z":u16}, "pBot_maxPos"=w2685:cluster{"X":dbl, "Y":dbl, "Z":dbl}, "pBot_minPos"=w2684:cluster{"X":dbl, "Y":dbl, "Z":dbl}, "connectedInstruments"=w2692:T7[], "isScanning?"=w2688:bool, "pBot_controls"=w2686:refnum<vi>[], "usb2000p_controlRefs"=w2687:refnum<vi>[])
        n1187 = case shown="False" w2688 {
          tunnel: w2698 -> [w2718 _]
          tunnel: w2697 -> [w2700 _]
          tunnel: w2696 -> [w2701 _]
          tunnel: w2695 -> [w2714 w2788]
          tunnel: [w2713 w2788] -> w2694
          tunnel: w2693 -> [w2712 w2792]
          tunnel: w2692 -> [w2711 _]
          tunnel: w2691 -> [w2710 _]
          tunnel: w2690 -> [w2709 _]
          tunnel: w2687 -> [w2708 _]
          tunnel: w2686 -> [w2707 _]
          tunnel: w2685 -> [w2703 _]
          tunnel: w2684 -> [w2702 _]
          frame False {
            n1188 = Subtract(x=w2710, y=w2709) -> (x-y=w2706:cluster{"X":dbl, "Y":dbl, "Z":dbl})
            n1189 = call-poly "flipYZ.vi"("pointIn"=w2706) -> ("pointOut"=w2705:cluster{"X":dbl, "Y":dbl, "Z":dbl})  [unwired: 10 in]
            n1190 = Subtract(x=w2703, y=w2702) -> (x-y=w2704:cluster{"X":dbl, "Y":dbl, "Z":dbl})
            n1191 = In Range and Coerce(upper limit=w2701, x=w2705, lower limit=w2700) -> (In Range?=w2717:cluster{"X":bool, "Y":bool, "Z":bool})  [unwired: 1 out]
            n1192 = Cluster To Array(cluster=w2717) -> (array=w2715:bool[])
            n1193 = And Array Elements(Boolean array=w2715) -> (logical AND=w2716:bool)
            n1194 = case shown="True" w2716 {
              tunnel: w2718 -> [_ w2751]
              tunnel: w2700 -> [_ w2750]
              tunnel: w2701 -> [_ w2749]
              tunnel: w2714 -> [w2721 w2732]
              tunnel: [w2720 w2731] -> w2713
              tunnel: w2712 -> [_ w2734]
              tunnel: w2711 -> [_ w2733]
              tunnel: w2708 -> [_ w2730]
              tunnel: w2707 -> [_ w2729]
              tunnel: w2704 -> [_ w2728]
              frame False {
                n1195 = local read "numberOfCommandLines"() -> (w2722:i32)
                n1196 = call "setCommandString.vi"("addLF_onlyIfNeeded? (T)"=TRUE, "addLF? (T)"=TRUE ("addLF?"), "addTimeAndChevron? (T)"=TRUE ("addTimeAndChevron?"), "numLines"=w2722, "stringToAdd"="Error! You must first position the plasmaBot head inside of the scan region. That is, the position given on the top of the screen must be inside of the scan region.\n\nYou have to do this because the program does not to any path planning.", "UI Data In"=w2721) -> ("UI Data Out"=w2720:T9, "outputCommandString"=w2723:string)  [unwired: 3 in, 1 out]
                n1197 = property on="cB_commandLog" class="Str"("Text.Text"=w2723, "Text.Scroll Position"=inf) -> ()  [unwired: 2 in, 2 out]
              }
              frame True {
                n1198 = Get Date/Time In Seconds() -> (seconds since 1Jan1904=w2741:timestamp)
                n1199 = Format Date/Time String(time format string (%c)="%Y%m%d_%H%M%S", seconds (now)=w2741) -> (date/time string=w2744:string)  [unwired: 1 in]
                n1200 = Concatenate Strings("scanData_" ("default name"), w2744, ".h5" ("default name")) -> (w2746:string)
                n1201 = call "File Dialog"("prompt"="Select a file to save the data to.", "default name"=w2746, "pattern (all files)"="*.h5", "pattern label"="HDF5 Data File") -> ("selected path"=w2735:path, "cancelled"=w2738:bool, "error out"=w2748:errorcluster)  [unwired: 8 in, 1 out]
                n1202 = Unbundle(w2748) -> ("status"=w2737:bool)  [unwired: 2 out]
                n1203 = Or(x=w2738, y=w2737) -> (x .or. y?=w2736:bool)
                n1204 = case shown="False" w2736 {
                  tunnel: w2751 -> [w2760 _]
                  tunnel: w2750 -> [w2771 _]
                  tunnel: w2749 -> [w2770 _]
                  tunnel: w2735 -> [w2768 _]
                  tunnel: w2734 -> [w2764 _]
                  tunnel: w2733 -> [w2765 _]
                  tunnel: w2732 -> [w2757 w2787]
                  tunnel: [w2756 w2787] -> w2731
                  tunnel: w2730 -> [w2754 _]
                  tunnel: w2729 -> [w2755 _]
                  tunnel: w2728 -> [w2752 _]
                  frame False {
                    n1205 = call "createScanPoints.vi"("travelRange"=w2752, "pBot_scanN"=w2760, "pBot_minScanRegion"=w2771, "pBot_maxScanRegion"=w2770) -> ("scanPoints"=w2767:T19)  [unwired: 7 in]
                    n1206 = property on="pBot_scanInstrument" class="CmbBox"() -> ("Value"=w2766:string)  [unwired: 2 in, 2 out]
                    n1207 = case shown="Default" w2766 {
                      selector: w2766 -> [_ w2781]
                      tunnel: w2765 -> [_ w2782]
                      tunnel: [w2777 w2780] -> w2761
                      frame "None" {
                        n1208 = Bundle By Name(cluster=T7 {"Name"="", "VISAname"="", "1D_dataArraySize"=0, "extraInfo"=variant, "error"={"status"=FALSE, "code"=0, "source"=""}} ("scanInstrumentInfo"), "Name"="") -> (w2777:T7)
                      }
                      frame Default {
                        n1209 = for {
                          tunnel: w2782 -> [w2783] mode=indexing
                          tunnel: w2781 -> [w2785]
                          tunnel: [w2783] -> w2780
                          stop <- w2784 stop-if-true
                          n1210 = Unbundle By Name(w2783) -> ("Name"=w2786:string)
                          n1211 = Equal?(x=w2786, y=w2785) -> (x = y?=w2784:bool)
                        }
                      }
                    }
                    n1212 = for {
                      tunnel: w2755 -> [w2772] mode=indexing
                      n1213 = call-poly <userlib>:"MGI Disable Enum (Small).vi"() -> ("Disabled & Grayed"=w2773:T22)
                      n1214 = property class="Ctl"(reference=w2772, "DisabledEnum"=w2773) -> ()  [unwired: 1 in, 2 out]
                    }
                    n1215 = for {
                      tunnel: w2754 -> [w2774] mode=indexing
                      n1216 = call-poly <userlib>:"MGI Disable Enum (Small).vi"() -> ("Disabled & Grayed"=w2775:T22)
                      n1217 = property class="Ctl"(reference=w2774, "DisabledEnum"=w2775) -> ()  [unwired: 1 in, 2 out]
                    }
                    n1218 = Bundle By Name(cluster=T6 {"dataFilePath"=path "", "scanPoints"={"dim1"=[], "dim2"=[], "dim3"=[]}, "N"={"X"=0, "Y"=0, "Z"=0}, "scanInstrumentInfo"={"Name"="", "VISAname"="", "1D_dataArraySize"=0, "extraInfo"=variant, "error"={"status"=FALSE, "code"=0, "source"=""}}}, "dataFilePath"=w2768, "scanPoints"=w2767, "N"=w2760, "scanInstrumentInfo"=w2761) -> (w2762:T6)
                    n1219 = local read "textColorRed"() -> (w2758:u32)
                    n1220 = in-place {
                      n1221 = in-place-cluster #11(w2757) -> ()  [unwired: 1 out]
                      n1222 = in-place-cluster #11("isScanning?"=TRUE) -> (w2756:T9)
                    }
                    n1223 = property on="pBot_runScan" class="Bool (strict)"("BoolText.Text"="Stop Scan" ("Boolean Text.Text"), "BoolText.TextColor"=w2758) -> ()  [unwired: 2 in, 2 out]
                    n1224 = local write "usb2000p_continuous?"(FALSE ("usb2000p_continuous?")) -> ()
                    n1225 = call-poly "Enqueue Message.vi"("Message Data"=w2762, "Message"="startScan", "Message Queue"=w2764) -> ()  [unwired: 7 in, 2 out]
                  }
                  frame True {
                  }
                }
              }
            }
          }
          frame True {
            n1226 = Flush Queue(queue=w2792) -> (queue out=w2791:refnum<queue>)  [unwired: 1 in, 2 out]
            n1227 = call-poly "Enqueue Message.vi"("Message Data"=errorcluster {"status"=TRUE, "code"=0, "source"="Scan terminated successfully!"} ("error constant"), "Message"="scanComplete", "Message Queue"=w2791) -> ()  [unwired: 7 in, 2 out]
          }
        }
        n1228 = local write "pBot_runScan"(FALSE ("pBot_runScan")) -> ()
      }
      frame "scanEnded" {
        n1229 = Variant To Data(error in=w2813, type=errorcluster {"status"=FALSE, "code"=0, "source"=""} ("error constant"), Variant=w2812) -> (data=w2810:errorcluster, error out=w2795:errorcluster)
        n1230 = Unbundle By Name(w2796) -> ("pBotConnected?"=w2797:bool, "pBot_controls"=w2793:refnum<vi>[], "usb2000p_controlRefs"=w2794:refnum<vi>[])
        n1231 = in-place {
          n1232 = in-place-cluster #12(w2796) -> ()  [unwired: 1 out]
          n1233 = in-place-cluster #12("isScanning?"=FALSE) -> (w2799:T9)
        }
        n1234 = case shown="Error" w2810 {
          selector: w2810 -> [_ w2823]
          tunnel: ["Scan complete!" ("source") w2822] -> w2803
          tunnel: w2798 -> [_ w2821]
          tunnel: w2797 -> [_ w2820]
          frame No Error {
          }
          frame Error {
            n1235 = Unbundle By Name(w2823) -> ("source"=w2822:string)
            n1236 = case shown="True" w2820 {
              tunnel: w2821 -> [_ w2825]
              frame False {
              }
              frame True {
                n1237 = call-poly "Enqueue Message.vi"("Message"="getCurrentInfo", "Message Queue"=w2825) -> ()  [unwired: 8 in, 2 out]
              }
            }
          }
        }
        n1238 = for {
          tunnel: w2793 -> [w2817] mode=indexing
          n1239 = property class="Ctl"(reference=w2817, "DisabledEnum"=T22."Enabled" ("Disabled")) -> ()  [unwired: 1 in, 2 out]
        }
        n1240 = for {
          tunnel: w2794 -> [w2815] mode=indexing
          n1241 = property class="Ctl"(reference=w2815, "DisabledEnum"=T22."Enabled" ("Disabled")) -> ()  [unwired: 1 in, 2 out]
        }
        n1242 = local read "textColorGreen"() -> (w2800:u32)
        n1243 = property on="pBot_runScan" class="Bool (strict)"("BoolText.Text"="Start scan" ("Boolean Text.Text"), "BoolText.TextColor"=w2800) -> ()  [unwired: 2 in, 2 out]
        n1244 = local read "numberOfCommandLines"() -> (w2809:i32)
        n1245 = call "setCommandString.vi"("addLF_onlyIfNeeded? (T)"=TRUE, "addLF? (T)"=TRUE ("addLF?"), "addTimeAndChevron? (T)"=TRUE ("addTimeAndChevron?"), "numLines"=w2809, "stringToAdd"=w2803, "UI Data In"=w2799) -> ("UI Data Out"=w2802:T9, "outputCommandString"=w2808:string)  [unwired: 3 in, 1 out]
        n1246 = property on="cB_commandLog" class="Str"("Text.Text"=w2808, "Text.Scroll Position"=inf) -> ()  [unwired: 2 in, 2 out]
      }
      frame "plotData" {
        n1247 = Variant To Data(error in=w2833, type=dbl[] [] ("Spectrum by Pixels"), Variant=w2832) -> (data=w2828:dbl[], error out=w2826:errorcluster)
        n1248 = Unbundle By Name(w2830) -> ("Wavelengths"=w2829:dbl[])
        n1249 = Bundle("Wavelengths"=w2829, "Spectrum by Pixels"=w2828) -> (w2827:T29)  [unwired: 1 in]
        n1250 = local write "1DdataGraph"(w2827) -> ()
      }
      frame "savePlot" {
        n1251 = local read "usb2000p_intTime"() -> (w2840:u32)
        n1252 = Get Date/Time In Seconds() -> (seconds since 1Jan1904=w2845:timestamp)
        n1253 = Format Into String(w2840) -> (resulting string=w2838:string)  [unwired: 3 in, 1 out]
        n1254 = Format Date/Time String(time format string (%c)="%Y%m%d_%H%M%S", seconds (now)=w2845) -> (date/time string=w2847:string)  [unwired: 1 in]
        n1255 = Concatenate Strings("spectra_" ("default name"), w2838, "ms_" ("string"), w2847, ".h5" ("default name")) -> (w2849:string)
        n1256 = local write "usb2000p_saveSpectra"(FALSE ("usb2000p_saveSpectra")) -> ()
        n1257 = call "File Dialog2"("prompt"="Select a file to save the data to.", "default name"=w2849, "pattern (all files)"="*.txt", "pattern label"="Text file") -> ("selected path"=w2835:path, "cancelled"=w2842:bool, "error out"=w2851:errorcluster)  [unwired: 8 in, 1 out]
        n1258 = Unbundle(w2851) -> ("status"=w2841:bool)  [unwired: 2 out]
        n1259 = Or(x=w2842, y=w2841) -> (x .or. y?=w2836:bool)
        n1260 = case shown="False" w2836 {
          tunnel: w2835 -> [w2855 _]
          frame False {
            n1261 = local read "1DdataGraph"() -> (w2861:cluster{dbl[], dbl[]})
            n1262 = Unbundle(w2861) -> (w2860:dbl[], w2859:dbl[])
            n1263 = Build Array(w2860, w2859) -> (w2858:dbl[][])
            n1264 = call-poly <vilib>:"Write Delimited Spreadsheet.vi"("file path (dialog if empty)"=w2855, "format (%.3f)"="%.6f", "2D data"=w2858, "transpose? (F)"=TRUE, "delimiter (\\t)"="," ("delimiter (\\t)")) -> ()  [unwired: 9 in, 2 out]
          }
          frame True {
          }
        }
      }
      frame "messageFromEquipLoop" {
        n1265 = Variant To Data(error in=w2874, type="", Variant=w2873) -> (data=w2862:string, error out=w2871:errorcluster)
        n1266 = local read "numberOfCommandLines"() -> (w2865:i32)
        n1267 = call "setCommandString.vi"("addLF_onlyIfNeeded? (T)"=TRUE, "addLF? (T)"=TRUE ("addLF?"), "addTimeAndChevron? (T)"=TRUE ("addTimeAndChevron?"), "numLines"=w2865, "stringToAdd"=w2862, "UI Data In"=w2864) -> ("UI Data Out"=w2863:T9, "outputCommandString"=w2866:string)  [unwired: 3 in, 1 out]
        n1268 = property on="cB_commandLog" class="Str"("Text.Text"=w2866, "Text.Scroll Position"=inf) -> ()  [unwired: 2 in, 2 out]
      }
      frame "testSomething" {
      }
      frame "Error" {
        # "#CodeRecommended - If you ever change the name of this \"Error\" message, you'll need to update the name in the Check Loop Error.vi as well."
        # "#CodeRecommended - Consider creating a system for logging errors in some way. These errors are for notification purposes only. Handling of specific errors should be performed in the message frames that generated the error."
        # "Error - Display an error dialog. This message is sent by the \"Error Handler\" VIs at the end of other loops in this application."
        n1269 = Variant To Data(error in=w2883, type=errorcluster {"status"=FALSE, "code"=0, "source"=""} ("error constant"), Variant=w2881) -> (data=w2879:errorcluster, error out=w2878:errorcluster)
        n1270 = call <vilib>:"Simple Error Handler.vi"("error in (no error)"=w2879) -> ()  [unwired: 4 in, 5 out]
        n1271 = Merge Errors(w2878) -> (w2877:errorcluster)
      }
      frame "Confirm Quit" {
        # "#CodeNeeded - \n\nIf there is data that has not been saved perhaps you should ask for confermation. \n\nalso when i add in the other devices i need to be able to check to see if they are disconnected or not."
        # "Confirm Quit - Determin if an instrument is still connected, and if one is, then put up a message that can confirm whether or not the user wants to exit the application. If they do want to quit, the disconnect from the instruments"
        n1272 = Unbundle By Name(w2893) -> ("pBotConnected?"=w2885:bool, "connectedInstruments"=w2888:T7[])
        n1273 = Array Size(array=w2888) -> (size(s)=w2887:i32)
        n1274 = Not Equal To 0?(x=w2887) -> (x != 0?=w2884:bool)
        n1275 = Or(x=w2885, y=w2884) -> (x .or. y?=w2886:bool)
        n1276 = case shown="True" w2886 {
          tunnel: w2892 -> [w2897 w2905]
          tunnel: w2890 -> [w2896 w2904]
          tunnel: w2891 -> [w2895 w2903]
          tunnel: [w2894 w2902] -> w2889
          frame False {
            w2899 = "Exit" ("Message")
            w2900 = TRUE ("Priority Message? (F)")
            # "no devices connected - quit"
            n1277 = call-poly "Enqueue Message.vi"("Priority Message? (F)"=w2900, "error in (no error)"=w2895, "Message"=w2899, "Message Queue"=w2896) -> ("error out"=w2901:errorcluster)  [unwired: 6 in, 1 out]
            n1278 = call-poly "Enqueue Message.vi"("Priority Message? (F)"=w2900, "error in (no error)"=w2895, "Message"=w2899, "Message Queue"=w2897) -> ("error out"=w2898:errorcluster)  [unwired: 6 in, 1 out]
            n1279 = Merge Errors(w2901, w2898) -> (w2894:errorcluster)
          }
          frame True {
            n1280 = Two Button Dialog(message="Warning! A device is still connected. Do you want to Quit anyway?", 1:"Don't quit" ("F button name (\"Cancel\")"), 2:"Quit" ("T button name (\"OK\")")) -> (T button?=w2906:bool)
            n1281 = case shown="True" w2906 {
              tunnel: w2905 -> [_ w2913]
              tunnel: w2904 -> [_ w2914]
              tunnel: w2903 -> [w2910 w2912]
              tunnel: [w2910 w2911] -> w2902
              frame False {
              }
              frame True {
                w2916 = "Exit" ("Message")
                w2917 = TRUE ("Priority Message? (F)")
                n1282 = call-poly "Enqueue Message.vi"("Priority Message? (F)"=w2917, "error in (no error)"=w2912, "Message"=w2916, "Message Queue"=w2914) -> ("error out"=w2918:errorcluster)  [unwired: 6 in, 1 out]
                n1283 = call-poly "Enqueue Message.vi"("Priority Message? (F)"=w2917, "error in (no error)"=w2912, "Message"=w2916, "Message Queue"=w2913) -> ("error out"=w2915:errorcluster)  [unwired: 6 in, 1 out]
                n1284 = Merge Errors(w2918, w2915) -> (w2911:errorcluster)
              }
            }
          }
        }
      }
      frame "Exit" {
        # "Stop the VI"
        # "Release the message queue reference"
        # "#CodeNeeded - Add any required cleanup code here. Note that if 'Exit' was called as a result of an error, an error dialog will be displayed. Add any custom error handling for an 'Exit' condition here as well."
        # "Exit - Exit the application."
        n1285 = Variant To Data(type=errorcluster {"status"=FALSE, "code"=0, "source"=""} ("error constant"), Variant=w2919) -> (data=w2920:errorcluster)  [unwired: 1 in, 1 out]
        n1286 = call <vilib>:"Simple Error Handler.vi"("error in (no error)"=w2920) -> ()  [unwired: 4 in, 5 out]
        n1287 = call "Fire User Event - Stop.vi"("User Event - Stop"=w2924) -> ("error out"=w2923:errorcluster)  [unwired: 10 in]
        n1288 = Release Queue(queue=w2929, error in (no error)=w2922) -> (error out=w2926:errorcluster)  [unwired: 1 in, 2 out]
        n1289 = Merge Errors(w2923, w2926) -> (w2925:errorcluster)
      }
      frame Default {
        # "'Default' case only runs if there is a message that isn't defined in any of the other cases.  Output a programming error."
        n1290 = xnode "Error Ring"("parameter 0"=w2930) -> ("error out"=w2931:errorcluster)
      }
    }
    n1291 = call "Error Handler - Message Handling Loop.vi"("error in (no error)"=w1197, "Message Queue"=w1199) -> ("dup error in"=w1198:errorcluster)  [unwired: 8 in, 1 out]
  }
  n1292 = Unregister For Events(event registration refnum=w15, error in=w12) -> (error out=w16:errorcluster)
  n1293 = Merge Errors(w16, w5, w6) -> (w17:errorcluster)
  n1294 = call "Destroy User Event - Stop.vi"("error in (no error)"=w17, "User Event - Stop"=w10) -> ("error out"=w13:errorcluster)  [unwired: 9 in]
  n1295 = disable-structure shown="RUN_TIME_ENGINE==True" {
    disable-tunnel: w13 -> [_ _]
    frame condition #0 (active) {
    }
    frame condition #1 {
      # "Call Quit LabVIEW if running as a built application."
      n1296 = Quit LabVIEW() -> ()  [unwired: 1 in]
    }
  }
  "textColorGreen" <- u32 9174826 ("textColorGreen")
  "textColorRed" <- u32 16750216 ("textColorRed")
  "textColorGray" <- u32 9868950 ("textColorGray")
